vi "Test DQMH modules.vi"() -> ()   [LabVIEW 2018, in "Application.lvlib"]
uses:
  Application.lvlib
  eMIC response.ctl
  DRV stand.ctl
  type defs/HW config.ctl
  eMICs Cluster.ctl
  SubVIs/App state data.ctl
  SubVIs/Trigger cluster.ctl
  type defs/DMM all config cluster.ctl
  type defs/DMM config cluster.ctl
  SubVIs/FGV DRV data.ctl
  SubVIs/DUT data Mode.ctl
  Instrument Drivers/LV_driver_MBrelay/type defs/FGV enum.ctl
  SubVIs/Step data.ctl
  <vilib>/ErrorRing/Error Ring.xnode
  Switches Module/MB switches Module.lvlib
  MB 01 switches Module/MB 01 switches Module.lvlib
  DMM Module/DMM Module.lvlib
  v2_CE14/CE14_v2.lvlib
  Instrument Drivers/LV_driver_MBrelay/MB Relay.lvlib
panel:
  out "Name":string
  out "SAP ID":string
  out "Progress":string
  out "DRV stand":T1
  in  "Auto/Man":bool
  out "DC Measure Completed":bool
  in  "Test Channel 10":bool
  in  "Test Channel 9":bool
  in  "Test Channel 8":bool
  in  "Test Channel 7":bool
  in  "Test Channel 6":bool
  in  "Test Channel 5":bool
  in  "Test Channel 4":bool
  in  "Test Channel 3":bool
  in  "Test Channel 2":bool
  in  "Test Channel 1":bool
  in  "Shorted Circuits Test":bool
  out "CE14  Module did it":bool[](array[boolean])
  out "time elased(ms)":u32
  out "Inst. 9":bool
  in  "Exit":bool
  out "Inst. 8":bool
  out "Inst. 7":bool
  out "Inst. 6":bool
  out "Inst. 5":bool
  out "Inst. 4":bool
  out "Inst. 3":bool
  out "Inst. 2":bool
  out "Inst. 1":bool
  out "new Trigger?":bool
  out "last Trigger?":bool
  out "error out":errorcluster
  out "State log":string
  out "AC Measure  Completed":bool
  in  "Select CE14 eMIC Module Instance":i32(ring)=-1 items=["All"=-1, "1"=1, "2"=2, "3"=3, "4"=4, "5"=5, "6"=6]
  out "New board?":bool
  in  "Test":bool caption="Again"
  out "DRV 61":u32(colorbox)
  in  "Settings":bool
  in  "Again":bool
  out "DRV 60":u32(colorbox) caption="60"
  out "DRV 59":u32(colorbox) caption="59"
  out "DRV 58":u32(colorbox) caption="58"
  out "DRV 57":u32(colorbox) caption="57"
  out "DRV 56":u32(colorbox) caption="56"
  out "DRV 55":u32(colorbox) caption="55"
  out "DRV 54":u32(colorbox) caption="54"
  out "DRV 53":u32(colorbox) caption="53"
  out "DRV 52":u32(colorbox) caption="52"
  out "DRV 51":u32(colorbox) caption="51"
  out "DRV 50":u32(colorbox) caption="50"
  out "DRV 49":u32(colorbox) caption="49"
  out "DRV 48":u32(colorbox) caption="48"
  out "DRV 47":u32(colorbox) caption="47"
  out "DRV 46":u32(colorbox) caption="46"
  out "DRV 45":u32(colorbox) caption="45"
  out "DRV 44":u32(colorbox) caption="44"
  out "DRV 43":u32(colorbox) caption="43"
  out "DRV 42":u32(colorbox) caption="42"
  out "DRV 41":u32(colorbox) caption="41"
  out "DRV 40":u32(colorbox) caption="40"
  out "DRV 39":u32(colorbox) caption="39"
  out "DRV 38":u32(colorbox) caption="38"
  out "DRV 37":u32(colorbox) caption="37"
  out "DRV 36":u32(colorbox) caption="36"
  out "DRV 35":u32(colorbox) caption="35"
  out "DRV 34":u32(colorbox) caption="34"
  out "DRV 33":u32(colorbox) caption="33"
  out "DRV 32":u32(colorbox) caption="32"
  out "DRV 31":u32(colorbox) caption="31"
  out "DRV 30":u32(colorbox) caption="30"
  out "DRV 29":u32(colorbox) caption="29"
  out "DRV 28":u32(colorbox) caption="28"
  out "DRV 27":u32(colorbox) caption="27"
  out "DRV 26":u32(colorbox) caption="26"
  out "DRV 25":u32(colorbox) caption="25"
  out "DRV 24":u32(colorbox) caption="24"
  out "DRV 23":u32(colorbox) caption="23"
  out "DRV 22":u32(colorbox) caption="22"
  out "DRV 21":u32(colorbox) caption="21"
  out "DRV 20":u32(colorbox) caption="20"
  out "DRV 19":u32(colorbox)=4375612 caption="19"
  out "DRV 18":u32(colorbox) caption="18"
  out "DRV 17":u32(colorbox) caption="17"
  out "DRV 16":u32(colorbox) caption="16"
  out "DRV 15":u32(colorbox) caption="15"
  out "DRV 14":u32(colorbox) caption="14"
  out "DRV 13":u32(colorbox)=4375612 caption="13"
  out "DRV 12":u32(colorbox) caption="12"
  out "DRV 11":u32(colorbox) caption="11"
  out "DRV 10":u32(colorbox) caption="10"
  out "DRV 9":u32(colorbox) caption="9"
  out "DRV 8":u32(colorbox) caption="8"
  out "DRV 7":u32(colorbox)=4375612 caption="7"
  out "DRV 6":u32(colorbox) caption="6"
  out "DRV 5":u32(colorbox) caption="5"
  out "DRV 4":u32(colorbox) caption="4"
  out "DRV 3":u32(colorbox) caption="3"
  out "DRV 2":u32(colorbox) caption="2"
  out "DRV 1":u32(colorbox)=13224393 caption="1"
  out "version":string caption="Version"
  out "Module ID":i32
  in  "Tab Control":T2(tab)
  out "Short DRV":bool[][](array[boolean])
  in  "Mux 10-1":bool
  in  "mux 6-1":bool
  in  "Read Optos":bool
  in  "DMM select Current Input":bool
  in  "mux2-1(DMM I) encode":enum16{"DMM I (0.5)", "DMM I (12)"}(ring)
  in  "mux 6-1 data":T3(ring)
  in  "mux 10-1 data":T4(ring)
  out "trigger Value":bool
  in  "Read trigger":bool
  in  "Reset JIG":bool
  in  "eMIC":bool
  in  "DEMUX 1-10":bool
  in  "TurnON/OFF +5V":bool
  in  "5V Value":bool
  in  "demux1_10(x6)_encode":T5(ring)
  in  "eMIC 6 values":bool[](array[boolean])=[FALSE, FALSE, FALSE, FALSE, FALSE, FALSE]
  in  "config DMM input":bool
  in  "connect DMM":bool
  in  "DMM read dual value":bool
  in  "config DMM":bool
  in  "Detector Rate":u8(ring)=2 items=["SLOW", "MID", "FAST"]
  in  "DCI range":dbl=0.5
  in  "DCV range":dbl=1000.0
  out "DCV(Volts)":dbl
  out "DCI(mA)":dbl
  in  "request AC":bool
  in  "Open COM eMIC":bool
  in  "check connected":bool
  out "eMIC 1":T6
  out "eMIC 2":T6
  out "eMIC 3":T6
  out "eMIC 4":T6
  out "eMIC 5":T6
  out "eMIC 6":T6
  out "EMIC connected":bool[](array[boolean])
  out "AC switches Module":bool
  out "DC Measure Module":bool
  out "DC Switches Module":bool
  out "AC Measure Module":bool
  # "HV-60D: LED POWER DRIVER ON-LINE TESTER"
  # "60"
  # "6"
  # "12"
  # "18"
  # "24"
  # "30"
  # "36"
  # "42"
  # "48"
  # "54"
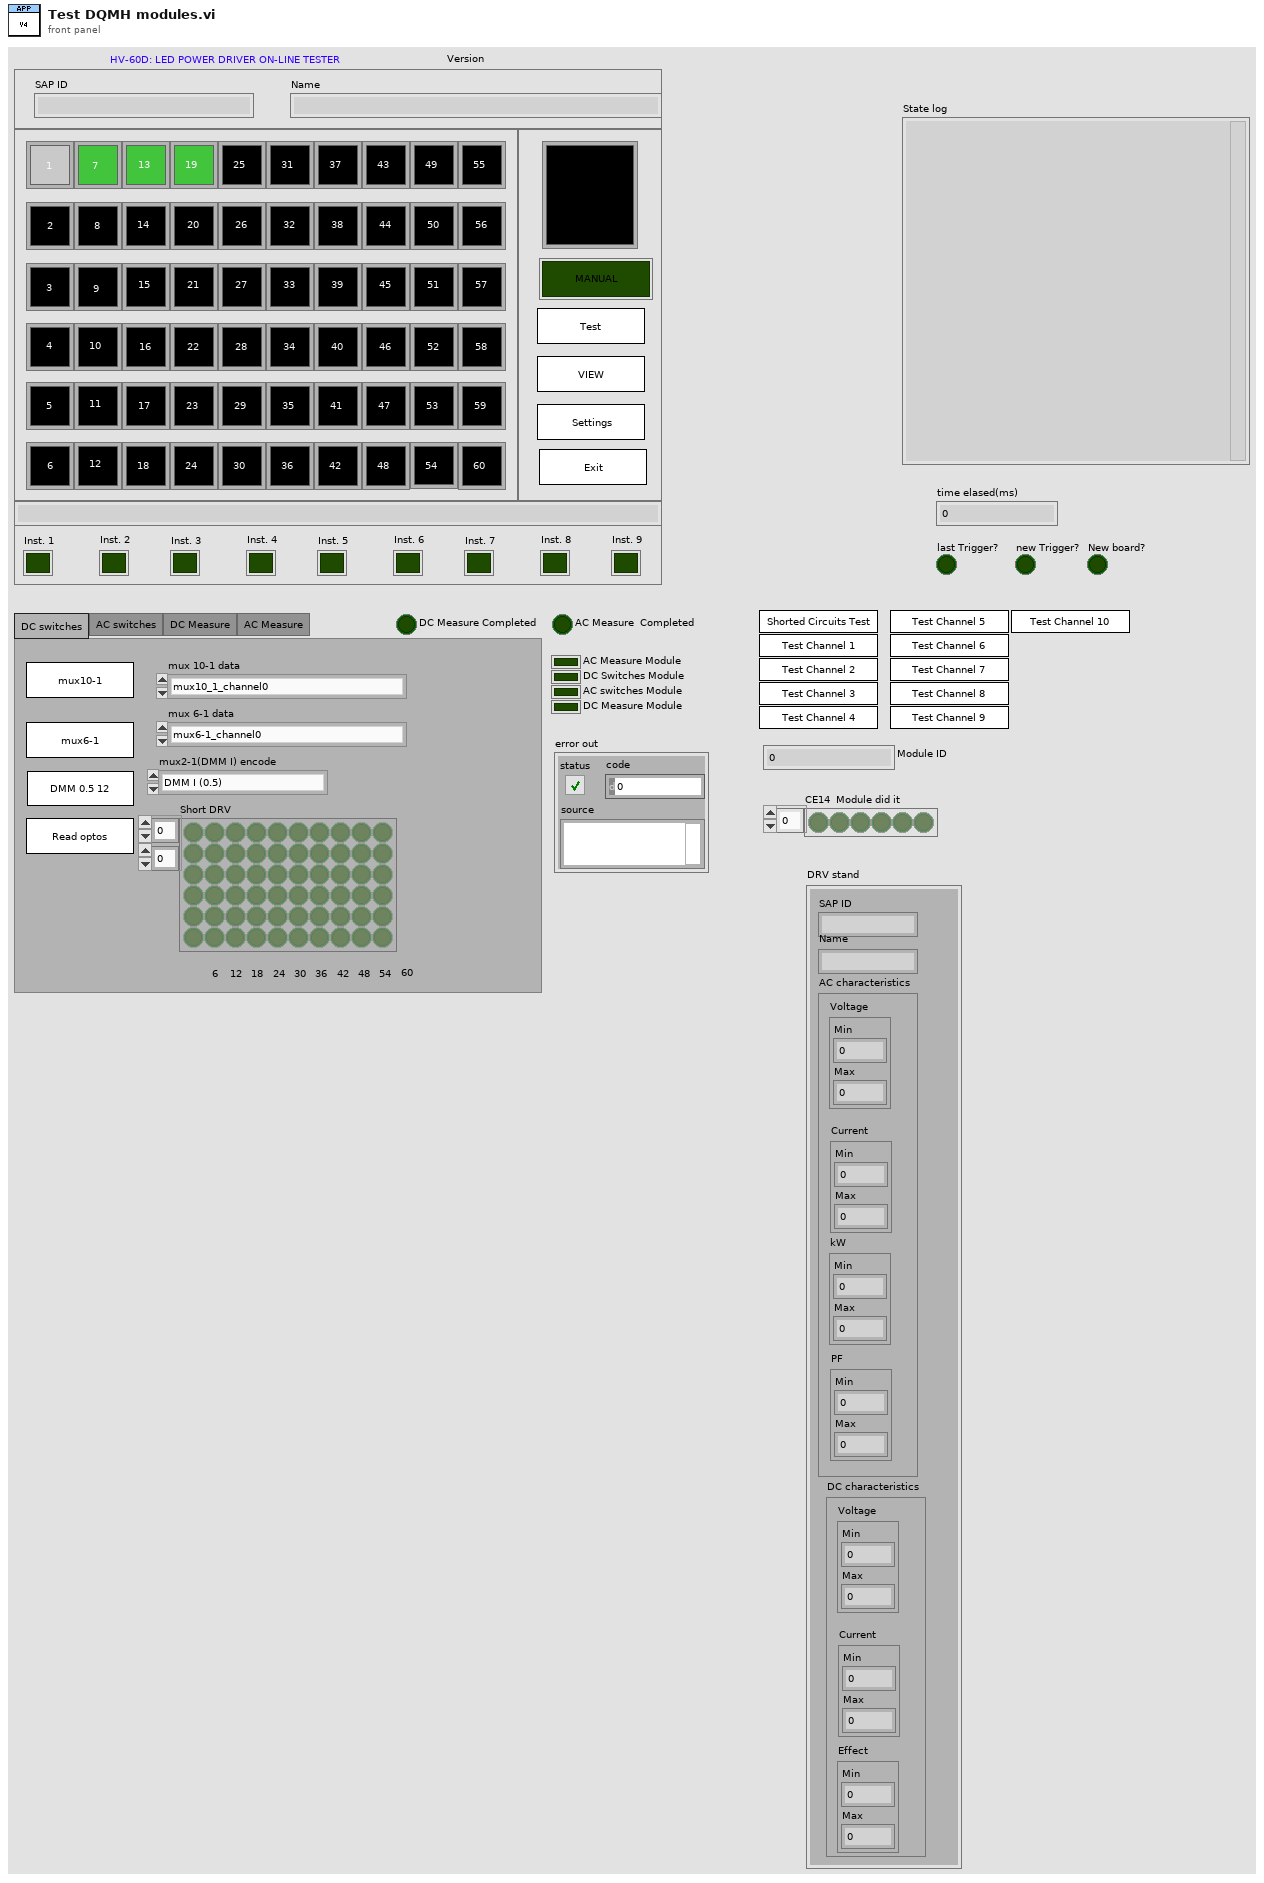
[diagram p1: front panel]
types:
  T1 = typedef "Application.lvlib/DRV stand.ctl" = cluster{"SAP ID":string, "Name":string, "AC characteristics":cluster{"Voltage":cluster{"Min":dbl, "Max":dbl}, "Current":cluster{"Min":dbl, "Max":dbl}, "kW":cluster{"Min":dbl, "Max":dbl}, "PF":cluster{"Min":dbl, "Max":dbl}}, "DC characteristics":cluster{"Voltage":cluster{"Min":dbl, "Max":dbl}, "Current":cluster{"Min":dbl, "Max":dbl}, "Effect":cluster{"Min":dbl, "Max":dbl}}}
  T2 = enum32{"DC switches", "AC switches", "DC Measure", "AC Measure"}
  T3 = enum16{"mux6-1_channel0", "mux6_1_channel1_0", "mux6_1_channel1_1", "mux6-1_channel1_2", "mux6_1_channel1_3", "mux6_1_channel2_0", "mux6_1_channel2_1", "mux6_1_channel2_2", "mux6_1_channel2_3", "mux6_1_channel3_0", "mux6_1_channel3_1", "mux6_1_channel3_2", "mux6_1_channel3_3", "mux6_1_channel4_0", "mux6_1_channel4_1", "mux6_1_channel4_2", "mux6_1_channel4_3", "mux6_1_channel5_0", "mux6_1_channel5_1", "mux6_1_channel5_2", "mux6_1_channel5_3", "mux6_1_channel6_0", "mux6_1_channel6_1", "mux6_1_channel6_2", "mux6_1_channel6_3"}
  T4 = enum16{"mux10_1_channel0", "mux10_1_channel1", "mux10_1_channel2", "mux10_1_channel3", "mux10_1_channel4", "mux10_1_channel5", "mux10_1_channel6", "mux10_1_channel7", "mux10_1_channel8", "mux10_1_channel9", "mux10_1_channel10"}
  T5 = enum16{"demux1_10_channel0", "demux1_10_channel1", "demux1_10_channel2", "demux1_10_channel3", "demux1_10_channel4", "demux1_10_channel5", "demux1_10_channel6", "demux1_10_channel7", "demux1_10_channel8", "demux1_10_channel9", "demux1_10_channel10"}
  T6 = typedef "Application.lvlib/eMIC response.ctl" = cluster{"ACV":dbl, "ACI":dbl, "pF":dbl, "kW":dbl, "Freq":dbl}
  T7 = typedef "Application.lvlib/eMICs Cluster.ctl" = cluster{"eMIC 1":T6, "eMIC 2":T6, "eMIC 3":T6, "eMIC 4":T6, "eMIC 5":T6, "eMIC 6":T6}
  T8 = typedef "Application.lvlib/HW config.ctl" = cluster{"DMM":string, "mux":string, "demux":string, "eMIC1":string, "eMIC2":string, "eMIC3":string, "eMIC4":string, "eMIC5":string, "eMIC6":string}
  T9 = typedef "Application.lvlib/Trigger cluster.ctl" = cluster{"new board?":bool, "new trigger":bool, "last trigger":bool}
  T10 = typedef "Application.lvlib/App state data.ctl" = cluster{"command":string, "command data":variant}
  T11 = typedef "CE14_v2.lvlib/Broadcast Events--cluster.ctl" = cluster{"Module Did Init":refnum<user-event>, "Status Updated":refnum<user-event>, "Error Reported":refnum<user-event>, "Module Did Stop":refnum<user-event>, "Update Module Execution Status":refnum<user-event>, "CE14 response data":refnum<user-event>}
  T12 = typedef "MB switches Module.lvlib/Broadcast Events--cluster.ctl" = cluster{"Module Did Init":refnum<user-event>, "Status Updated":refnum<user-event>, "Error Reported":refnum<user-event>, "Module Did Stop":refnum<user-event>, "Update Module Execution Status":refnum<user-event>}
  T13 = typedef "MB 01 switches Module.lvlib/Broadcast Events--cluster.ctl" = cluster{"Module Did Init":refnum<user-event>, "Status Updated":refnum<user-event>, "Error Reported":refnum<user-event>, "Module Did Stop":refnum<user-event>, "Update Module Execution Status":refnum<user-event>}
  T14 = typedef "DMM Module.lvlib/Broadcast Events--cluster.ctl" = cluster{"Module Did Init":refnum<user-event>, "Status Updated":refnum<user-event>, "Error Reported":refnum<user-event>, "Module Did Stop":refnum<user-event>, "Update Module Execution Status":refnum<user-event>}
  T15 = enum32{"Invalid", "Standard", "Closed", "Hidden", "Minimized", "Maximized"}
  T16 = typedef "Application.lvlib/DMM all config cluster.ctl" = cluster{"DMM config cluster":T17, "mux2-1(DMM I) encode":enum16{"DMM I (0.5)", "DMM I (12)"}}
  T17 = typedef "Application.lvlib/DMM config cluster.ctl" = cluster{"DCV range":dbl, "DCI range":dbl, "Detector Rate":u8}
  T18 = typedef "Application.lvlib/DUT data Mode.ctl" = enum16{"range Limit", "Short Circuits", "AC parameter", "DC parameter"}
  T19 = typedef "Application.lvlib/FGV DRV data.ctl" = enum16{"Init", "Write", "Read", "Process"}
  T20 = typedef "MB Relay.lvlib/FGV enum.ctl" = enum16{"Write", "Init FGV", "Read", "All OFF", "All ON"}
  T21 = typedef "CE14_eMIC.lvlib/CE14.data.ctl" = cluster{"string":string, "float":dbl, "Name":string}
  T22 = typedef "Application.lvlib/DRV cluster 2.ctl" = cluster{"Shorted Circuit":bool, "AC voltage(volts)":dbl, "AC Current (mA)":dbl, "AC kW (W)":dbl, "AC pF ":dbl, "DC Voltage (Volts)":dbl, "DC Current (mA)":dbl, "DC kW (W)":dbl, "DRV Fail/Pass (T)":bool}
  T23 = typedef "Application.lvlib/Step data.ctl" = cluster{"command":string, "Data":variant}
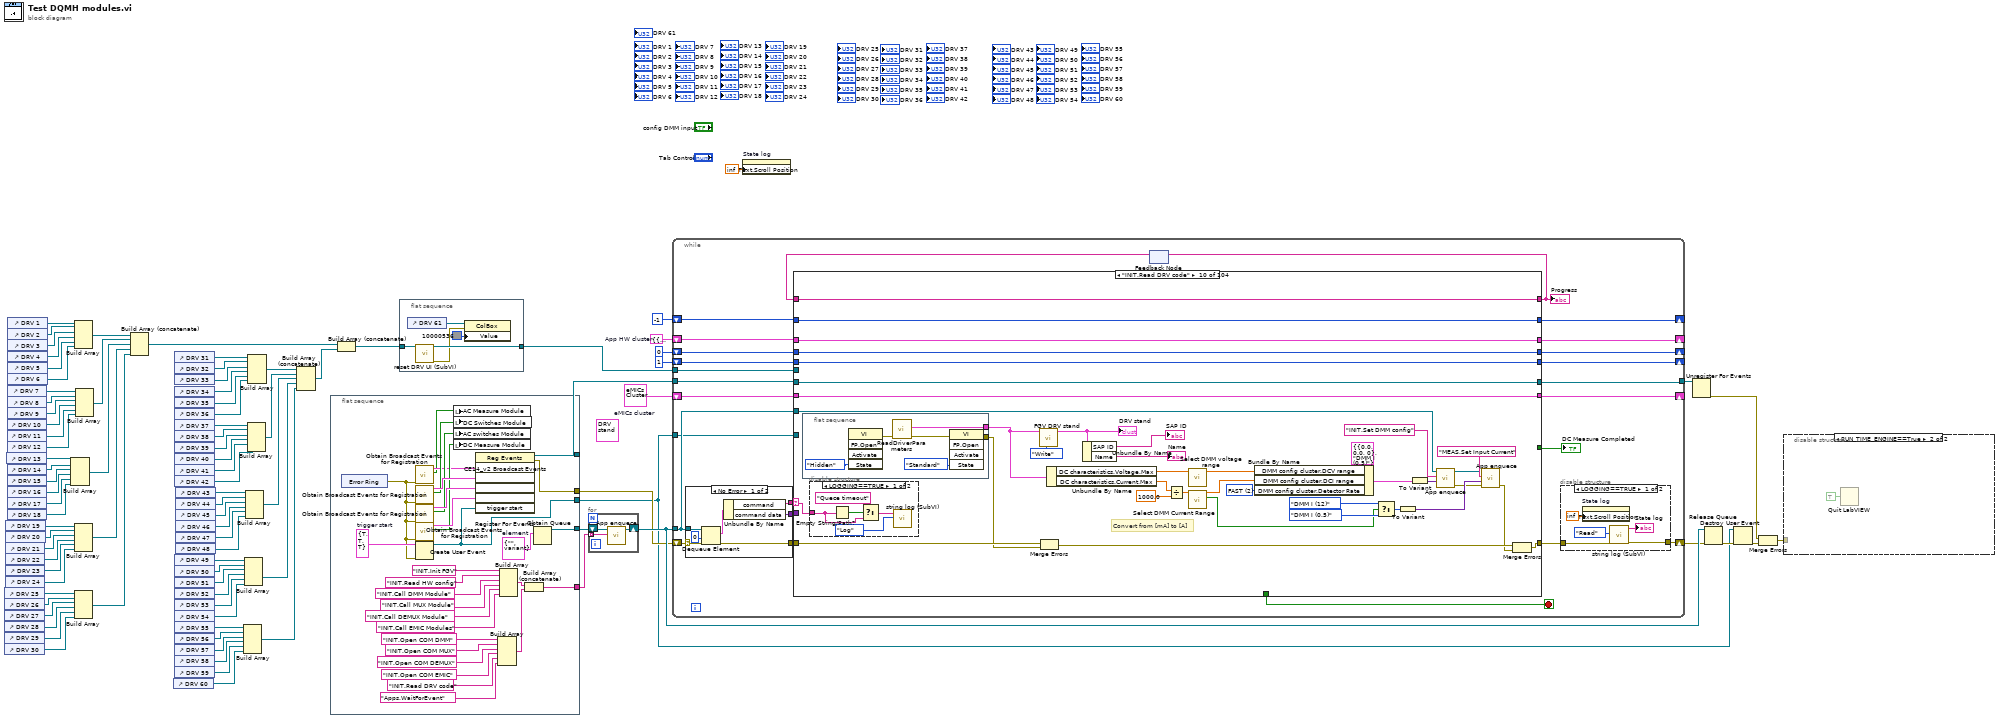
[diagram p0: block diagram]
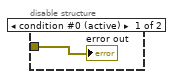
[diagram p2: hidden frame]
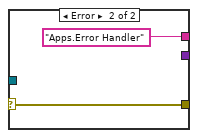
[diagram p4: hidden frame]
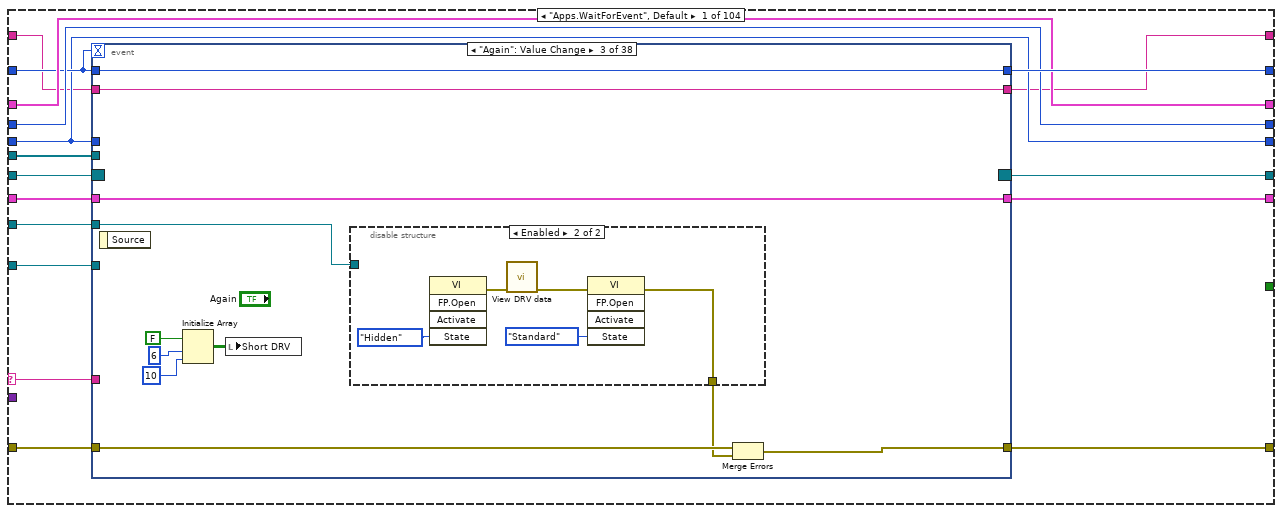
[diagram p5: hidden frame]
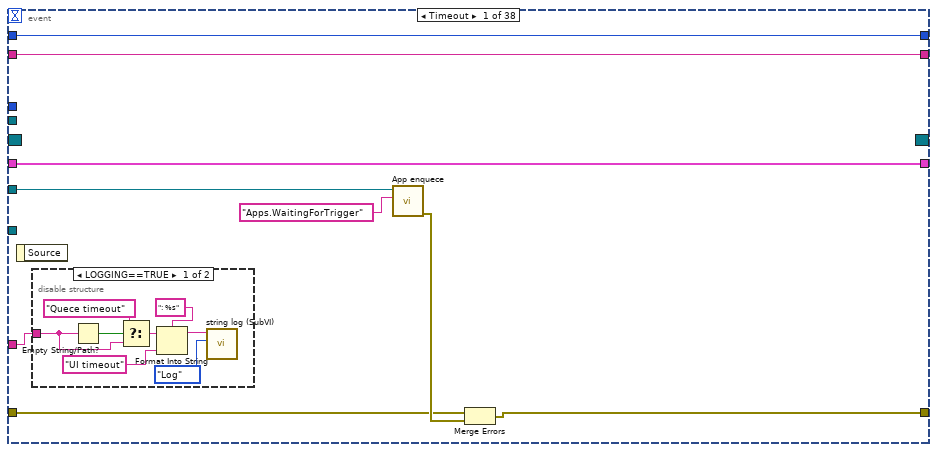
[diagram p6: hidden frame]
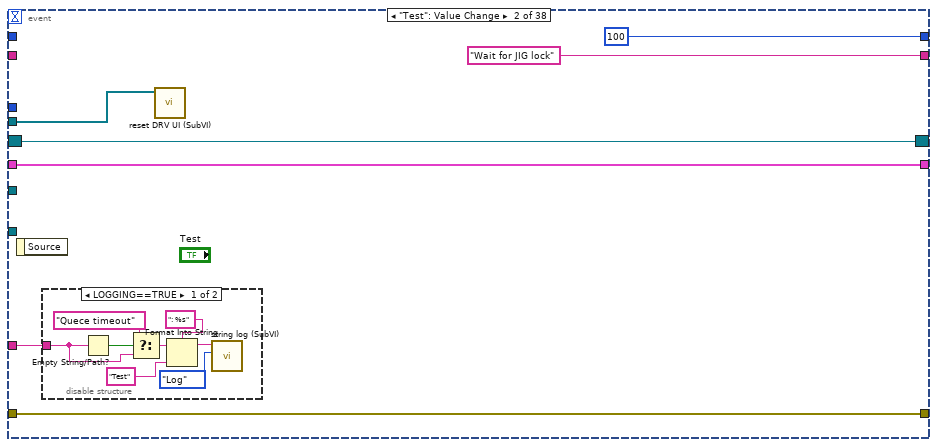
[diagram p8: hidden frame]
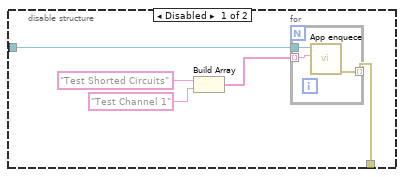
[diagram p10: hidden frame]
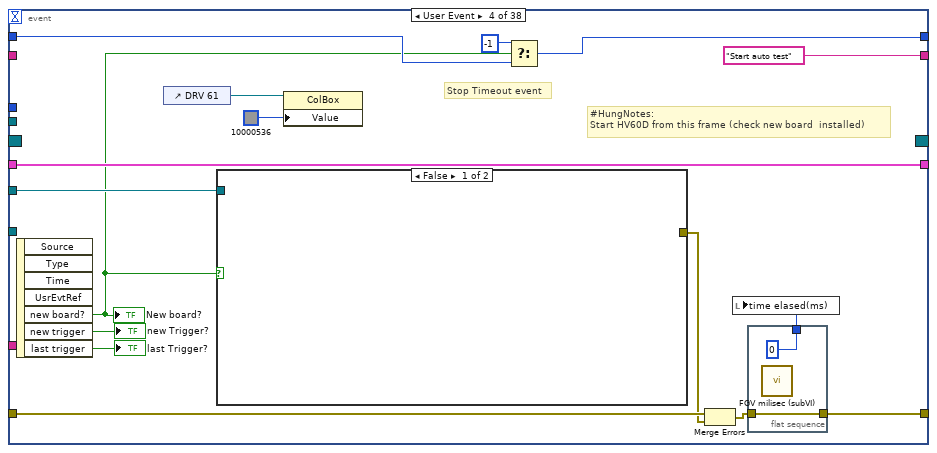
[diagram p11: hidden frame]
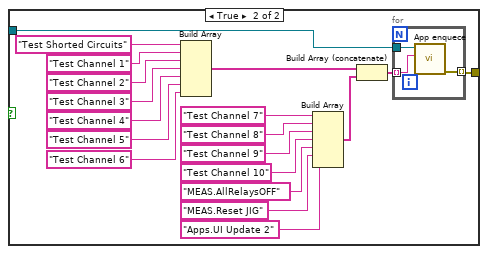
[diagram p12: hidden frame]
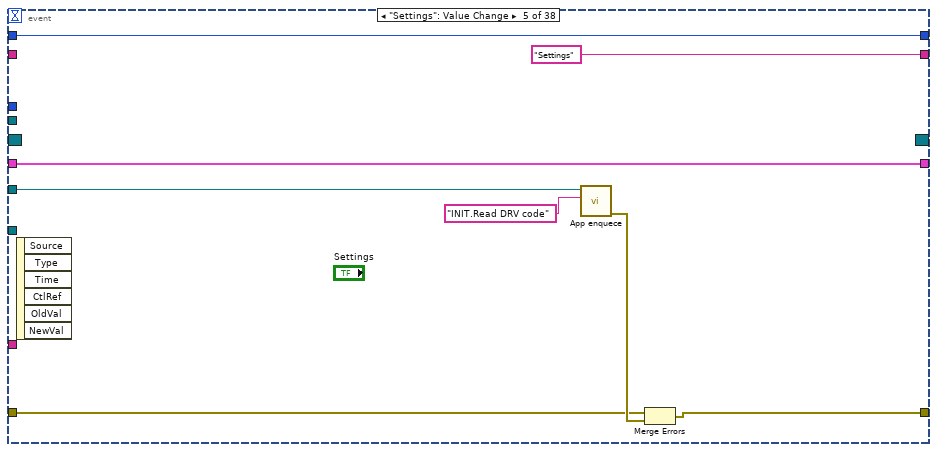
[diagram p13: hidden frame]
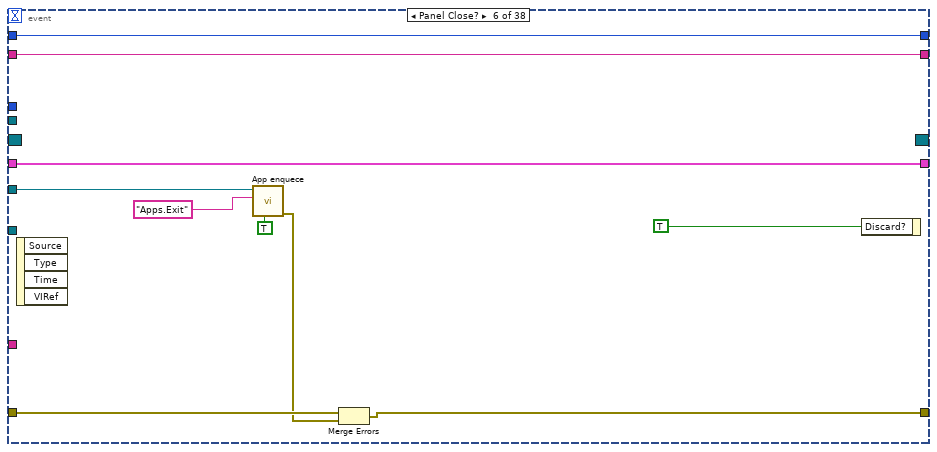
[diagram p14: hidden frame]
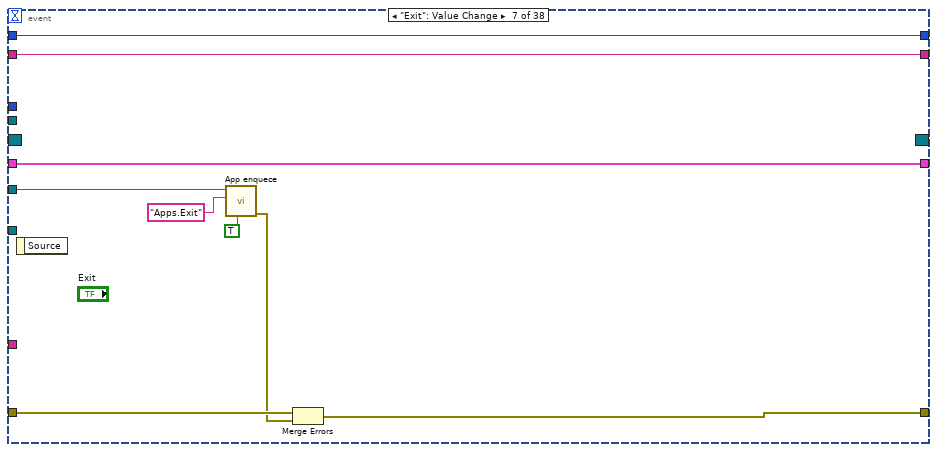
[diagram p15: hidden frame]
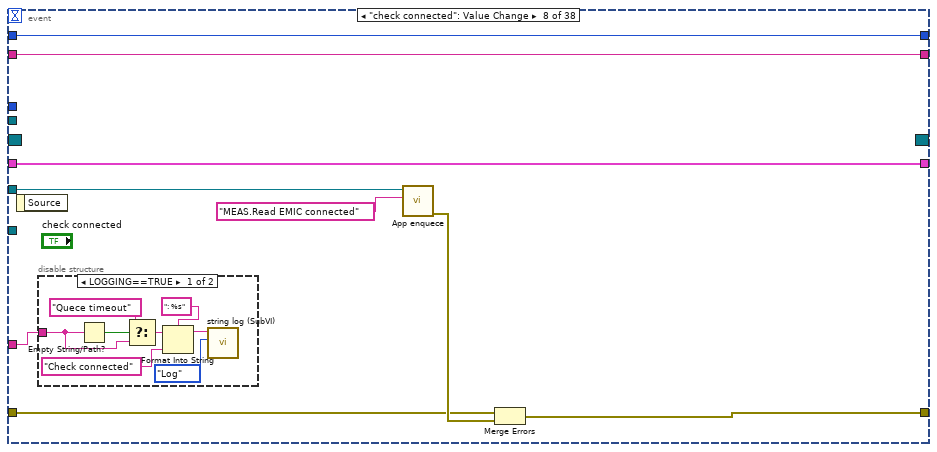
[diagram p16: hidden frame]
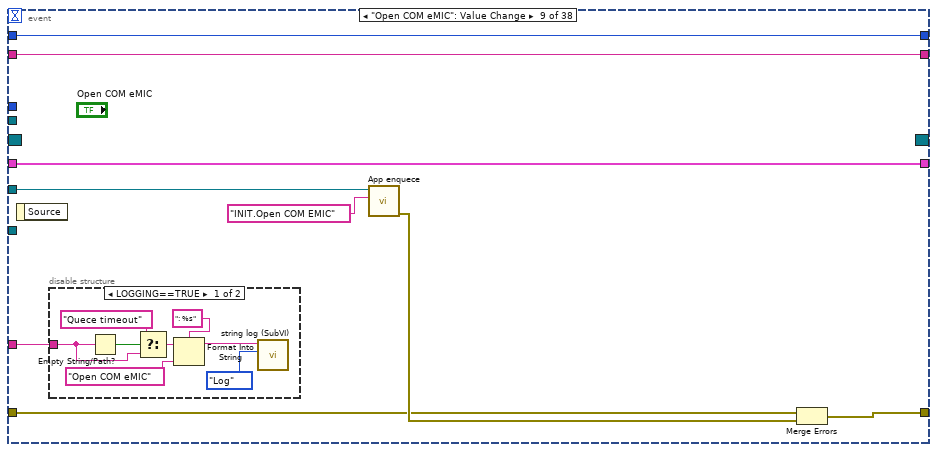
[diagram p18: hidden frame]
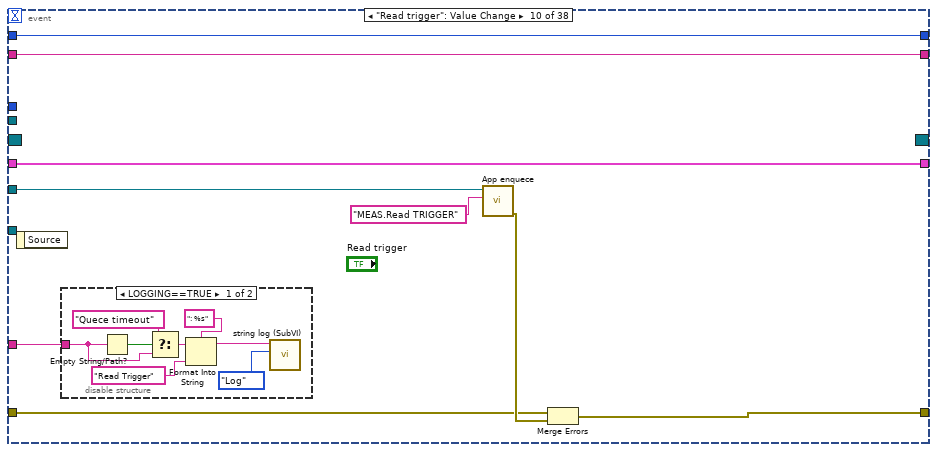
[diagram p20: hidden frame]
diagram:
  (unwired) T1 {"SAP ID"="", "Name"="", "AC characteristics"={"Voltage"={"Min"=0.0, "Max"=0.0}, "Current"={"Min"=0.0, "Max"=0.0}, "kW"={"Min"=0.0, "Max"=0.0}, "PF"={"Min"=0.0, "Max"=0.0}}, "DC characteristics"={"Voltage"={"Min"=0.0, "Max"=0.0}, "Current"={"Min"=0.0, "Max"=0.0}, "Effect"={"Min"=0.0, "Max"=0.0}}} ("DRV stand")
  w84 = T7 {"eMIC 1"={"ACV"=0.0, "ACI"=0.0, "pF"=0.0, "kW"=0.0, "Freq"=0.0}, "eMIC 2"={"ACV"=0.0, "ACI"=0.0, "pF"=0.0, "kW"=0.0, "Freq"=0.0}, "eMIC 3"={"ACV"=0.0, "ACI"=0.0, "pF"=0.0, "kW"=0.0, "Freq"=0.0}, "eMIC 4"={"ACV"=0.0, "ACI"=0.0, "pF"=0.0, "kW"=0.0, "Freq"=0.0}, "eMIC 5"={"ACV"=0.0, "ACI"=0.0, "pF"=0.0, "kW"=0.0, "Freq"=0.0}, "eMIC 6"={"ACV"=0.0, "ACI"=0.0, "pF"=0.0, "kW"=0.0, "Freq"=0.0}}  # eMICs cluster
  w89 = cluster{"HW config 2":T8} {"HW config 2"={"DMM"="COM15", "mux"="COM11", "demux"="COM16", "eMIC1"="COM13", "eMIC2"="COM6", "eMIC3"="COM9", "eMIC4"="COM10", "eMIC5"="COM12", "eMIC6"="COM11"}}  # App HW cluster
  n1 = control-ref of="DRV 25"() -> (w54:refnum<vi>)
  n2 = control-ref of="DRV 26"() -> (w55:refnum<vi>)
  n3 = control-ref of="DRV 27"() -> (w56:refnum<vi>)
  n4 = control-ref of="DRV 28"() -> (w57:refnum<vi>)
  n5 = control-ref of="DRV 29"() -> (w58:refnum<vi>)
  n6 = control-ref of="DRV 30"() -> (w59:refnum<vi>)
  n7 = control-ref of="DRV 21"() -> (w63:refnum<vi>)
  n8 = control-ref of="DRV 22"() -> (w62:refnum<vi>)
  n9 = control-ref of="DRV 23"() -> (w61:refnum<vi>)
  n10 = control-ref of="DRV 24"() -> (w60:refnum<vi>)
  n11 = control-ref of="DRV 19"() -> (w65:refnum<vi>)
  n12 = control-ref of="DRV 20"() -> (w64:refnum<vi>)
  n13 = control-ref of="DRV 13"() -> (w71:refnum<vi>)
  n14 = control-ref of="DRV 7"() -> (w77:refnum<vi>)
  n15 = control-ref of="DRV 8"() -> (w76:refnum<vi>)
  n16 = control-ref of="DRV 9"() -> (w75:refnum<vi>)
  n17 = control-ref of="DRV 10"() -> (w74:refnum<vi>)
  n18 = control-ref of="DRV 11"() -> (w73:refnum<vi>)
  n19 = control-ref of="DRV 12"() -> (w72:refnum<vi>)
  n20 = control-ref of="DRV 14"() -> (w70:refnum<vi>)
  n21 = control-ref of="DRV 15"() -> (w69:refnum<vi>)
  n22 = control-ref of="DRV 16"() -> (w68:refnum<vi>)
  n23 = control-ref of="DRV 17"() -> (w67:refnum<vi>)
  n24 = control-ref of="DRV 18"() -> (w66:refnum<vi>)
  n25 = control-ref of="DRV 1"() -> (w83:refnum<vi>)
  n26 = control-ref of="DRV 2"() -> (w82:refnum<vi>)
  n27 = control-ref of="DRV 3"() -> (w81:refnum<vi>)
  n28 = control-ref of="DRV 4"() -> (w80:refnum<vi>)
  n29 = control-ref of="DRV 5"() -> (w79:refnum<vi>)
  n30 = control-ref of="DRV 6"() -> (w78:refnum<vi>)
  n31 = Build Array(w71, w70, w69, w68, w67, w66) -> (w51:refnum<vi>[])
  n32 = Build Array(w83, w82, w81, w80, w79, w78) -> (w53:refnum<vi>[])
  n33 = Build Array(w65, w64, w63, w62, w61, w60) -> (w50:refnum<vi>[])
  n34 = Build Array(w54, w55, w56, w57, w58, w59) -> (w49:refnum<vi>[])
  n35 = Build Array(w77, w76, w75, w74, w73, w72) -> (w52:refnum<vi>[])
  n36 = Build Array (concatenate)(w53, w52, w51, w50, w49) -> (w13:refnum<vi>[])
  n37 = control-ref of="DRV 60"() -> (w24:refnum<vi>)
  n38 = control-ref of="DRV 55"() -> (w19:refnum<vi>)
  n39 = control-ref of="DRV 56"() -> (w20:refnum<vi>)
  n40 = control-ref of="DRV 57"() -> (w21:refnum<vi>)
  n41 = control-ref of="DRV 58"() -> (w22:refnum<vi>)
  n42 = control-ref of="DRV 59"() -> (w23:refnum<vi>)
  n43 = control-ref of="DRV 31"() -> (w43:refnum<vi>)
  n44 = control-ref of="DRV 32"() -> (w44:refnum<vi>)
  n45 = control-ref of="DRV 33"() -> (w45:refnum<vi>)
  n46 = control-ref of="DRV 34"() -> (w46:refnum<vi>)
  n47 = control-ref of="DRV 35"() -> (w47:refnum<vi>)
  n48 = control-ref of="DRV 36"() -> (w48:refnum<vi>)
  n49 = control-ref of="DRV 37"() -> (w42:refnum<vi>)
  n50 = control-ref of="DRV 38"() -> (w41:refnum<vi>)
  n51 = control-ref of="DRV 39"() -> (w40:refnum<vi>)
  n52 = control-ref of="DRV 40"() -> (w39:refnum<vi>)
  n53 = control-ref of="DRV 41"() -> (w38:refnum<vi>)
  n54 = control-ref of="DRV 42"() -> (w37:refnum<vi>)
  n55 = control-ref of="DRV 49"() -> (w30:refnum<vi>)
  n56 = control-ref of="DRV 50"() -> (w29:refnum<vi>)
  n57 = control-ref of="DRV 51"() -> (w28:refnum<vi>)
  n58 = control-ref of="DRV 52"() -> (w27:refnum<vi>)
  n59 = control-ref of="DRV 53"() -> (w26:refnum<vi>)
  n60 = control-ref of="DRV 54"() -> (w25:refnum<vi>)
  n61 = control-ref of="DRV 43"() -> (w31:refnum<vi>)
  n62 = control-ref of="DRV 44"() -> (w32:refnum<vi>)
  n63 = control-ref of="DRV 45"() -> (w33:refnum<vi>)
  n64 = control-ref of="DRV 46"() -> (w34:refnum<vi>)
  n65 = control-ref of="DRV 47"() -> (w35:refnum<vi>)
  n66 = control-ref of="DRV 48"() -> (w36:refnum<vi>)
  n67 = Build Array(w19, w20, w21, w22, w23, w24) -> (w14:refnum<vi>[])
  n68 = Build Array(w30, w29, w28, w27, w26, w25) -> (w15:refnum<vi>[])
  n69 = Build Array(w31, w32, w33, w34, w35, w36) -> (w16:refnum<vi>[])
  n70 = Build Array(w42, w41, w40, w39, w38, w37) -> (w17:refnum<vi>[])
  n71 = Build Array(w43, w44, w45, w46, w47, w48) -> (w18:refnum<vi>[])
  n72 = Build Array (concatenate)(w18, w17, w16, w15, w14) -> (w12:refnum<vi>[])
  n73 = flat-sequence {
    tunnel: [w116] -> w91
    tunnel: [w115] -> w88
    tunnel: [w114] -> w87
    tunnel: [w113] -> w11
    tunnel: [w108] -> w3
    frame #0 {
      w109 = T9 {"new board?"=TRUE, "new trigger"=TRUE, "last trigger"=TRUE}  # trigger start
      w110 = T10 {"command"="", "command data"=variant}  # element
      n74 = xnode "Error Ring"() -> ("error out"=w107:errorcluster)
      n75 = call "Obtain Broadcast Events for Registration.vi"("error in (no error)"=w107) -> ("Already running?"=w111:bool, "CE14_v2 Broadcast Events"=w112:T11)  [unwired: 8 in, 1 out]
      n76 = call "Obtain Broadcast Events for Registration.vi"("error in (no error)"=w107) -> ("Already running?"=w119:bool, "Switches Module Broadcast Events"=w122:T12)  [unwired: 8 in, 1 out]
      n77 = call "Obtain Broadcast Events for Registration.vi"("error in (no error)"=w107) -> ("Already running?"=w118:bool, "MB 01 switches Module Broadcast Events"=w121:T13)  [unwired: 8 in, 1 out]
      n78 = call "Obtain Broadcast Events for Registration.vi"("error in (no error)"=w107) -> ("Already running?"=w117:bool, "DMM Module Broadcast Events"=w120:T14)  [unwired: 8 in, 1 out]
      n79 = Create User Event(user event datatype=w109, error in=w107) -> (user event=w108:refnum<user-event>)  [unwired: 1 out]
      n80 = local write "AC Measure Module"(w111) -> ()
      n81 = local write "DC Switches Module"(w119) -> ()
      n82 = local write "AC switches Module"(w118) -> ()
      n83 = local write "DC Measure Module"(w117) -> ()
      n84 = register-events(w112, w122, w121, w120, w108) -> (reference out=w116:refnum<event-registration>, error out=w113:errorcluster)  [unwired: 2 in]
      n85 = Build Array("INIT.Open COM DMM", "INIT.Open COM MUX", "INIT.Open COM DEMUX", "INIT.Open COM EMIC", "INIT.Read DRV code", "Apps.WaitForEvent") -> (w104:string[])
      n86 = Build Array("INIT.Init FGV", "INIT.Read HW config", "INIT.Call DMM Module", "INIT.Call MUX Module", "INIT.Call DEMUX Module", "INIT.Call EMIC Modules") -> (w105:string[])
      n87 = Build Array (concatenate)(w105, w104) -> (w114:string[])
      n88 = Obtain Queue(element data type=w110) -> (queue out=w115:refnum<queue>)  [unwired: 4 in, 2 out]
    }
  }
  n89 = Build Array (concatenate)(w13, w12) -> (w10:refnum<vi>[])
  n90 = flat-sequence {
    tunnel: w10 -> [w128]
    tunnel: [w127] -> w9
    frame #0 {
      n91 = control-ref of="DRV 61"() -> (w124:refnum<vi>)
      n92 = call "reset DRV UI (SubVI).vi"("Ref  in"=w128) -> ("error out"=w125:errorcluster, "Ref out"=w127:refnum<vi>[])  [unwired: 9 in]
      n93 = property class="ColBox"(reference=w124, error in=w125, "Value"=u32 10000536 ("DRV 1")) -> ()  [unwired: 2 out]
    }
  }
  n94 = for {
    tunnel: w87 -> [w131] mode=indexing
    shift-right: [w129] -> w86
    shift-left: w88 -> [w130]
    n95 = call "App enquece.vi"("command"=w131, "queue in"=w130) -> ("Queue out"=w129:refnum<queue>)  [unwired: 8 in, 1 out]
  }
  n96 = while {
    shift-right: [w134] -> w85
    shift-left: w11 -> [w156]
    shift-right: [w154] -> _
    shift-left: -1 -> [w153]
    tunnel: w91 -> [w152]
    tunnel: [w151] -> w90
    shift-right: [w149] -> _
    shift-left: w89 -> [w150]
    tunnel: w86 -> [w138]
    shift-right: [w147] -> _
    shift-left: w84 -> [w146]
    tunnel: w9 -> [w144]
    shift-right: [w143] -> _
    shift-left: 1 ("DUT channel (1-11)") -> [w142]
    shift-right: [w141] -> _
    shift-left: 0 ("DUT index(0-59)") -> [w140]
    tunnel: w3 -> [w137]
    stop <- w145 stop-if-true
    n97 = case shown="No Error" w156 {
      selector: w156 -> [w168 w169]
      tunnel: [w166 "Apps.Error Handler"] -> w139
      tunnel: [w167 w169] -> w155
      tunnel: [w165 _] -> w148
      tunnel: w138 -> [w164 _]
      frame No Error {
        n98 = Dequeue Element(queue=w164, timeout in ms (-1)=0, error in (no error)=w168) -> (element=w163:T10, error out=w167:errorcluster)  [unwired: 2 out]
        n99 = Unbundle By Name(w163) -> ("command"=w166:string, "command data"=w165:variant)
      }
      frame Error {
      }
    }
    n100 = feedback #1() -> (w132:string)  [unwired: 1 in]
    n101 = case shown="\"INIT.Read DRV code\"" w139 {
      selector: w139 -> [w175 _ w982 w1010 w1035 w1058 w1081 _ w1120 w1196 w1217 w1240 w1263 w1288 w1322 w1341 w1360 w1379 w1408 w1433 w1457 w1502 w1523 w1547 w1582 w1604 w1629 w1660 w1701 w1723 w1758 w1793 w1827 w1882 w1953 w2022 w2092 w2162 w2232 w2302 w2372 w2443 w2514 w2566 w2603 w2641 w2679 w2717 w2755 w2793 w2831 w2869 w2907 w2945 w2983 w3021 w3059 w3097 w3135 w3173 w3211 w3249 w3287 w3325 w3363 w3401 w3439 w3477 w3515 w3553 w3591 w3629 w3667 w3705 w3743 w3781 w3819 w3857 w3895 w3933 w3971 w4009 w4047 w4085 w4123 w4161 w4199 w4237 w4275 w4313 w4351 w4389 w4427 w4465 w4503 w4541 w4579 w4617 w4655 w4693 w4731 w4769 w4807 _]
      tunnel: w155 -> [w182 w970 w983 w1013 w1049 w1066 w1095 w1117 w1133 w1197 w1218 w1241 w1264 w1289 w1323 w1342 w1361 w1380 w1411 w1434 w1458 w1505 w1526 w1546 w1584 w1605 w1630 w1661 w1705 w1726 w1761 w1794 w1821 w1884 w1955 w2024 w2094 w2164 w2234 w2304 w2374 w2445 w2516 w2579 w2617 w2655 w2693 w2731 w2769 w2807 w2845 w2883 w2921 w2959 w2997 w3035 w3073 w3111 w3149 w3187 w3225 w3263 w3301 w3339 w3377 w3415 w3453 w3491 w3529 w3567 w3605 w3643 w3681 w3719 w3757 w3795 w3833 w3871 w3909 w3947 w3985 w4023 w4061 w4099 w4137 w4175 w4213 w4251 w4289 w4327 w4365 w4403 w4441 w4479 w4517 w4555 w4593 w4631 w4669 w4707 w4745 w4783 w4821 w4846]
      tunnel: [w183 w971 w984 w1014 w1033 w1067 w1083 w1105 w1124 w1183 w1219 w1242 w1265 w1287 w1321 w1340 w1359 w1378 w1398 w1432 w1460 w1504 w1525 w1549 w1583 w1609 w1632 w1664 w1703 w1725 w1759 w1792 w1825 w1885 w1956 w2025 w2095 w2165 w2235 w2305 w2375 w2446 w2517 w2580 w2618 w2656 w2694 w2732 w2770 w2808 w2846 w2884 w2922 w2960 w2998 w3036 w3074 w3112 w3150 w3188 w3226 w3264 w3302 w3340 w3378 w3416 w3454 w3492 w3530 w3568 w3606 w3644 w3682 w3720 w3758 w3796 w3834 w3872 w3910 w3948 w3986 w4024 w4062 w4100 w4138 w4176 w4214 w4252 w4290 w4328 w4366 w4404 w4442 w4480 w4518 w4556 w4594 w4632 w4670 w4708 w4746 w4784 w4822 w4846] -> w135
      tunnel: [_ _ _ _ _ TRUE _ _ _ _ _ _ _ _ _ _ _ _ _ _ _ _ _ _ _ _ _ _ _ _ _ _ _ _ _ _ _ _ _ _ _ _ _ _ _ _ _ _ _ _ _ _ _ _ _ _ _ _ _ _ _ _ _ _ _ _ _ _ _ _ _ _ _ _ _ _ _ _ _ _ _ _ _ _ _ _ _ _ _ _ _ _ _ _ _ _ _ _ _ _ _ _ _ _] -> w145
      tunnel: [w187 w980 w993 w1017 w1048 w1073 w1094 w1116 w1132 w1204 w1233 w1256 w1279 w1303 w1330 w1349 w1368 w1388 w1417 w1448 w1468 w1493 w1536 w1555 w1591 w1616 w1640 w1683 w1712 w1734 w1769 w1800 w1846 w1904 w1974 w2044 w2114 w2184 w2254 w2324 w2394 w2464 w2535 w2585 w2623 w2661 w2699 w2737 w2775 w2813 w2851 w2889 w2927 w2965 w3003 w3041 w3079 w3117 w3155 w3193 w3231 w3269 w3307 w3345 w3383 w3421 w3459 w3497 w3535 w3573 w3611 w3649 w3687 w3725 w3763 w3801 w3839 w3877 w3915 w3953 w3991 w4029 w4067 w4105 w4143 w4181 w4219 w4257 w4295 w4333 w4371 w4409 w4447 w4485 w4523 w4561 w4599 w4637 w4675 w4713 w4751 w4789 w4827 w4845] -> w154
      tunnel: w153 -> [w174 w980 w993 w1017 w1048 w1073 w1094 w1116 w1132 w1204 w1233 w1256 w1279 w1303 w1330 w1349 w1368 w1388 w1417 w1448 w1468 w1492 w1536 w1555 w1591 w1616 w1640 w1683 w1712 w1734 w1769 w1800 w1846 w1904 w1974 w2044 w2114 w2184 w2254 w2324 w2394 w2464 w2535 w2585 w2623 w2661 w2699 w2737 w2775 w2813 w2851 w2889 w2927 w2965 w3003 w3041 w3079 w3117 w3155 w3193 w3231 w3269 w3307 w3345 w3383 w3421 w3459 w3497 w3535 w3573 w3611 w3649 w3687 w3725 w3763 w3801 w3839 w3877 w3915 w3953 w3991 w4029 w4067 w4105 w4143 w4181 w4219 w4257 w4295 w4333 w4371 w4409 w4447 w4485 w4523 w4561 w4599 w4637 w4675 w4713 w4751 w4789 w4827 w4845]
      tunnel: w152 -> [w186 w979 w992 w1016 w1047 w1072 w1093 w1115 w1131 w1203 w1231 w1254 w1277 w1296 w1329 w1348 w1367 w1387 w1416 w1447 w1467 w1511 w1535 w1554 w1590 w1615 w1639 w1682 w1711 w1733 w1768 w1799 w1845 w1903 w1973 w2043 w2113 w2183 w2253 w2323 w2393 w2423 w2534 w2584 w2622 w2660 w2698 w2736 w2774 w2812 w2850 w2888 w2926 w2964 w3002 w3040 w3078 w3116 w3154 w3192 w3230 w3268 w3306 w3344 w3382 w3420 w3458 w3496 w3534 w3572 w3610 w3648 w3686 w3724 w3762 w3800 w3838 w3876 w3914 w3952 w3990 w4028 w4066 w4104 w4142 w4180 w4218 w4256 w4294 w4332 w4370 w4408 w4446 w4484 w4522 w4560 w4598 w4636 w4674 w4712 w4750 w4788 w4826 w4844]
      tunnel: [w185 w979 w992 w1016 w1047 w1072 w1093 w1115 w1131 w1203 w1232 w1255 w1278 w1294 w1329 w1348 w1367 w1387 w1416 w1447 w1467 w1511 w1535 w1554 w1590 w1615 w1639 w1682 w1711 w1733 w1768 w1799 w1845 w1903 w1973 w2043 w2113 w2183 w2253 w2323 w2393 w2423 w2534 w2584 w2622 w2660 w2698 w2736 w2774 w2812 w2850 w2888 w2926 w2964 w3002 w3040 w3078 w3116 w3154 w3192 w3230 w3268 w3306 w3344 w3382 w3420 w3458 w3496 w3534 w3572 w3610 w3648 w3686 w3724 w3762 w3800 w3838 w3876 w3914 w3952 w3990 w4028 w4066 w4104 w4142 w4180 w4218 w4256 w4294 w4332 w4370 w4408 w4446 w4484 w4522 w4560 w4598 w4636 w4674 w4712 w4750 w4788 w4826 w4844] -> w151
      tunnel: w150 -> [w184 w978 w991 w1015 w1046 w1071 w1092 w1114 w1130 w1202 w1228 w1252 w1274 w1295 w1328 w1345 w1366 w1386 w1415 w1446 w1466 w1510 w1534 w1553 w1589 w1614 w1638 w1681 w1710 w1732 w1767 w1798 w1844 w1902 w1972 w2042 w2112 w2182 w2252 w2322 w2392 w2463 w2533 w2583 w2621 w2659 w2697 w2735 w2773 w2811 w2849 w2887 w2925 w2963 w3001 w3039 w3077 w3115 w3153 w3191 w3229 w3267 w3305 w3343 w3381 w3419 w3457 w3495 w3533 w3571 w3609 w3647 w3685 w3723 w3761 w3799 w3837 w3875 w3913 w3951 w3989 w4027 w4065 w4103 w4141 w4179 w4217 w4255 w4293 w4331 w4369 w4407 w4445 w4483 w4521 w4559 w4597 w4635 w4673 w4711 w4749 w4787 w4825 w4843]
      tunnel: [w184 w978 w991 w1015 w1046 w1071 w1092 w1114 w1128 w1202 w1228 w1252 w1274 w1295 w1328 w1345 w1366 w1386 w1415 w1446 w1466 w1510 w1534 w1553 w1589 w1614 w1638 w1681 w1710 w1732 w1767 w1798 w1844 w1902 w1972 w2042 w2112 w2182 w2252 w2322 w2392 w2463 w2533 w2583 w2621 w2659 w2697 w2735 w2773 w2811 w2849 w2887 w2925 w2963 w3001 w3039 w3077 w3115 w3153 w3191 w3229 w3267 w3305 w3343 w3381 w3419 w3457 w3495 w3533 w3571 w3609 w3647 w3685 w3723 w3761 w3799 w3837 w3875 w3913 w3951 w3989 w4027 w4065 w4103 w4141 w4179 w4217 w4255 w4293 w4331 w4369 w4407 w4445 w4483 w4521 w4559 w4597 w4635 w4673 w4711 w4749 w4787 w4825 w4843] -> w149
      tunnel: w148 -> [_ _ _ _ _ _ _ _ _ _ _ _ _ _ _ _ _ _ _ w1445 _ _ w1531 _ _ w1613 w1637 w1680 _ w1731 w1766 _ _ _ _ _ _ _ _ _ _ _ _ _ _ _ _ _ _ _ _ _ _ _ _ _ _ _ _ _ _ _ _ _ _ _ _ _ _ _ _ _ _ _ _ _ _ _ _ _ _ _ _ _ _ _ _ _ _ _ _ _ _ _ _ _ _ _ _ _ _ _ _ _]
      tunnel: w138 -> [w181 w974 w990 _ _ _ w1089 _ w1123 w1187 _ _ _ _ _ _ _ _ _ _ _ _ _ _ _ _ _ w1668 _ _ _ _ w1833 w1867 w1936 w2005 w2075 w2146 w2215 w2288 w2356 w2426 w2497 w2578 w2616 w2654 w2692 w2730 w2768 w2806 w2844 w2882 w2920 w2958 w2996 w3034 w3072 w3110 w3148 w3186 w3224 w3262 w3300 w3338 w3376 w3414 w3452 w3490 w3528 w3566 w3604 w3642 w3680 w3718 w3756 w3794 w3832 w3870 w3908 w3946 w3984 w4022 w4060 w4098 w4136 w4174 w4212 w4250 w4288 w4326 w4364 w4402 w4440 w4478 w4516 w4554 w4592 w4630 w4668 w4706 w4744 w4782 w4820 _]
      tunnel: [w180 w977 w988 w1000 w1045 w1065 w1091 w1113 w1127 w1201 w1222 w1245 w1268 w1293 w1327 w1346 w1364 w1383 w1413 w1438 w1465 w1509 w1529 w1552 w1587 w1611 w1635 w1678 w1708 w1729 w1764 w1797 w1843 w1883 w1954 w2023 w2093 w2163 w2233 w2303 w2373 w2444 w2515 w2582 w2620 w2658 w2696 w2734 w2772 w2810 w2848 w2886 w2924 w2962 w3000 w3038 w3076 w3114 w3152 w3190 w3228 w3266 w3304 w3342 w3380 w3418 w3456 w3494 w3532 w3570 w3608 w3646 w3684 w3722 w3760 w3798 w3836 w3874 w3912 w3950 w3988 w4026 w4064 w4102 w4140 w4178 w4216 w4254 w4292 w4330 w4368 w4406 w4444 w4482 w4520 w4558 w4596 w4634 w4672 w4710 w4748 w4786 w4824 w4842] -> w147
      tunnel: w146 -> [w179 w977 w988 w1000 w1045 w1065 w1091 w1113 w1127 w1201 w1222 w1245 w1268 w1293 w1327 w1346 w1364 w1383 w1413 w1438 w1465 w1509 w1529 w1552 w1587 w1611 w1635 w1678 w1708 w1729 w1764 w1797 w1843 w1883 w1954 w2023 w2093 w2163 w2233 w2303 w2373 w2444 w2515 w2582 w2620 w2658 w2696 w2734 w2772 w2810 w2848 w2886 w2924 w2962 w3000 w3038 w3076 w3114 w3152 w3190 w3228 w3266 w3304 w3342 w3380 w3418 w3456 w3494 w3532 w3570 w3608 w3646 w3684 w3722 w3760 w3798 w3836 w3874 w3912 w3950 w3988 w4026 w4064 w4102 w4140 w4178 w4216 w4254 w4292 w4330 w4368 w4406 w4444 w4482 w4520 w4558 w4596 w4634 w4672 w4710 w4748 w4786 w4824 w4842]
      tunnel: w144 -> [w178 _ _ w1008 _ _ _ _ _ _ _ _ _ _ _ _ _ _ _ _ _ _ _ _ w1578 _ _ _ _ _ _ _ w1832 _ _ _ _ _ _ _ _ _ _ _ _ _ _ _ _ _ _ _ _ _ _ _ _ _ _ _ _ _ _ _ _ _ _ _ _ _ _ _ _ _ _ _ _ _ _ _ _ _ _ _ _ _ _ _ _ _ _ _ _ _ _ _ _ _ _ _ _ _ _ _]
      tunnel: [w173 w976 w986 w1005 w1044 w1060 w1085 w1112 w1126 w1200 w1221 w1244 w1267 w1291 w1325 w1344 w1363 w1382 w1410 w1436 w1462 w1508 w1528 w1551 w1586 w1608 w1634 w1662 w1707 w1728 w1763 w1796 w1831 w1886 w1958 w2027 w2097 w2167 w2237 w2307 w2377 w2448 w2519 w2567 w2605 w2643 w2681 w2719 w2757 w2795 w2833 w2871 w2909 w2947 w2985 w3023 w3061 w3099 w3137 w3175 w3213 w3251 w3289 w3327 w3365 w3403 w3441 w3479 w3517 w3555 w3593 w3631 w3669 w3707 w3745 w3783 w3821 w3859 w3897 w3935 w3973 w4011 w4049 w4087 w4125 w4163 w4201 w4239 w4277 w4315 w4353 w4391 w4429 w4467 w4505 w4543 w4581 w4619 w4657 w4695 w4733 w4771 w4809 w4841] -> w143
      tunnel: w142 -> [w173 w976 w986 w1005 w1044 w1060 w1085 w1112 w1126 w1200 w1221 w1244 w1267 w1291 w1325 w1344 w1363 w1382 w1410 w1436 w1462 w1508 w1528 w1551 w1586 w1608 w1634 w1662 w1707 w1728 w1763 w1796 w1831 _ _ _ _ _ _ _ _ _ _ w2567 w2605 w2643 w2681 w2719 w2757 w2795 w2833 w2871 w2909 w2947 w2985 w3023 w3061 w3099 w3137 w3175 w3213 w3251 w3289 w3327 w3365 w3403 w3441 w3479 w3517 w3555 w3593 w3631 w3669 w3707 w3745 w3783 w3821 w3859 w3897 w3935 w3973 w4011 w4049 w4087 w4125 w4163 w4201 w4239 w4277 w4315 w4353 w4391 w4429 w4467 w4505 w4543 w4581 w4619 w4657 w4695 w4733 w4771 w4809 w4841]
      tunnel: [w177 w975 w985 w1011 w1043 w1059 w1084 w1111 w1125 w1199 w1220 w1243 w1266 w1290 w1324 w1343 w1362 w1381 w1409 w1435 w1461 w1507 w1527 w1550 w1585 w1607 w1633 w1669 w1706 w1727 w1762 w1795 w1830 w1862 w1957 w2026 w2096 w2166 w2236 w2306 w2376 w2447 w2518 w2560 w2604 w2642 w2680 w2718 w2756 w2794 w2832 w2870 w2908 w2946 w2984 w3022 w3060 w3098 w3136 w3174 w3212 w3250 w3288 w3326 w3364 w3402 w3440 w3478 w3516 w3554 w3592 w3630 w3668 w3706 w3744 w3782 w3820 w3858 w3896 w3934 w3972 w4010 w4048 w4086 w4124 w4162 w4200 w4238 w4276 w4314 w4352 w4390 w4428 w4466 w4504 w4542 w4580 w4618 w4656 w4694 w4732 w4770 w4808 w4840] -> w141
      tunnel: w140 -> [w177 w975 w985 w1011 w1043 w1059 w1084 w1111 w1125 w1199 w1220 w1243 w1266 w1290 w1324 w1343 w1362 w1381 w1409 w1435 w1461 w1507 w1527 w1550 w1585 w1607 w1633 w1669 w1706 w1727 w1762 w1795 w1830 w1862 w1957 w2026 w2096 w2166 w2236 w2306 w2376 w2447 w2518 _ _ _ _ _ _ _ _ _ _ _ _ _ _ _ _ _ _ _ _ _ _ _ _ _ _ _ _ _ _ _ _ _ _ _ _ _ _ _ _ _ _ _ _ _ _ _ _ _ _ _ _ _ _ _ _ _ _ _ _ w4840]
      tunnel: w137 -> [w176 _ _ _ _ _ _ _ _ _ _ _ _ _ _ _ _ _ _ _ _ w1499 _ _ _ _ _ _ _ _ _ _ _ _ _ _ _ _ _ _ _ _ _ _ _ _ _ _ _ _ _ _ _ _ _ _ _ _ _ _ _ _ _ _ _ _ _ _ _ _ _ _ _ _ _ _ _ _ _ _ _ _ _ _ _ _ _ _ _ _ _ _ _ _ _ _ _ _ _ _ _ _ _ _]
      tunnel: [_ _ _ _ _ _ _ _ _ _ _ _ _ _ _ _ _ _ _ _ _ _ _ _ _ _ _ _ _ _ _ TRUE _ _ _ _ _ _ _ _ _ _ _ _ _ _ _ _ _ _ _ _ _ _ _ _ _ _ _ _ _ _ _ _ _ _ _ _ _ _ _ _ _ _ _ _ _ _ _ _ _ _ _ _ _ _ _ _ _ _ _ _ _ _ _ _ _ _ _ _ _ _ _ _] -> w136
      tunnel: [w171 w969 w981 w999 "Completed" w1057 w1080 w1110 "Initialize Apps" w1171 w1216 w1239 w1262 w1285 w1319 w1338 w1357 w1376 w1396 w1430 w1456 w1494 w1522 w1544 w1579 w1602 w1626 w1659 w1698 w1720 w1755 w1788 "Shorted Circuit" "Test Channel 1" "Test Channel 2" "Test Channel 3" "Test Channel 4" "Test Channel 5" "Test Channel 6" "Test Channel 7" "Test Channel 8" "Test Channel 9" "Test Channel 10" w2559 w2597 w2635 w2673 w2711 w2749 w2787 w2825 w2863 w2901 w2939 w2977 w3015 w3053 w3091 w3129 w3167 w3205 w3243 w3281 w3319 w3357 w3395 w3433 w3471 w3509 w3547 w3585 w3623 w3661 w3699 w3737 w3775 w3813 w3851 w3889 w3927 w3965 w4003 w4041 w4079 w4117 w4155 w4193 w4231 w4269 w4307 w4345 w4383 w4421 w4459 w4497 w4535 w4573 w4611 w4649 w4687 w4725 w4763 w4801 w4839] -> w133
      tunnel: w132 -> [w172 w969 w981 w999 _ w1057 w1080 w1110 _ w1171 w1216 w1239 w1262 w1285 w1319 w1338 w1357 w1376 w1396 w1430 w1456 w1494 w1522 w1544 w1579 w1602 w1626 w1659 w1698 w1720 w1755 w1788 _ _ _ _ _ _ _ _ _ _ _ w2559 w2597 w2635 w2673 w2711 w2749 w2787 w2825 w2863 w2901 w2939 w2977 w3015 w3053 w3091 w3129 w3167 w3205 w3243 w3281 w3319 w3357 w3395 w3433 w3471 w3509 w3547 w3585 w3623 w3661 w3699 w3737 w3775 w3813 w3851 w3889 w3927 w3965 w4003 w4041 w4079 w4117 w4155 w4193 w4231 w4269 w4307 w4345 w4383 w4421 w4459 w4497 w4535 w4573 w4611 w4649 w4687 w4725 w4763 w4801 w4839]
      frame "Apps.WaitForEvent", Default {
        n102 = event shown="[2] \"Again\": Value Change" {
          selector: w186 -> [_ w208 _ _ _ _ _ _ _ _ _ _ _ _ _ _ _ _ _ _ _ _ _ _ _ _ _ _ _ _ _ _ _ _ _ _ _ _]
          dyn-events: [_ w208 _ _ _ _ _ _ _ _ _ _ _ _ _ _ _ _ _ _ _ _ _ _ _ _ _ _ _ _ _ _ _ _ _ _ _ _] -> w185
          timeout: w174 -> [_ _ _ _ _ _ _ _ _ _ _ _ _ _ _ _ _ _ _ _ _ _ _ _ _ _ _ _ _ _ _ _ _ _ _ _ _ _]
          tunnel: [w191 100 w230 w252 w291 w301 w310 w316 w336 w353 w370 w384 w403 w427 w444 w459 w481 w498 w515 w539 w558 w576 w600 w686 w716 w733 w752 w771 w790 w809 w828 w847 w866 w885 w904 w916 w935 w954] -> w187
          tunnel: w174 -> [w191 _ w230 w251 w291 w301 w310 w316 w336 w353 w370 w384 w403 w427 w444 w459 w481 w498 w515 w539 w558 w576 w600 w686 w716 w733 w752 w771 w790 w809 w828 w847 w866 w885 w904 w916 w935 w954]
          tunnel: [w195 w207 w226 w249 w285 w293 w305 w314 w331 w348 w365 w382 w401 w420 w439 w456 w479 w496 w513 w532 w550 w570 w592 w685 w713 w731 w750 w769 w788 w807 w826 w845 w864 w883 w902 w914 w931 w951] -> w183
          tunnel: w182 -> [w189 w207 w228 w257 w286 w295 w309 w313 w330 w347 w364 w381 w400 w419 w438 w455 w478 w495 w512 w531 w552 w574 w591 w684 w714 w732 w751 w770 w789 w808 w827 w846 w865 w884 w903 w913 w930 w952]
          tunnel: w181 -> [w192 _ w229 w259 w289 w297 w308 w319 w335 w352 w369 w389 w408 w424 w443 w467 w484 w501 w520 w536 w557 w577 w594 w673 w710 w728 w747 w766 w785 w804 w823 w843 w861 w880 w899 _ _ _]
          tunnel: [w196 w211 w221 w258 w290 w299 w303 w315 w333 w349 w366 w383 w402 w421 w440 w458 w480 w497 w514 w538 w553 w571 w595 w687 w709 w726 w745 w764 w783 w802 w821 w841 w859 w878 w897 w915 w934 w953] -> w180
          tunnel: w179 -> [w196 w211 w221 w258 w290 w299 w303 w315 w333 w349 w366 w383 w402 w421 w440 w458 w480 w497 w514 w538 w553 _ w599 w687 w709 w726 w745 w764 w783 w802 w821 w841 w859 w878 w897 w915 w934 w953]
          tunnel: w178 -> [_ w205 _ _ _ _ _ _ _ _ _ _ _ _ _ _ _ _ _ _ _ _ _ _ _ w725 w742 w760 w779 w798 w817 w836 w855 w874 w893 _ _ _]
          tunnel: w175 -> [w194 w210 _ _ _ _ _ w312 w329 w346 w363 w380 w399 w418 w437 w454 w477 w494 w511 w530 w549 w572 w589 w683 _ _ _ _ _ _ _ _ _ _ _ w912 w933 w950]
          tunnel: w176 -> [_ _ _ _ _ _ _ _ _ _ _ _ _ _ _ _ _ _ _ _ _ _ _ _ _ _ _ _ _ _ _ _ _ _ _ _ _ _]
          tunnel: w173 -> [_ _ _ _ _ _ _ _ _ _ _ _ _ _ _ _ _ _ _ _ _ _ w587 _ _ _ _ _ _ _ _ _ _ _ _ _ _ _]
          tunnel: w172 -> [w188 _ w220 _ _ w292 w302 w311 w328 w345 w362 w379 w398 w417 w436 w453 w476 w493 w510 w529 w548 w567 w586 w670 w708 w721 w740 w759 w778 w797 w816 w835 w854 w873 w892 w910 w929 w948]
          tunnel: [w188 "Wait for JIG lock" w220 "Start auto test" "Settings" w292 w302 w311 w328 w345 w362 w379 w398 w417 w436 w453 w476 w493 w510 w529 w548 w567 w586 w670 w708 w721 w740 w759 w778 w797 w816 w835 w854 w873 w892 w910 w929 w948] -> w171
          event Timeout {
            n103 = event-data() -> ()  [unwired: 1 in, 1 out]
            n104 = disable-structure shown="LOGGING==TRUE" {
              disable-tunnel: w194 -> [w197 _]
              frame condition #0 (active) {
                n105 = Empty String/Path?(string/path=w197) -> (empty?=w204:bool)
                n106 = Select(t="Quece timeout", s=w204, f=w197) -> (s? t:f=w202:string)
                n107 = Format Into String(format string=": %s", initial string=w202, "UI timeout") -> (resulting string=w199:string)  [unwired: 1 in, 1 out]
                n108 = call "string log (SubVI).vi"("Enum"=enum16{"Init", "Log", "Read"}."Log", "state Name"=w199) -> ()  [unwired: 8 in, 2 out]
              }
              frame condition #1 {
              }
            }
            n109 = call "App enquece.vi"("command"="Apps.WaitingForTrigger", "queue in"=w192) -> ("error out"=w190:errorcluster)  [unwired: 8 in, 1 out]
            n110 = Merge Errors(w189, w190) -> (w195:errorcluster)
          }
          event "Test": Value Change {
            n111 = event-data() -> ()  [unwired: 1 in, 1 out]
            n112 = disable-structure shown="LOGGING==TRUE" {
              disable-tunnel: w210 -> [w212 _]
              frame condition #0 (active) {
                n113 = Empty String/Path?(string/path=w212) -> (empty?=w219:bool)
                n114 = Select(t="Quece timeout", s=w219, f=w212) -> (s? t:f=w217:string)
                n115 = Format Into String(format string=": %s", initial string=w217, "Test") -> (resulting string=w214:string)  [unwired: 1 in, 1 out]
                n116 = call "string log (SubVI).vi"("Enum"=enum16{"Init", "Log", "Read"}."Log", "state Name"=w214) -> ()  [unwired: 8 in, 2 out]
              }
              frame condition #1 {
              }
            }
            n117 = call "reset DRV UI (SubVI).vi"("Ref  in"=w205) -> ()  [unwired: 9 in, 2 out]
          }
          event "Again": Value Change {
            n118 = event-data() -> ()  [unwired: 1 in, 1 out]
            n119 = Initialize Array(FALSE, 6 ("dimension size"), 10 ("dimension size")) -> (w222:bool[][])
            n120 = local write "Short DRV"(w222) -> ()
            n121 = disable-structure shown="Enabled" {
              disable-tunnel: w229 -> [w235 _]
              disable-tunnel: [w234 w241] -> w227
              frame Disabled {
                n122 = Build Array("Test Shorted Circuits", "Test Channel 1") -> (w232:string[])
                n123 = for {
                  tunnel: w235 -> [w238]
                  tunnel: [w237] -> w234 mode=indexing
                  tunnel: w232 -> [w236] mode=indexing
                  n124 = call "App enquece.vi"("command"=w236, "queue in"=w238) -> ("error out"=w237:errorcluster)  [unwired: 8 in, 1 out]
                }
              }
              frame Enabled {
                n125 = invoke class="VI" method="FP.Open"("State"=T15."Hidden") -> (error out=w243:errorcluster)  [unwired: 4 in, 4 out]
                n126 = call "View DRV data.vi"("error in (no error)"=w243) -> ("error out"=w242:errorcluster)  [unwired: 10 in]
                n127 = invoke class="VI" method="FP.Open"(error in=w242, "State"=T15."Standard") -> (error out=w241:errorcluster)  [unwired: 3 in, 4 out]
              }
            }
            n128 = Merge Errors(w228, w227) -> (w226:errorcluster)
          }
          event User Event {
            # "#HungNotes:\nStart HV60D from this frame (check new board  installed)"
            # "Stop Timeout event"
            n129 = event-data() -> ("new board?"=w250:bool, "new trigger"=→"new Trigger?":bool, "last trigger"=→"last Trigger?":bool)  [unwired: 1 in, 4 out]
            "New board?" <- w250
            n130 = control-ref of="DRV 61"() -> (w245:refnum<vi>)
            n131 = case shown="False" w250 {
              tunnel: w259 -> [_ w272]
              tunnel: [_ w279] -> w256
              frame False {
              }
              frame True {
                n132 = Build Array("Test Shorted Circuits", "Test Channel 1", "Test Channel 2", "Test Channel 3", "Test Channel 4", "Test Channel 5", "Test Channel 6") -> (w265:string[])
                n133 = Build Array("Test Channel 7", "Test Channel 8", "Test Channel 9", "Test Channel 10", "MEAS.AllRelaysOFF", "MEAS.Reset JIG", "Apps.UI Update 2") -> (w264:string[])
                n134 = Build Array (concatenate)(w265, w264) -> (w263:string[])
                n135 = for {
                  tunnel: w272 -> [w283]
                  tunnel: [w282] -> w279 mode=indexing
                  tunnel: w263 -> [w281] mode=indexing
                  n136 = call "App enquece.vi"("command"=w281, "queue in"=w283) -> ("error out"=w282:errorcluster)  [unwired: 8 in, 1 out]
                }
              }
            }
            n137 = property class="ColBox"(reference=w245, "Value"=u32 10000536 ("DRV 1")) -> ()  [unwired: 1 in, 2 out]
            n138 = Select(t=-1, s=w250, f=w251) -> (s? t:f=w252:i32)
            n139 = Merge Errors(w257, w256) -> (w248:errorcluster)
            n140 = local write "time elased(ms)"(w247) -> ()
            n141 = flat-sequence {
              tunnel: [w261] -> w249
              tunnel: w248 -> [w261]
              tunnel: [u32 0 ("time elased(ms)")] -> w247
              frame #0 {
                n142 = call "FGV milisec (subVI).vi"() -> ()  [unwired: 11 in, 1 out]
              }
            }
          }
          event "Settings": Value Change {
            n143 = event-data() -> ()  [unwired: 1 in, 6 out]
            n144 = call "App enquece.vi"("command"="INIT.Read DRV code", "queue in"=w289) -> ("error out"=w287:errorcluster)  [unwired: 8 in, 1 out]
            n145 = Merge Errors(w286, w287) -> (w285:errorcluster)
          }
          event Panel Close? {
            n146 = event-data() -> ()  [unwired: 1 in, 4 out]
            n147 = call "App enquece.vi"("Priority Enquece"=TRUE, "command"="Apps.Exit", "queue in"=w297) -> ("error out"=w294:errorcluster)  [unwired: 7 in, 1 out]
            n148 = Merge Errors(w295, w294) -> (w293:errorcluster)
            n149 = event-data("Discard?"=TRUE) -> ()  [unwired: 1 in, 1 out]
          }
          event "Exit": Value Change {
            n150 = event-data() -> ()  [unwired: 1 in, 1 out]
            n151 = call "App enquece.vi"("Priority Enquece"=TRUE, "command"="Apps.Exit", "queue in"=w308) -> ("error out"=w307:errorcluster)  [unwired: 7 in, 1 out]
            n152 = Merge Errors(w309, w307) -> (w305:errorcluster)
          }
          event "check connected": Value Change {
            n153 = event-data() -> ()  [unwired: 1 in, 1 out]
            n154 = disable-structure shown="LOGGING==TRUE" {
              disable-tunnel: w312 -> [w320 _]
              frame condition #0 (active) {
                n155 = Empty String/Path?(string/path=w320) -> (empty?=w327:bool)
                n156 = Select(t="Quece timeout", s=w327, f=w320) -> (s? t:f=w325:string)
                n157 = Format Into String(format string=": %s", initial string=w325, "Check connected") -> (resulting string=w322:string)  [unwired: 1 in, 1 out]
                n158 = call "string log (SubVI).vi"("Enum"=enum16{"Init", "Log", "Read"}."Log", "state Name"=w322) -> ()  [unwired: 8 in, 2 out]
              }
              frame condition #1 {
              }
            }
            n159 = call "App enquece.vi"("command"="MEAS.Read EMIC connected", "queue in"=w319) -> ("error out"=w317:errorcluster)  [unwired: 8 in, 1 out]
            n160 = Merge Errors(w313, w317) -> (w314:errorcluster)
          }
          event "Open COM eMIC": Value Change {
            n161 = event-data() -> ()  [unwired: 1 in, 1 out]
            n162 = disable-structure shown="LOGGING==TRUE" {
              disable-tunnel: w329 -> [w337 _]
              frame condition #0 (active) {
                n163 = Empty String/Path?(string/path=w337) -> (empty?=w344:bool)
                n164 = Select(t="Quece timeout", s=w344, f=w337) -> (s? t:f=w342:string)
                n165 = Format Into String(format string=": %s", initial string=w342, "Open COM eMIC") -> (resulting string=w339:string)  [unwired: 1 in, 1 out]
                n166 = call "string log (SubVI).vi"("Enum"=enum16{"Init", "Log", "Read"}."Log", "state Name"=w339) -> ()  [unwired: 8 in, 2 out]
              }
              frame condition #1 {
              }
            }
            n167 = call "App enquece.vi"("command"="INIT.Open COM EMIC", "queue in"=w335) -> ("error out"=w334:errorcluster)  [unwired: 8 in, 1 out]
            n168 = Merge Errors(w330, w334) -> (w331:errorcluster)
          }
          event "Read trigger": Value Change {
            n169 = event-data() -> ()  [unwired: 1 in, 1 out]
            n170 = disable-structure shown="LOGGING==TRUE" {
              disable-tunnel: w346 -> [w354 _]
              frame condition #0 (active) {
                n171 = Empty String/Path?(string/path=w354) -> (empty?=w361:bool)
                n172 = Select(t="Quece timeout", s=w361, f=w354) -> (s? t:f=w359:string)
                n173 = Format Into String(format string=": %s", initial string=w359, "Read Trigger") -> (resulting string=w356:string)  [unwired: 1 in, 1 out]
                n174 = call "string log (SubVI).vi"("Enum"=enum16{"Init", "Log", "Read"}."Log", "state Name"=w356) -> ()  [unwired: 8 in, 2 out]
              }
              frame condition #1 {
              }
            }
            n175 = call "App enquece.vi"("command"="MEAS.Read TRIGGER", "queue in"=w352) -> ("error out"=w350:errorcluster)  [unwired: 8 in, 1 out]
            n176 = Merge Errors(w347, w350) -> (w348:errorcluster)
          }
          event "Read Optos": Value Change {
            n177 = event-data() -> ()  [unwired: 1 in, 1 out]
            n178 = disable-structure shown="LOGGING==TRUE" {
              disable-tunnel: w363 -> [w371 _]
              frame condition #0 (active) {
                n179 = Empty String/Path?(string/path=w371) -> (empty?=w378:bool)
                n180 = Select(t="Quece timeout", s=w378, f=w371) -> (s? t:f=w376:string)
                n181 = Format Into String(format string=": %s", initial string=w376, "Read Optos") -> (resulting string=w373:string)  [unwired: 1 in, 1 out]
                n182 = call "string log (SubVI).vi"("Enum"=enum16{"Init", "Log", "Read"}."Log", "state Name"=w373) -> ()  [unwired: 8 in, 2 out]
              }
              frame condition #1 {
              }
            }
            n183 = call "App enquece.vi"("command"="MEAS.Read Optos", "queue in"=w369) -> ("error out"=w367:errorcluster)  [unwired: 8 in, 1 out]
            n184 = Merge Errors(w364, w367) -> (w365:errorcluster)
          }
          event "DMM select Current Input": Value Change {
            n185 = event-data() -> ()  [unwired: 1 in, 1 out]
            n186 = disable-structure shown="LOGGING==TRUE" {
              disable-tunnel: w380 -> [w390 _]
              frame condition #0 (active) {
                n187 = Empty String/Path?(string/path=w390) -> (empty?=w397:bool)
                n188 = Select(t="Quece timeout", s=w397, f=w390) -> (s? t:f=w395:string)
                n189 = Format Into String(format string=": %s", initial string=w395, "DMM Current Input") -> (resulting string=w392:string)  [unwired: 1 in, 1 out]
                n190 = call "string log (SubVI).vi"("Enum"=enum16{"Init", "Log", "Read"}."Log", "state Name"=w392) -> ()  [unwired: 8 in, 2 out]
              }
              frame condition #1 {
              }
            }
            n191 = To Variant(anything="mux2-1(DMM I) encode") -> (Variant=w386:variant)
            n192 = call "App enquece.vi"("command data"=w386, "command"="MEAS.Set Input Current", "queue in"=w389) -> ("error out"=w385:errorcluster)  [unwired: 7 in, 1 out]
            n193 = Merge Errors(w381, w385) -> (w382:errorcluster)
          }
          event "DEMUX 1-10": Value Change {
            n194 = event-data() -> ()  [unwired: 1 in, 1 out]
            n195 = disable-structure shown="LOGGING==TRUE" {
              disable-tunnel: w399 -> [w409 _]
              frame condition #0 (active) {
                n196 = Empty String/Path?(string/path=w409) -> (empty?=w416:bool)
                n197 = Select(t="Quece timeout", s=w416, f=w409) -> (s? t:f=w414:string)
                n198 = Format Into String(format string=": %s", initial string=w414, "demux1-10") -> (resulting string=w411:string)  [unwired: 1 in, 1 out]
                n199 = call "string log (SubVI).vi"("Enum"=enum16{"Init", "Log", "Read"}."Log", "state Name"=w411) -> ()  [unwired: 8 in, 2 out]
              }
              frame condition #1 {
              }
            }
            n200 = To Variant(anything="demux1_10(x6)_encode") -> (Variant=w405:variant)
            n201 = call "App enquece.vi"("command data"=w405, "command"="MEAS.demux1-10", "queue in"=w408) -> ("error out"=w404:errorcluster)  [unwired: 7 in, 1 out]
            n202 = Merge Errors(w400, w404) -> (w401:errorcluster)
          }
          event "eMIC": Value Change {
            n203 = event-data() -> ()  [unwired: 1 in, 1 out]
            n204 = disable-structure shown="LOGGING==TRUE" {
              disable-tunnel: w418 -> [w428 _]
              frame condition #0 (active) {
                n205 = Empty String/Path?(string/path=w428) -> (empty?=w435:bool)
                n206 = Select(t="Quece timeout", s=w435, f=w428) -> (s? t:f=w433:string)
                n207 = Format Into String(format string=": %s", initial string=w433, "eMIC") -> (resulting string=w430:string)  [unwired: 1 in, 1 out]
                n208 = call "string log (SubVI).vi"("Enum"=enum16{"Init", "Log", "Read"}."Log", "state Name"=w430) -> ()  [unwired: 8 in, 2 out]
              }
              frame condition #1 {
              }
            }
            n209 = To Variant(anything="eMIC 6 values") -> (Variant=w422:variant)
            n210 = call "App enquece.vi"("command data"=w422, "command"="MEAS.eMIC", "queue in"=w424) -> ("error out"=w426:errorcluster)  [unwired: 7 in, 1 out]
            n211 = Merge Errors(w419, w426) -> (w420:errorcluster)
          }
          event "connect DMM": Value Change {
            n212 = event-data() -> ()  [unwired: 1 in, 1 out]
            n213 = disable-structure shown="LOGGING==TRUE" {
              disable-tunnel: w437 -> [w445 _]
              frame condition #0 (active) {
                n214 = Empty String/Path?(string/path=w445) -> (empty?=w452:bool)
                n215 = Select(t="Quece timeout", s=w452, f=w445) -> (s? t:f=w450:string)
                n216 = Format Into String(format string=": %s", initial string=w450, "Connect DMM") -> (resulting string=w447:string)  [unwired: 1 in, 1 out]
                n217 = call "string log (SubVI).vi"("Enum"=enum16{"Init", "Log", "Read"}."Log", "state Name"=w447) -> ()  [unwired: 8 in, 2 out]
              }
              frame condition #1 {
              }
            }
            n218 = call "App enquece.vi"("command"="INIT.Open COM DMM", "queue in"=w443) -> ("error out"=w442:errorcluster)  [unwired: 8 in, 1 out]
            n219 = Merge Errors(w438, w442) -> (w439:errorcluster)
          }
          event "config DMM": Value Change {
            n220 = event-data() -> ()  [unwired: 1 in, 1 out]
            n221 = disable-structure shown="LOGGING==TRUE" {
              disable-tunnel: w454 -> [w468 _]
              frame condition #0 (active) {
                n222 = Empty String/Path?(string/path=w468) -> (empty?=w475:bool)
                n223 = Select(t="Quece timeout", s=w475, f=w468) -> (s? t:f=w473:string)
                n224 = Format Into String(format string=": %s", initial string=w473, "config DMM") -> (resulting string=w470:string)  [unwired: 1 in, 1 out]
                n225 = call "string log (SubVI).vi"("Enum"=enum16{"Init", "Log", "Read"}."Log", "state Name"=w470) -> ()  [unwired: 8 in, 2 out]
              }
              frame condition #1 {
              }
            }
            n226 = Bundle By Name(cluster=T16 {"DMM config cluster"={"DCV range"=0.0, "DCI range"=0.0, "Detector Rate"=0}, "mux2-1(DMM I) encode"=enum."DMM I (0.5)"} ("DMM all config"), "DMM config cluster.DCV range"="DCV range", "DMM config cluster.DCI range"="DCI range", "DMM config cluster.Detector Rate"="Detector Rate") -> (w462:T16)
            n227 = To Variant(anything=w462) -> (Variant=w460:variant)
            n228 = call "App enquece.vi"("command data"=w460, "command"="MEAS.Set DMM config", "queue in"=w467) -> ("error out"=w457:errorcluster)  [unwired: 7 in, 1 out]
            n229 = Merge Errors(w455, w457) -> (w456:errorcluster)
          }
          event "DMM read dual value": Value Change {
            n230 = event-data() -> ()  [unwired: 1 in, 1 out]
            n231 = disable-structure shown="LOGGING==TRUE" {
              disable-tunnel: w477 -> [w485 _]
              frame condition #0 (active) {
                n232 = Empty String/Path?(string/path=w485) -> (empty?=w492:bool)
                n233 = Select(t="Quece timeout", s=w492, f=w485) -> (s? t:f=w490:string)
                n234 = Format Into String(format string=": %s", initial string=w490, "DMM read dual value") -> (resulting string=w487:string)  [unwired: 1 in, 1 out]
                n235 = call "string log (SubVI).vi"("Enum"=enum16{"Init", "Log", "Read"}."Log", "state Name"=w487) -> ()  [unwired: 8 in, 2 out]
              }
              frame condition #1 {
              }
            }
            n236 = call "App enquece.vi"("command"="MEAS.DMM dual read", "queue in"=w484) -> ("error out"=w482:errorcluster)  [unwired: 8 in, 1 out]
            n237 = Merge Errors(w478, w482) -> (w479:errorcluster)
          }
          event "Reset JIG": Value Change {
            n238 = event-data() -> ()  [unwired: 1 in, 1 out]
            n239 = disable-structure shown="LOGGING==TRUE" {
              disable-tunnel: w494 -> [w502 _]
              frame condition #0 (active) {
                n240 = Empty String/Path?(string/path=w502) -> (empty?=w509:bool)
                n241 = Select(t="Quece timeout", s=w509, f=w502) -> (s? t:f=w507:string)
                n242 = Format Into String(format string=": %s", initial string=w507, "reset JIG") -> (resulting string=w504:string)  [unwired: 1 in, 1 out]
                n243 = call "string log (SubVI).vi"("Enum"=enum16{"Init", "Log", "Read"}."Log", "state Name"=w504) -> ()  [unwired: 8 in, 2 out]
              }
              frame condition #1 {
              }
            }
            n244 = call "App enquece.vi"("command"="MEAS.Reset JIG", "queue in"=w501) -> ("error out"=w499:errorcluster)  [unwired: 8 in, 1 out]
            n245 = Merge Errors(w495, w499) -> (w496:errorcluster)
          }
          event "TurnON/OFF +5V": Value Change {
            n246 = event-data() -> ()  [unwired: 1 in, 1 out]
            n247 = disable-structure shown="LOGGING==TRUE" {
              disable-tunnel: w511 -> [w521 _]
              frame condition #0 (active) {
                n248 = Empty String/Path?(string/path=w521) -> (empty?=w528:bool)
                n249 = Select(t="Quece timeout", s=w528, f=w521) -> (s? t:f=w526:string)
                n250 = Format Into String(format string=": %s", initial string=w526, "ON/OFF +5V") -> (resulting string=w523:string)  [unwired: 1 in, 1 out]
                n251 = call "string log (SubVI).vi"("Enum"=enum16{"Init", "Log", "Read"}."Log", "state Name"=w523) -> ()  [unwired: 8 in, 2 out]
              }
              frame condition #1 {
              }
            }
            n252 = To Variant(anything="5V Value") -> (Variant=w517:variant)
            n253 = call "App enquece.vi"("command data"=w517, "command"="MEAS.Turn+5V", "queue in"=w520) -> ("error out"=w519:errorcluster)  [unwired: 7 in, 1 out]
            n254 = Merge Errors(w512, w519) -> (w513:errorcluster)
          }
          event "mux 6-1": Value Change {
            n255 = event-data() -> ()  [unwired: 1 in, 1 out]
            n256 = disable-structure shown="LOGGING==TRUE" {
              disable-tunnel: w530 -> [w540 _]
              frame condition #0 (active) {
                n257 = Empty String/Path?(string/path=w540) -> (empty?=w547:bool)
                n258 = Select(t="Quece timeout", s=w547, f=w540) -> (s? t:f=w545:string)
                n259 = Format Into String(format string=": %s", initial string=w545, "mux6-1") -> (resulting string=w542:string)  [unwired: 1 in, 1 out]
                n260 = call "string log (SubVI).vi"("Enum"=enum16{"Init", "Log", "Read"}."Log", "state Name"=w542) -> ()  [unwired: 8 in, 2 out]
              }
              frame condition #1 {
              }
            }
            n261 = To Variant(anything="mux 6-1 data") -> (Variant=w534:variant)
            n262 = call "App enquece.vi"("command data"=w534, "command"="MEAS.mux6_1", "queue in"=w536) -> ("error out"=w533:errorcluster)  [unwired: 7 in, 1 out]
            n263 = Merge Errors(w531, w533) -> (w532:errorcluster)
          }
          event "Mux 10-1": Value Change {
            n264 = event-data() -> ()  [unwired: 1 in, 1 out]
            n265 = disable-structure shown="LOGGING==TRUE" {
              disable-tunnel: w549 -> [w559 _]
              frame condition #0 (active) {
                n266 = Empty String/Path?(string/path=w559) -> (empty?=w566:bool)
                n267 = Select(t="Quece timeout", s=w566, f=w559) -> (s? t:f=w564:string)
                n268 = Format Into String(format string=": %s", initial string=w564, "mux10-1") -> (resulting string=w561:string)  [unwired: 1 in, 1 out]
                n269 = call "string log (SubVI).vi"("Enum"=enum16{"Init", "Log", "Read"}."Log", "state Name"=w561) -> ()  [unwired: 8 in, 2 out]
              }
              frame condition #1 {
              }
            }
            n270 = To Variant(anything="mux 10-1 data") -> (Variant=w554:variant)
            n271 = call "App enquece.vi"("command data"=w554, "command"="MEAS.mux10-1", "queue in"=w557) -> ("error out"=w551:errorcluster)  [unwired: 7 in, 1 out]
            n272 = Merge Errors(w552, w551) -> (w550:errorcluster)
          }
          event "request AC": Value Change {
            w571 = T7 {"eMIC 1"={"ACV"=0.0, "ACI"=0.0, "pF"=0.0, "kW"=0.0, "Freq"=0.0}, "eMIC 2"={"ACV"=0.0, "ACI"=0.0, "pF"=0.0, "kW"=0.0, "Freq"=0.0}, "eMIC 3"={"ACV"=0.0, "ACI"=0.0, "pF"=0.0, "kW"=0.0, "Freq"=0.0}, "eMIC 4"={"ACV"=0.0, "ACI"=0.0, "pF"=0.0, "kW"=0.0, "Freq"=0.0}, "eMIC 5"={"ACV"=0.0, "ACI"=0.0, "pF"=0.0, "kW"=0.0, "Freq"=0.0}, "eMIC 6"={"ACV"=0.0, "ACI"=0.0, "pF"=0.0, "kW"=0.0, "Freq"=0.0}}  # eMICs cluster
            n273 = event-data() -> ()  [unwired: 1 in, 1 out]
            n274 = disable-structure shown="LOGGING==TRUE" {
              disable-tunnel: w572 -> [w578 _]
              frame condition #0 (active) {
                n275 = Empty String/Path?(string/path=w578) -> (empty?=w585:bool)
                n276 = Select(t="Quece timeout", s=w585, f=w578) -> (s? t:f=w583:string)
                n277 = Format Into String(format string=": %s", initial string=w583, "request AC") -> (resulting string=w580:string)  [unwired: 1 in, 1 out]
                n278 = call "string log (SubVI).vi"("Enum"=enum16{"Init", "Log", "Read"}."Log", "state Name"=w580) -> ()  [unwired: 8 in, 2 out]
              }
              frame condition #1 {
              }
            }
            n279 = call "FGV wait for 6 eMICs.vi"("Enum"=enum16{"Init", "count"}."Init") -> ("error out"=w568:errorcluster)  [unwired: 8 in, 2 out]
            n280 = call "App enquece.vi"("error in (no error)"=w568, "command"="MEAS.request AC", "queue in"=w577) -> ("error out"=w573:errorcluster)  [unwired: 7 in, 1 out]
            n281 = Merge Errors(w574, w573) -> (w570:errorcluster)
          }
          event User Event {
            # "TRUE means  6 eMICs have responsed\nthen update FGVs\nFALSE means  waiting  for  DUT data. \nthen move to other test channel"
            n282 = event-data() -> ("Module ID"=w588:i32, "Array"=w607:T21[])  [unwired: 1 in]
            n283 = call "FGV wait for 6 eMICs.vi"("Enum"=enum16{"Init", "count"}."count") -> ("error out"=w593:errorcluster, "wait done"=w596:bool)  [unwired: 8 in, 1 out]
            "AC Measure  Completed" <- w596
            n284 = for {
              tunnel: w607 -> [w653] mode=indexing
              shift-right: [w649] -> w598
              shift-left: T6 {"ACV"=0.0, "ACI"=0.0, "pF"=0.0, "kW"=0.0, "Freq"=0.0} ("eMIC response") -> [w651]
              n285 = Unbundle By Name(w653) -> ("float"=w650:dbl, "Name"=w652:string)
              n286 = case shown="\"ACV\"" w652 {
                tunnel: w651 -> [w654 w657 w660 w663 w666 w669]
                tunnel: w650 -> [_ w655 w658 w661 w665 w667]
                tunnel: [w654 w656 w659 w662 w664 w668] -> w649
                frame "False", Default {
                }
                frame "ACI" {
                  n287 = Bundle By Name(cluster=w657, "ACI"=w655) -> (w656:T6)
                }
                frame "kW" {
                  n288 = Bundle By Name(cluster=w660, "kW"=w658) -> (w659:T6)
                }
                frame "PF" {
                  n289 = Bundle By Name(cluster=w663, "pF"=w661) -> (w662:T6)
                }
                frame "ACV" {
                  n290 = Bundle By Name(cluster=w666, "ACV"=w665) -> (w664:T6)
                }
                frame "Freq" {
                  n291 = Bundle By Name(cluster=w669, "Freq"=w667) -> (w668:T6)
                }
              }
            }
            n292 = case shown="2" w588 {
              tunnel: [w630 w632 w635 w638 w641 w644 w647] -> w595
              tunnel: w599 -> [w630 w633 w636 w639 w642 w645 w648]
              tunnel: w598 -> [_ w631 w634 w637 w640 w643 w646]
              frame 0, Default {
              }
              frame 1 {
                n293 = Bundle By Name(cluster=w633, "eMIC 1"=w631) -> (w632:T7)
              }
              frame 2 {
                n294 = Bundle By Name(cluster=w636, "eMIC 2"=w634) -> (w635:T7)
              }
              frame 3 {
                n295 = Bundle By Name(cluster=w639, "eMIC 3"=w637) -> (w638:T7)
              }
              frame 4 {
                n296 = Bundle By Name(cluster=w642, "eMIC 4"=w640) -> (w641:T7)
              }
              frame 5 {
                n297 = Bundle By Name(cluster=w645, "eMIC 5"=w643) -> (w644:T7)
              }
              frame 6 {
                n298 = Bundle By Name(cluster=w648, "eMIC 6"=w646) -> (w647:T7)
              }
            }
            n299 = disable-structure shown="LOGGING==TRUE" {
              disable-tunnel: w589 -> [w615 _]
              disable-tunnel: w588 -> [w611 _]
              frame condition #0 (active) {
                n300 = Empty String/Path?(string/path=w615) -> (empty?=w617:bool)
                n301 = Select(t="Quece timeout", s=w617, f=w615) -> (s? t:f=w614:string)
                n302 = Format Into String(format string=":%s %d", initial string=w614, "CE14  data response", w611) -> (resulting string=w610:string)  [unwired: 1 in, 1 out]
                n303 = call "string log (SubVI).vi"("Enum"=enum16{"Init", "Log", "Read"}."Log", "state Name"=w610) -> ()  [unwired: 8 in, 2 out]
              }
              frame condition #1 {
              }
            }
            n304 = case shown="True" w596 {
              tunnel: w595 -> [_ w624]
              tunnel: w587 -> [_ w629]
              tunnel: w594 -> [w622 _]
              tunnel: w593 -> [w619 w626]
              tunnel: [w618 w625] -> w590
              frame False {
                n305 = call "App enquece.vi"("Priority Enquece"=TRUE, "error in (no error)"=w619, "command"="Apps.WaitForEvent", "queue in"=w622) -> ("error out"=w618:errorcluster)  [unwired: 6 in, 1 out]
              }
              frame True {
                n306 = To Variant(anything=w624) -> (Variant=w623:variant)
                n307 = call "FGV Driver Data.vi"("DUT channel (1-11)"=w629, "Mode"=DUT_data_Mode."AC parameter", "error in (no error)"=w626, "FGV enum"=FGV_DRV_data."Write" ("FGV DRV data enum"), "data"=w623) -> ("error out"=w625:errorcluster)  [unwired: 3 in, 3 out]
              }
            }
            n308 = Unbundle By Name(w595) -> ("eMIC 1"=→"eMIC 1":T6, "eMIC 2"=→"eMIC 2":T6, "eMIC 3"=→"eMIC 3":T6, "eMIC 4"=→"eMIC 4":T6, "eMIC 5"=→"eMIC 5":T6, "eMIC 6"=→"eMIC 6":T6)
            n309 = Merge Errors(w591, w590) -> (w592:errorcluster)
          }
          event User Event {
            n310 = event-data() -> ("Init?"=w680:bool, "Module ID"=w681:i32)  [unwired: 1 in]
            "Module ID" <- w681
            "AC Measure Module" <- w680
            n311 = disable-structure shown="LOGGING==TRUE" {
              disable-tunnel: w683 -> [w703 _]
              disable-tunnel: w681 -> [w699 _]
              frame condition #0 (active) {
                n312 = Empty String/Path?(string/path=w703) -> (empty?=w705:bool)
                n313 = Select(t="Quece timeout", s=w705, f=w703) -> (s? t:f=w702:string)
                n314 = Format Into String(format string=":%s %d", initial string=w702, "CE14 Did  it", w699) -> (resulting string=w698:string)  [unwired: 1 in, 1 out]
                n315 = call "string log (SubVI).vi"("Enum"=enum16{"Init", "Log", "Read"}."Log", "state Name"=w698) -> ()  [unwired: 8 in, 2 out]
              }
              frame condition #1 {
              }
            }
            n316 = disable-structure shown="DEBUGGING==TRUE" {
              disable-tunnel: w686 -> [w706 _]
              frame condition #0 {
                n317 = call "Show Panel.vi"("Module ID"=w706) -> ()  [unwired: 10 in, 1 out]
              }
              frame condition #1 (active) {
              }
            }
            n318 = Decrement(x=w681) -> (x-1=w682:i32)
            n319 = Initialize Array(FALSE, 6 ("dimension size")) -> (w676:bool[])
            n320 = feedback #2(w676) -> (w677:bool[])
            n321 = Replace Array Subset(array=w677, new element=w680, index=w682) -> (w675:bool[])
            "CE14  Module did it" <- w675
            n322 = feedback-in #2(w675) -> ()
            n323 = And Array Elements(Boolean array=w675) -> (logical AND=w674:bool)
            n324 = case shown="False" w674 {
              tunnel: w673 -> [_ w690]
              tunnel: [_ w689] -> w672
              frame False {
              }
              frame True {
                n325 = flat-sequence {
                  tunnel: [w692] -> w691
                  tunnel: w690 -> [w692]
                  tunnel: w691 -> [w695]
                  tunnel: [w694] -> w689
                  frame #0 {
                    n326 = Wait (ms)(milliseconds to wait=u32 500) -> ()  [unwired: 1 out]
                  }
                  frame #1 {
                    n327 = call "App enquece.vi"("command"="MEAS.Read EMIC connected", "queue in"=w695) -> ("error out"=w694:errorcluster)  [unwired: 8 in, 1 out]
                  }
                }
              }
            }
            n328 = control-ref of="Select CE14 eMIC Module Instance"() -> (w688:refnum<vi>)
            n329 = call "Update Select Module Ring.vi"("Select Module Ring Ref"=w688) -> ("error out"=w671:errorcluster)  [unwired: 8 in, 2 out]
            n330 = Merge Errors(w684, w672, w671) -> (w685:errorcluster)
          }
          event "Shorted Circuits Test": Value Change {
            n331 = event-data() -> ()  [unwired: 1 in, 1 out]
            n332 = Build Array("Test Shorted Circuits", "MEAS.AllRelaysOFF") -> (w711:string[])
            n333 = for {
              tunnel: [w719] -> w712 mode=indexing
              tunnel: w711 -> [w718] mode=indexing
              tunnel: w710 -> [w717]
              n334 = call "App enquece.vi"("command"=w718, "queue in"=w717) -> ("error out"=w719:errorcluster)  [unwired: 8 in, 1 out]
            }
            n335 = Merge Errors(w714, w712) -> (w713:errorcluster)
          }
          event "Test Channel 1": Value Change {
            n336 = event-data() -> ()  [unwired: 1 in, 1 out]
            n337 = Array Subset(array=w725, index=0, length=6) -> (w722:refnum<vi>[])
            n338 = for {
              tunnel: w722 -> [w734] mode=indexing
              n339 = property class="ColBox"(reference=w734, "Value"=u32 10000536 ("DRV 1")) -> ()  [unwired: 1 in, 2 out]
            }
            n340 = Build Array("Test Channel 1", "MEAS.AllRelaysOFF") -> (w729:string[])
            n341 = for {
              tunnel: [w738] -> w730 mode=indexing
              tunnel: w729 -> [w737] mode=indexing
              tunnel: w728 -> [w736]
              n342 = call "App enquece.vi"("command"=w737, "queue in"=w736) -> ("error out"=w738:errorcluster)  [unwired: 8 in, 1 out]
            }
            n343 = Merge Errors(w732, w730) -> (w731:errorcluster)
          }
          event "Test Channel 2": Value Change {
            n344 = event-data() -> ()  [unwired: 1 in, 1 out]
            n345 = Array Subset(array=w742, index=6, length=6) -> (w741:refnum<vi>[])
            n346 = for {
              tunnel: w741 -> [w753] mode=indexing
              n347 = property class="ColBox"(reference=w753, "Value"=u32 10000536 ("DRV 1")) -> ()  [unwired: 1 in, 2 out]
            }
            n348 = Build Array("Test Channel 2", "MEAS.AllRelaysOFF") -> (w748:string[])
            n349 = for {
              tunnel: [w757] -> w749 mode=indexing
              tunnel: w748 -> [w756] mode=indexing
              tunnel: w747 -> [w755]
              n350 = call "App enquece.vi"("command"=w756, "queue in"=w755) -> ("error out"=w757:errorcluster)  [unwired: 8 in, 1 out]
            }
            n351 = Merge Errors(w751, w749) -> (w750:errorcluster)
          }
          event "Test Channel 3": Value Change {
            n352 = event-data() -> ()  [unwired: 1 in, 1 out]
            n353 = Array Subset(array=w760, index=12, length=6) -> (w761:refnum<vi>[])
            n354 = for {
              tunnel: w761 -> [w772] mode=indexing
              n355 = property class="ColBox"(reference=w772, "Value"=u32 10000536 ("DRV 1")) -> ()  [unwired: 1 in, 2 out]
            }
            n356 = Build Array("Test Channel 3", "MEAS.AllRelaysOFF") -> (w767:string[])
            n357 = for {
              tunnel: [w776] -> w768 mode=indexing
              tunnel: w767 -> [w775] mode=indexing
              tunnel: w766 -> [w774]
              n358 = call "App enquece.vi"("command"=w775, "queue in"=w774) -> ("error out"=w776:errorcluster)  [unwired: 8 in, 1 out]
            }
            n359 = Merge Errors(w770, w768) -> (w769:errorcluster)
          }
          event "Test Channel 4": Value Change {
            n360 = event-data() -> ()  [unwired: 1 in, 1 out]
            n361 = Array Subset(array=w779, index=18, length=6) -> (w780:refnum<vi>[])
            n362 = for {
              tunnel: w780 -> [w791] mode=indexing
              n363 = property class="ColBox"(reference=w791, "Value"=u32 10000536 ("DRV 1")) -> ()  [unwired: 1 in, 2 out]
            }
            n364 = Build Array("Test Channel 4", "MEAS.AllRelaysOFF") -> (w786:string[])
            n365 = for {
              tunnel: [w795] -> w787 mode=indexing
              tunnel: w786 -> [w794] mode=indexing
              tunnel: w785 -> [w793]
              n366 = call "App enquece.vi"("command"=w794, "queue in"=w793) -> ("error out"=w795:errorcluster)  [unwired: 8 in, 1 out]
            }
            n367 = Merge Errors(w789, w787) -> (w788:errorcluster)
          }
          event "Test Channel 5": Value Change {
            n368 = event-data() -> ()  [unwired: 1 in, 1 out]
            n369 = Array Subset(array=w798, index=24, length=6) -> (w799:refnum<vi>[])
            n370 = for {
              tunnel: w799 -> [w810] mode=indexing
              n371 = property class="ColBox"(reference=w810, "Value"=u32 10000536 ("DRV 1")) -> ()  [unwired: 1 in, 2 out]
            }
            n372 = Build Array("Test Channel 5", "MEAS.AllRelaysOFF") -> (w805:string[])
            n373 = for {
              tunnel: [w814] -> w806 mode=indexing
              tunnel: w805 -> [w813] mode=indexing
              tunnel: w804 -> [w812]
              n374 = call "App enquece.vi"("command"=w813, "queue in"=w812) -> ("error out"=w814:errorcluster)  [unwired: 8 in, 1 out]
            }
            n375 = Merge Errors(w808, w806) -> (w807:errorcluster)
          }
          event "Test Channel 6": Value Change {
            n376 = event-data() -> ()  [unwired: 1 in, 1 out]
            n377 = Array Subset(array=w817, index=30, length=6) -> (w818:refnum<vi>[])
            n378 = for {
              tunnel: w818 -> [w829] mode=indexing
              n379 = property class="ColBox"(reference=w829, "Value"=u32 10000536 ("DRV 1")) -> ()  [unwired: 1 in, 2 out]
            }
            n380 = Build Array("Test Channel 6", "MEAS.AllRelaysOFF") -> (w824:string[])
            n381 = for {
              tunnel: [w833] -> w825 mode=indexing
              tunnel: w824 -> [w832] mode=indexing
              tunnel: w823 -> [w831]
              n382 = call "App enquece.vi"("command"=w832, "queue in"=w831) -> ("error out"=w833:errorcluster)  [unwired: 8 in, 1 out]
            }
            n383 = Merge Errors(w827, w825) -> (w826:errorcluster)
          }
          event "Test Channel 7": Value Change {
            n384 = event-data() -> ()  [unwired: 1 in, 1 out]
            n385 = Array Subset(array=w836, index=36, length=6) -> (w837:refnum<vi>[])
            n386 = for {
              tunnel: w837 -> [w848] mode=indexing
              n387 = property class="ColBox"(reference=w848, "Value"=u32 10000536 ("DRV 1")) -> ()  [unwired: 1 in, 2 out]
            }
            n388 = Build Array("Test Channel 7", "MEAS.AllRelaysOFF") -> (w844:string[])
            n389 = for {
              tunnel: [w852] -> w840 mode=indexing
              tunnel: w844 -> [w851] mode=indexing
              tunnel: w843 -> [w850]
              n390 = call "App enquece.vi"("command"=w851, "queue in"=w850) -> ("error out"=w852:errorcluster)  [unwired: 8 in, 1 out]
            }
            n391 = Merge Errors(w846, w840) -> (w845:errorcluster)
          }
          event "Test Channel 8": Value Change {
            n392 = event-data() -> ()  [unwired: 1 in, 1 out]
            n393 = Array Subset(array=w855, index=42, length=6) -> (w856:refnum<vi>[])
            n394 = for {
              tunnel: w856 -> [w867] mode=indexing
              n395 = property class="ColBox"(reference=w867, "Value"=u32 10000536 ("DRV 1")) -> ()  [unwired: 1 in, 2 out]
            }
            n396 = Build Array("Test Channel 8", "MEAS.AllRelaysOFF") -> (w862:string[])
            n397 = for {
              tunnel: [w871] -> w863 mode=indexing
              tunnel: w862 -> [w870] mode=indexing
              tunnel: w861 -> [w869]
              n398 = call "App enquece.vi"("command"=w870, "queue in"=w869) -> ("error out"=w871:errorcluster)  [unwired: 8 in, 1 out]
            }
            n399 = Merge Errors(w865, w863) -> (w864:errorcluster)
          }
          event "Test Channel 9": Value Change {
            n400 = event-data() -> ()  [unwired: 1 in, 1 out]
            n401 = Array Subset(array=w874, index=48, length=6) -> (w875:refnum<vi>[])
            n402 = for {
              tunnel: w875 -> [w886] mode=indexing
              n403 = property class="ColBox"(reference=w886, "Value"=u32 10000536 ("DRV 1")) -> ()  [unwired: 1 in, 2 out]
            }
            n404 = Build Array("Test Channel 9", "MEAS.AllRelaysOFF") -> (w881:string[])
            n405 = for {
              tunnel: [w890] -> w882 mode=indexing
              tunnel: w881 -> [w889] mode=indexing
              tunnel: w880 -> [w888]
              n406 = call "App enquece.vi"("command"=w889, "queue in"=w888) -> ("error out"=w890:errorcluster)  [unwired: 8 in, 1 out]
            }
            n407 = Merge Errors(w884, w882) -> (w883:errorcluster)
          }
          event "Test Channel 10": Value Change {
            n408 = event-data() -> ()  [unwired: 1 in, 1 out]
            n409 = Array Subset(array=w893, index=54, length=6) -> (w894:refnum<vi>[])
            n410 = for {
              tunnel: w894 -> [w905] mode=indexing
              n411 = property class="ColBox"(reference=w905, "Value"=u32 10000536 ("DRV 1")) -> ()  [unwired: 1 in, 2 out]
            }
            n412 = Build Array("Test Channel 10", "MEAS.AllRelaysOFF") -> (w900:string[])
            n413 = for {
              tunnel: [w909] -> w901 mode=indexing
              tunnel: w900 -> [w908] mode=indexing
              tunnel: w899 -> [w907]
              n414 = call "App enquece.vi"("command"=w908, "queue in"=w907) -> ("error out"=w909:errorcluster)  [unwired: 8 in, 1 out]
            }
            n415 = Merge Errors(w903, w901) -> (w902:errorcluster)
          }
          event User Event {
            n416 = event-data() -> ("Init?"=→"DC Measure Module" →"Inst. 1":bool)  [unwired: 1 in]
            n417 = disable-structure shown="LOGGING==TRUE" {
              disable-tunnel: w912 -> [w917 _]
              frame condition #0 (active) {
                n418 = Empty String/Path?(string/path=w917) -> (empty?=w924:bool)
                n419 = Select(t="Quece timeout", s=w924, f=w917) -> (s? t:f=w922:string)
                n420 = Format Into String(format string=":%s", initial string=w922, "DMM  Did  it") -> (resulting string=w919:string)  [unwired: 1 in, 1 out]
                n421 = call "string log (SubVI).vi"("Enum"=enum16{"Init", "Log", "Read"}."Log", "state Name"=w919) -> ()  [unwired: 8 in, 2 out]
              }
              frame condition #1 {
              }
            }
            n422 = disable-structure shown="DEBUGGING==TRUE" {
              disable-tunnel: [w925 w927] -> w914
              disable-tunnel: w913 -> [w925 w928]
              frame condition #0 (active) {
              }
              frame condition #1 {
                n423 = call "Show Panel.vi"() -> ("error out"=w926:errorcluster)  [unwired: 11 in]
                n424 = Merge Errors(w928, w926) -> (w927:errorcluster)
              }
            }
          }
          event User Event {
            n425 = event-data() -> ("Init?"=→"AC switches Module" →"Inst. 2":bool)  [unwired: 1 in]
            n426 = disable-structure shown="LOGGING==TRUE" {
              disable-tunnel: w933 -> [w940 _]
              frame condition #0 (active) {
                n427 = Empty String/Path?(string/path=w940) -> (empty?=w947:bool)
                n428 = Select(t="Quece timeout", s=w947, f=w940) -> (s? t:f=w945:string)
                n429 = Format Into String(format string=":%s", initial string=w945, "MB01  Did  it") -> (resulting string=w942:string)  [unwired: 1 in, 1 out]
                n430 = call "string log (SubVI).vi"("Enum"=enum16{"Init", "Log", "Read"}."Log", "state Name"=w942) -> ()  [unwired: 8 in, 2 out]
              }
              frame condition #1 {
              }
            }
            n431 = disable-structure shown="DEBUGGING==TRUE" {
              disable-tunnel: [w936 w939] -> w931
              disable-tunnel: w930 -> [w936 w938]
              frame condition #0 (active) {
              }
              frame condition #1 {
                n432 = call "Show Panel.vi"() -> ("error out"=w937:errorcluster)  [unwired: 11 in]
                n433 = Merge Errors(w938, w937) -> (w939:errorcluster)
              }
            }
          }
          event User Event {
            n434 = event-data() -> ("Init?"=→"DC Switches Module" →"Inst. 3":bool)  [unwired: 1 in]
            n435 = disable-structure shown="LOGGING==TRUE" {
              disable-tunnel: w950 -> [w955 _]
              frame condition #0 (active) {
                n436 = Empty String/Path?(string/path=w955) -> (empty?=w962:bool)
                n437 = Select(t="Quece timeout", s=w962, f=w955) -> (s? t:f=w960:string)
                n438 = Format Into String(format string=":%s", initial string=w960, "M054  Did  it") -> (resulting string=w957:string)  [unwired: 1 in, 1 out]
                n439 = call "string log (SubVI).vi"("Enum"=enum16{"Init", "Log", "Read"}."Log", "state Name"=w957) -> ()  [unwired: 8 in, 2 out]
              }
              frame condition #1 {
              }
            }
            n440 = disable-structure shown="DEBUGGING==TRUE" {
              disable-tunnel: w952 -> [w963 w965 w968]
              disable-tunnel: [w964 w965 w966] -> w951
              frame condition #0 (active) {
                n441 = Merge Errors(w963) -> (w964:errorcluster)
              }
              frame condition #1 {
              }
              frame condition #2 {
                n442 = call "Show Panel.vi"() -> ("error out"=w967:errorcluster)  [unwired: 11 in]
                n443 = Merge Errors(w968, w967) -> (w966:errorcluster)
              }
            }
          }
        }
      }
      frame "Apps.WaitingForTrigger" {
        n444 = call "App enquece.vi"("command"="MEAS.Read TRIGGER", "queue in"=w974) -> ("error out"=w972:errorcluster)  [unwired: 8 in, 1 out]
        n445 = Merge Errors(w970, w972) -> (w971:errorcluster)
      }
      frame "Apps.UpdateStatus" {
        n446 = disable-structure shown="LOGGING==TRUE" {
          disable-tunnel: w982 -> [w995 _]
          frame condition #0 (active) {
            n447 = Empty String/Path?(string/path=w995) -> (empty?=w998:bool)
            n448 = Select(t="Quece timeout", s=w998, f=w995) -> (s? t:f=w994:string)
            n449 = call "string log (SubVI).vi"("Enum"=enum16{"Init", "Log", "Read"}."Log", "state Name"=w994) -> ()  [unwired: 8 in, 2 out]
          }
          frame condition #1 {
          }
        }
        n450 = call "App enquece.vi"("command"="Apps.WaitForEvent", "queue in"=w990) -> ("error out"=w987:errorcluster)  [unwired: 8 in, 1 out]
        n451 = Merge Errors(w983, w987) -> (w984:errorcluster)
      }
      frame "Apps.UI Update" {
        w1002 = 6 ("length")
        n452 = disable-structure shown="LOGGING==TRUE" {
          disable-tunnel: w1010 -> [w1019 _]
          frame condition #0 (active) {
            n453 = Empty String/Path?(string/path=w1019) -> (empty?=w1022:bool)
            n454 = Select(t="Quece timeout", s=w1022, f=w1019) -> (s? t:f=w1018:string)
            n455 = call "string log (SubVI).vi"("Enum"=enum16{"Init", "Log", "Read"}."Log", "state Name"=w1018) -> ()  [unwired: 8 in, 2 out]
          }
          frame condition #1 {
          }
        }
        n456 = call "FGV Driver Data.vi"("DUT channel (1-11)"=w1005, "FGV enum"=FGV_DRV_data."Process" ("FGV DRV data enum")) -> ("60 DRV data"=w1003:T22[])  [unwired: 6 in, 3 out]
        n457 = Decrement(x=w1005) -> (x-1=w1006:i32)
        n458 = Multiply(x=w1006, y=w1002) -> (x*y=w1004:i32)
        n459 = Array Subset(array=w1008, index=w1004, length=w1002) -> (w1007:refnum<vi>[])
        n460 = Array Subset(array=w1003, index=w1004, length=w1002) -> (w1001:T22[])
        n461 = for {
          tunnel: w1007 -> [w1025] mode=indexing
          tunnel: w1001 -> [w1024] mode=indexing
          tunnel: [w1023] -> w1012 mode=indexing
          n462 = Unbundle By Name(w1024) -> ("DRV Fail/Pass (T)"=w1028:bool)
          n463 = Select(t=u32 16711686 ("DRV 1"), s=w1028, f=u32 65309 ("DRV 1")) -> (s? t:f=w1029:u32)
          n464 = property class="ColBox"(reference=w1025, "Value"=w1029) -> (error out=w1023:errorcluster)  [unwired: 1 in, 1 out]
        }
        n465 = Merge Errors(w1013, w1012) -> (w1014:errorcluster)
      }
      frame "Apps.UI Update 2" {
        n466 = disable-structure shown="LOGGING==TRUE" {
          disable-tunnel: w1035 -> [w1051 _]
          frame condition #0 (active) {
            n467 = Empty String/Path?(string/path=w1051) -> (empty?=w1054:bool)
            n468 = Select(t="Quece timeout", s=w1054, f=w1051) -> (s? t:f=w1050:string)
            n469 = call "string log (SubVI).vi"("Enum"=enum16{"Init", "Log", "Read"}."Log", "state Name"=w1050) -> ()  [unwired: 8 in, 2 out]
          }
          frame condition #1 {
          }
        }
        n470 = call "FGV Driver Data.vi"("FGV enum"=FGV_DRV_data."Read" ("FGV DRV data enum")) -> ("error out"=w1034:errorcluster, "60 DRV data"=w1031:T22[])  [unwired: 7 in, 2 out]
        n471 = for {
          tunnel: w1031 -> [w1056] mode=indexing
          tunnel: [w1055] -> w1041 mode=indexing
          n472 = Unbundle By Name(w1056) -> ("DRV Fail/Pass (T)"=w1055:bool)
        }
        n473 = Or Array Elements(Boolean array=w1041) -> (logical OR=w1039:bool)
        n474 = control-ref of="DRV 61"() -> (w1040:refnum<vi>)
        n475 = Select(t=u32 16711680 ("DRV 1"), s=w1039, f=u32 6618880 ("DRV 1")) -> (s? t:f=w1036:u32)
        n476 = property class="ColBox"(reference=w1040, error in=w1034, "Value"=w1036) -> (error out=w1032:errorcluster)  [unwired: 1 out]
        n477 = Merge Errors(w1049, w1032) -> (w1033:errorcluster)
      }
      frame "Apps.Exit" {
        w1061 = TRUE
        n478 = disable-structure shown="LOGGING==TRUE" {
          disable-tunnel: w1058 -> [w1076 _]
          frame condition #0 (active) {
            n479 = Empty String/Path?(string/path=w1076) -> (empty?=w1079:bool)
            n480 = Select(t="Quece timeout", s=w1079, f=w1076) -> (s? t:f=w1075:string)
            n481 = call "string log (SubVI).vi"("Enum"=enum16{"Init", "Log", "Read"}."Log", "state Name"=w1075) -> ()  [unwired: 8 in, 2 out]
          }
          frame condition #1 {
          }
        }
        n482 = call "Application Name--constant.vi"() -> ("Application Name"=w1062:string)  [unwired: 11 in]
        n483 = call "Stop Module.vi"("Wait for Module to stop? (F)"=w1061, "Origin"=w1062, "Module ID"=-1) -> ("error out"=w1064:errorcluster)  [unwired: 8 in]
        n484 = call "Stop Module.vi"("Wait for Module to Stop? (F)"=w1061, "Origin"=w1062) -> ("error out"=w1070:errorcluster)  [unwired: 9 in]
        n485 = call "Stop Module.vi"("Wait for Module to Stop? (F)"=w1061, "Origin"=w1062) -> ("error out"=w1069:errorcluster)  [unwired: 9 in]
        n486 = call "Stop Module.vi"("Wait for Module to Stop? (F)"=w1061, "Origin"=w1062) -> ("error out"=w1068:errorcluster)  [unwired: 9 in]
        n487 = Merge Errors(w1066, w1070, w1069, w1068, w1064) -> (w1067:errorcluster)
      }
      frame "Apps.Error Handler" {
        w1088 = TRUE  # Priority Enquece
        n488 = disable-structure shown="LOGGING==TRUE" {
          disable-tunnel: w1081 -> [w1097 _]
          frame condition #0 (active) {
            n489 = Empty String/Path?(string/path=w1097) -> (empty?=w1100:bool)
            n490 = Select(t="Quece timeout", s=w1100, f=w1097) -> (s? t:f=w1096:string)
            n491 = call "string log (SubVI).vi"("Enum"=enum16{"Init", "Log", "Read"}."Log", "state Name"=w1096) -> ()  [unwired: 8 in, 2 out]
          }
          frame condition #1 {
          }
        }
        n492 = call <vilib>:"Simple Error Handler.vi"("error in (no error)"=w1095) -> ("error out"=w1090:errorcluster)  [unwired: 4 in, 4 out]
        n493 = flat-sequence {
          tunnel: w1090 -> [_]
          tunnel: [w1101] -> w1082
          frame #0 {
            n494 = xnode "Error Ring"() -> ("error out"=w1101:errorcluster)
          }
        }
        n495 = call "App enquece.vi"("Priority Enquece"=w1088, "command"="Apps.Exit", "queue in"=w1089) -> ("error out"=w1087:errorcluster)  [unwired: 7 in, 1 out]
        n496 = Merge Errors(w1082, w1087) -> (w1083:errorcluster)
      }
      frame "INIT.Init FGV" {
        n497 = call "FGV_HoldingRegs.vi"("FGV_enum"=FGV_enum."Init FGV") -> ("error out"=w1106:errorcluster)  [unwired: 8 in, 2 out]
        n498 = local write "EMIC connected"(bool[] [FALSE, FALSE, FALSE, FALSE, FALSE, FALSE] ("Array")) -> ()
        n499 = local write "Auto/Man"(FALSE) -> ()
        n500 = call "FGV Driver Data.vi"("error in (no error)"=w1106, "FGV enum"=FGV_DRV_data."Init" ("FGV DRV data enum")) -> ("error out"=w1104:errorcluster)  [unwired: 6 in, 3 out]
        n501 = Merge Errors(w1117, w1104) -> (w1105:errorcluster)
      }
      frame "INIT.Read HW config" {
        n502 = disable-structure shown="LOGGING==TRUE" {
          disable-tunnel: w1120 -> [w1163 _]
          frame condition #0 (active) {
            n503 = Empty String/Path?(string/path=w1163) -> (empty?=w1166:bool)
            n504 = Select(t="Quece timeout", s=w1166, f=w1163) -> (s? t:f=w1162:string)
            n505 = call "string log (SubVI).vi"("Enum"=enum16{"Init", "Log", "Read"}."Log", "state Name"=w1162) -> ()  [unwired: 8 in, 2 out]
          }
          frame condition #1 {
          }
        }
        n506 = call "HW Config.vi"() -> ("error out"=w1121:errorcluster, "HW config 2"=w1129:T8)  [unwired: 10 in]
        n507 = Bundle By Name(cluster=w1130, "HW config 2"=w1129) -> (w1128:cluster{"HW config 2":T8})
        n508 = disable-structure shown="Enabled" {
          disable-tunnel: w1123 -> [w1136 _]
          disable-tunnel: [w1135 w1161] -> w1122
          disable-tunnel: w1121 -> [w1134 w1161]
          frame Enabled {
            n509 = invoke class="VI" method="FP.Open"(error in=w1134, "State"=T15."Minimized") -> (error out=w1137:errorcluster)  [unwired: 3 in, 4 out]
            n510 = disable-structure shown="Disabled" {
              disable-tunnel: [w1143 TRUE ("Login Successed")] -> w1140
              disable-tunnel: [w1142 w1150] -> w1139
              disable-tunnel: w1137 -> [w1141 w1150]
              frame Disabled {
                n511 = disable-structure shown="Default" {
                  disable-tunnel: [w1146 TRUE ("Login Successed")] -> w1143
                  disable-tunnel: [w1145 w1148] -> w1142
                  disable-tunnel: w1141 -> [w1144 w1148]
                  frame condition #0 {
                    n512 = call "Login.vi"("error in (no error)"=w1144) -> ("error out"=w1145:errorcluster, "Login Successed"=w1146:bool)  [unwired: 9 in]
                  }
                  frame condition #1 (active) {
                  }
                }
              }
              frame Enabled {
              }
            }
            n513 = case shown="True" w1140 {
              tunnel: w1136 -> [w1157 _]
              tunnel: w1139 -> [w1154 w1159]
              tunnel: [w1153 w1160] -> w1135
              frame False {
                n514 = call "string log (SubVI).vi"("Enum"=enum16{"Init", "Log", "Read"}."Init") -> ("error out"=w1151:errorcluster)  [unwired: 9 in, 1 out]
                n515 = call "App enquece.vi"("Priority Enquece"=TRUE, "error in (no error)"=w1154, "command"="Apps.Exit", "queue in"=w1157) -> ("error out"=w1153:errorcluster)  [unwired: 6 in, 1 out]
                n516 = call "inst.InitialiseFGV.vi"("error in (no error)"=w1151) -> ()  [unwired: 10 in, 1 out]
              }
              frame True {
                n517 = invoke class="VI" method="FP.Open"(error in=w1159, "State"=T15."Standard") -> (error out=w1160:errorcluster)  [unwired: 3 in, 4 out]
              }
            }
          }
          frame Disabled {
          }
        }
        n518 = Merge Errors(w1133, w1122) -> (w1124:errorcluster)
        "version" <- "Development" ("version")
      }
      frame "INIT.Read DRV code" {
        w1184 = u8 2 items=["SLOW", "MID", "FAST"] ("Detector Rate")
        # "Convert from [mA] to [A]"
        n519 = flat-sequence {
          tunnel: [w1210] -> w1173
          tunnel: [w1205] -> w1167
          frame #0 {
            n520 = invoke class="VI" method="FP.Open"("State"=T15."Hidden") -> (error out=w1208:errorcluster)  [unwired: 4 in, 4 out]
            n521 = call "ReadDriverParameters.vi"("error in (no error)"=w1208) -> ("error out"=w1206:errorcluster, "DRV stand"=w1210:T1)  [unwired: 9 in]
            n522 = invoke class="VI" method="FP.Open"(error in=w1206, "State"=T15."Standard") -> (error out=w1205:errorcluster)  [unwired: 3 in, 4 out]
          }
        }
        n523 = disable-structure shown="LOGGING==TRUE" {
          disable-tunnel: w1196 -> [w1212 _]
          frame condition #0 (active) {
            n524 = Empty String/Path?(string/path=w1212) -> (empty?=w1215:bool)
            n525 = Select(t="Quece timeout", s=w1215, f=w1212) -> (s? t:f=w1211:string)
            n526 = call "string log (SubVI).vi"("Enum"=enum16{"Init", "Log", "Read"}."Log", "state Name"=w1211) -> ()  [unwired: 8 in, 2 out]
          }
          frame condition #1 {
          }
        }
        n527 = call "FGV DRV stand.vi"("Enum"=enum16{"Write", "Read"}."Write", "DRV stand  in"=w1173) -> ("DRV stand out"=w1170:T1)  [unwired: 9 in]
        "DRV stand" <- w1170
        n528 = Merge Errors(w1197, w1167) -> (w1198:errorcluster)
        n529 = Unbundle By Name(w1173) -> ("DC characteristics.Voltage.Max"=w1195:dbl, "DC characteristics.Current.Max"=w1194:dbl)
        n530 = Unbundle By Name(w1170) -> ("SAP ID"=→"SAP ID":string, "Name"=→"Name":string)
        n531 = Divide(x=w1194, y=1000.0) -> (x/y=w1192:dbl)
        n532 = call "Select DMM voltage range.vi"("Max"=w1195) -> ("DDM voltage Range"=w1186:dbl)  [unwired: 9 in, 1 out]
        n533 = call "Select DMM Current Range.vi"("Max"=w1192) -> ("1A/10A?"=w1174:bool, "DMM current range"=w1185:dbl)  [unwired: 8 in, 1 out]
        n534 = Bundle By Name(cluster=T16 {"DMM config cluster"={"DCV range"=0.0, "DCI range"=0.0, "Detector Rate"=0}, "mux2-1(DMM I) encode"=enum."DMM I (0.5)"} ("DMM all config"), "DMM config cluster.DCV range"=w1186, "DMM config cluster.DCI range"=w1185, "DMM config cluster.Detector Rate"=w1184) -> (w1190:T16)
        n535 = Select(t=enum16{"DMM I (0.5)", "DMM I (12)"}."DMM I (12)" ("mux2-1(DMM I) encode 2"), s=w1174, f=enum16{"DMM I (0.5)", "DMM I (12)"}."DMM I (0.5)" ("mux2-1(DMM I) encode 2")) -> (s? t:f=w1179:enum16{"DMM I (0.5)", "DMM I (12)"})
        n536 = To Variant(anything=w1179) -> (Variant=w1181:variant)
        n537 = To Variant(anything=w1190) -> (Variant=w1189:variant)
        n538 = call "App enquece.vi"("command data"=w1189, "command"="INIT.Set DMM config", "queue in"=w1187) -> ("error out"=w1176:errorcluster, "Queue out"=w1180:refnum<queue>)  [unwired: 7 in]
        n539 = call "App enquece.vi"("error in (no error)"=w1176, "command data"=w1181, "command"="MEAS.Set Input Current", "queue in"=w1180) -> ("error out"=w1175:errorcluster)  [unwired: 6 in, 1 out]
        n540 = Merge Errors(w1198, w1175) -> (w1183:errorcluster)
      }
      frame "INIT.Call DMM module" {
        n541 = disable-structure shown="LOGGING==TRUE" {
          disable-tunnel: w1217 -> [w1235 _]
          frame condition #0 (active) {
            n542 = Empty String/Path?(string/path=w1235) -> (empty?=w1238:bool)
            n543 = Select(t="Quece timeout", s=w1238, f=w1235) -> (s? t:f=w1234:string)
            n544 = call "string log (SubVI).vi"("Enum"=enum16{"Init", "Log", "Read"}."Log", "state Name"=w1234) -> ()  [unwired: 8 in, 2 out]
          }
          frame condition #1 {
          }
        }
        n545 = Unbundle By Name(w1228) -> ("HW config 2.DMM"=w1227:string)
        n546 = Type Cast(type=refnum<visa-resource-name> refnum ("VISA resource name 2"), x=w1227) -> (*(type *) &x=w1225:refnum<visa-resource-name>)
        n547 = call "Start Module.vi"("VISA resource name 2"=w1225) -> ("error out"=w1230:errorcluster, "Wait for Event Sync?"=w1224:bool, "DMM Module Broadcast Events"=w1223:T14)  [unwired: 7 in, 1 out]
        n548 = register-events(reference=w1231, w1223) -> (reference out=w1232:refnum<event-registration>)  [unwired: 5 in, 1 out]
        n549 = call "Synchronize Module Events.vi"("error in"=w1230, "Wait for Event Sync?"=w1224) -> ("error out"=w1229:errorcluster)  [unwired: 9 in]
        n550 = Merge Errors(w1218, w1229) -> (w1219:errorcluster)
      }
      frame "INIT.Call MUX module" {
        n551 = disable-structure shown="LOGGING==TRUE" {
          disable-tunnel: w1240 -> [w1258 _]
          frame condition #0 (active) {
            n552 = Empty String/Path?(string/path=w1258) -> (empty?=w1261:bool)
            n553 = Select(t="Quece timeout", s=w1261, f=w1258) -> (s? t:f=w1257:string)
            n554 = call "string log (SubVI).vi"("Enum"=enum16{"Init", "Log", "Read"}."Log", "state Name"=w1257) -> ()  [unwired: 8 in, 2 out]
          }
          frame condition #1 {
          }
        }
        n555 = Unbundle By Name(w1252) -> ("HW config 2.mux"=w1251:string)
        n556 = Type Cast(type=refnum<visa-resource-name> refnum ("VISA resource name"), x=w1251) -> (*(type *) &x=w1250:refnum<visa-resource-name>)
        n557 = call "Start Module.vi"("VISA resource name"=w1250) -> ("error out"=w1253:errorcluster, "Wait for Event Sync?"=w1247:bool, "Switches Module Broadcast Events"=w1248:T12)  [unwired: 7 in, 1 out]
        n558 = register-events(reference=w1254, w1248) -> (reference out=w1255:refnum<event-registration>)  [unwired: 5 in, 1 out]
        n559 = call "Synchronize Module Events.vi"("error in"=w1253, "Wait for Event Sync?"=w1247) -> ("error out"=w1246:errorcluster)  [unwired: 9 in]
        n560 = Merge Errors(w1241, w1246) -> (w1242:errorcluster)
      }
      frame "INIT.Call DEMUX module" {
        n561 = disable-structure shown="LOGGING==TRUE" {
          disable-tunnel: w1263 -> [w1281 _]
          frame condition #0 (active) {
            n562 = Empty String/Path?(string/path=w1281) -> (empty?=w1284:bool)
            n563 = Select(t="Quece timeout", s=w1284, f=w1281) -> (s? t:f=w1280:string)
            n564 = call "string log (SubVI).vi"("Enum"=enum16{"Init", "Log", "Read"}."Log", "state Name"=w1280) -> ()  [unwired: 8 in, 2 out]
          }
          frame condition #1 {
          }
        }
        n565 = Unbundle By Name(w1274) -> ("HW config 2.demux"=w1273:string)
        n566 = Type Cast(type=refnum<visa-resource-name> refnum ("COMport name"), x=w1273) -> (*(type *) &x=w1272:refnum<visa-resource-name>)
        n567 = call "Start Module.vi"("COMport name"=w1272) -> ("error out"=w1275:errorcluster, "Wait for Event Sync?"=w1276:bool, "MB 01 switches Module Broadcast Events"=w1270:T13)  [unwired: 7 in, 1 out]
        n568 = register-events(reference=w1277, w1270) -> (reference out=w1278:refnum<event-registration>)  [unwired: 5 in, 1 out]
        n569 = call "Synchronize Module Events.vi"("error in"=w1275, "Wait for Event Sync?"=w1276) -> ("error out"=w1269:errorcluster)  [unwired: 9 in]
        n570 = Merge Errors(w1264, w1269) -> (w1265:errorcluster)
      }
      frame "INIT.Call EMIC modules" {
        n571 = disable-structure shown="LOGGING==TRUE" {
          disable-tunnel: w1288 -> [w1305 _]
          frame condition #0 (active) {
            n572 = Empty String/Path?(string/path=w1305) -> (empty?=w1308:bool)
            n573 = Select(t="Quece timeout", s=w1308, f=w1305) -> (s? t:f=w1304:string)
            n574 = call "string log (SubVI).vi"("Enum"=enum16{"Init", "Log", "Read"}."Log", "state Name"=w1304) -> ()  [unwired: 8 in, 2 out]
          }
          frame condition #1 {
          }
        }
        n575 = Unbundle By Name(w1295) -> ("HW config 2.eMIC1"=w1302:string, "HW config 2.eMIC2"=w1301:string, "HW config 2.eMIC3"=w1300:string, "HW config 2.eMIC4"=w1299:string, "HW config 2.eMIC5"=w1298:string, "HW config 2.eMIC6"=w1297:string)
        n576 = Build Array(w1302, w1301, w1300, w1299, w1298, w1297) -> (w1286:string[])
        n577 = for {
          shift-right: [w1318] -> w1294
          shift-left: w1296 -> [w1316]
          tunnel: w1286 -> [w1317] mode=indexing
          tunnel: [w1310] -> w1292 mode=indexing
          n578 = Type Cast(type=refnum<visa-resource-name> refnum ("VISA resource name"), x=w1317) -> (*(type *) &x=w1314:refnum<visa-resource-name>)
          n579 = call "Start Module.vi"("VISA resource name"=w1314) -> ("error out"=w1311:errorcluster, "Wait for Event Sync?"=w1309:bool, "CE14_v2 Broadcast Events"=w1313:T11, "Module ID"=w1312:i32)  [unwired: 7 in]
          n580 = register-events(reference=w1316, w1313) -> (reference out=w1318:refnum<event-registration>)  [unwired: 5 in, 1 out]
          n581 = call "Synchronize Module Events.vi"("error in"=w1311, "Wait for Event Sync?"=w1309, "Module ID in"=w1312) -> ("error out"=w1310:errorcluster)  [unwired: 7 in, 1 out]
        }
        n582 = Merge Errors(w1289, w1292) -> (w1287:errorcluster)
      }
      frame "INIT.Open COM DMM" {
        n583 = disable-structure shown="LOGGING==TRUE" {
          disable-tunnel: w1322 -> [w1334 _]
          frame condition #0 (active) {
            n584 = Empty String/Path?(string/path=w1334) -> (empty?=w1337:bool)
            n585 = Select(t="Quece timeout", s=w1337, f=w1334) -> (s? t:f=w1333:string)
            n586 = call "string log (SubVI).vi"("Enum"=enum16{"Init", "Log", "Read"}."Log", "state Name"=w1333) -> ()  [unwired: 8 in, 2 out]
          }
          frame condition #1 {
          }
        }
        n587 = call "DMM connect and reset.vi"() -> ("error out"=w1326:errorcluster)  [unwired: 11 in]
        n588 = Merge Errors(w1323, w1326) -> (w1320:errorcluster)
        n589 = flat-sequence {
          tunnel: [w1332] -> w1321
          tunnel: w1320 -> [w1332]
          frame #0 {
            n590 = Wait (ms)(milliseconds to wait=u32 70) -> ()  [unwired: 1 out]
          }
        }
      }
      frame "INIT.Open COM MUX" {
        n591 = disable-structure shown="LOGGING==TRUE" {
          disable-tunnel: w1341 -> [w1353 _]
          frame condition #0 (active) {
            n592 = Empty String/Path?(string/path=w1353) -> (empty?=w1356:bool)
            n593 = Select(t="Quece timeout", s=w1356, f=w1353) -> (s? t:f=w1352:string)
            n594 = call "string log (SubVI).vi"("Enum"=enum16{"Init", "Log", "Read"}."Log", "state Name"=w1352) -> ()  [unwired: 8 in, 2 out]
          }
          frame condition #1 {
          }
        }
        n595 = call "inst.Open.vi"() -> ("error out"=w1347:errorcluster)  [unwired: 11 in]
        n596 = Merge Errors(w1342, w1347) -> (w1339:errorcluster)
        n597 = flat-sequence {
          tunnel: [w1351] -> w1340
          tunnel: w1339 -> [w1351]
          frame #0 {
            n598 = Wait (ms)(milliseconds to wait=u32 70) -> ()  [unwired: 1 out]
          }
        }
      }
      frame "INIT.Open COM DEMUX" {
        n599 = disable-structure shown="LOGGING==TRUE" {
          disable-tunnel: w1360 -> [w1372 _]
          frame condition #0 (active) {
            n600 = Empty String/Path?(string/path=w1372) -> (empty?=w1375:bool)
            n601 = Select(t="Quece timeout", s=w1375, f=w1372) -> (s? t:f=w1371:string)
            n602 = call "string log (SubVI).vi"("Enum"=enum16{"Init", "Log", "Read"}."Log", "state Name"=w1371) -> ()  [unwired: 8 in, 2 out]
          }
          frame condition #1 {
          }
        }
        n603 = call "MB01 Open.vi"() -> ("error out"=w1365:errorcluster)  [unwired: 11 in]
        n604 = Merge Errors(w1361, w1365) -> (w1358:errorcluster)
        n605 = flat-sequence {
          tunnel: [w1370] -> w1359
          tunnel: w1358 -> [w1370]
          frame #0 {
            n606 = Wait (ms)(milliseconds to wait=u32 70) -> ()  [unwired: 1 out]
          }
        }
      }
      frame "INIT.Open COM EMIC" {
        n607 = disable-structure shown="LOGGING==TRUE" {
          disable-tunnel: w1379 -> [w1392 _]
          frame condition #0 (active) {
            n608 = Empty String/Path?(string/path=w1392) -> (empty?=w1395:bool)
            n609 = Select(t="Quece timeout", s=w1395, f=w1392) -> (s? t:f=w1391:string)
            n610 = call "string log (SubVI).vi"("Enum"=enum16{"Init", "Log", "Read"}."Log", "state Name"=w1391) -> ()  [unwired: 8 in, 2 out]
          }
          frame condition #1 {
          }
        }
        n611 = call "Connect to CE14.vi"("Module ID"=-1) -> ("error out"=w1384:errorcluster)  [unwired: 10 in]
        n612 = Merge Errors(w1380, w1384) -> (w1377:errorcluster)
        n613 = flat-sequence {
          tunnel: [w1390] -> w1378
          tunnel: w1377 -> [w1390]
          frame #0 {
            n614 = Wait (ms)(milliseconds to wait=u32 70) -> ()  [unwired: 1 out]
          }
        }
      }
      frame "MEAS.Read EMIC connected" {
        n615 = disable-structure shown="LOGGING==TRUE" {
          disable-tunnel: w1408 -> [w1421 _]
          frame condition #0 (active) {
            n616 = Empty String/Path?(string/path=w1421) -> (empty?=w1424:bool)
            n617 = Select(t="Quece timeout", s=w1424, f=w1421) -> (s? t:f=w1420:string)
            n618 = call "string log (SubVI).vi"("Enum"=enum16{"Init", "Log", "Read"}."Log", "state Name"=w1420) -> ()  [unwired: 8 in, 2 out]
          }
          frame condition #1 {
          }
        }
        n619 = for {
          N: 6 -> [_]
          tunnel: [w1427] -> w1406 mode=indexing
          tunnel: [w1426] -> w1412 mode=indexing
          i -> [w1429]
          n620 = Increment(x=w1429) -> (x+1=w1428:i32)
          n621 = Wait (ms)(milliseconds to wait=u32 50) -> ()  [unwired: 1 out]
          n622 = call "CE14.CheckConnected.vi"("Module ID"=w1428) -> ("error out"=w1426:errorcluster, "Success"=w1427:bool)  [unwired: 8 in, 1 out]
        }
        "EMIC connected" <- w1406
        n623 = local read "CE14  Module did it"() -> (w1407:bool[])
        n624 = And(x=w1407, y=w1406) -> (x .and. y?=w1405:bool[])
        n625 = Merge Errors(w1411, w1412) -> (w1397:errorcluster)
        n626 = Index Array(array=w1405) -> (element #1=→"Inst. 4":bool, element #2=→"Inst. 5":bool, element #3=→"Inst. 6":bool, element #4=→"Inst. 7":bool, element #5=→"Inst. 8":bool, element #6=→"Inst. 9":bool)  [unwired: 9 in, 3 out]
        n627 = flat-sequence {
          tunnel: [w1418] -> w1398
          tunnel: w1397 -> [w1418]
          frame #0 {
            n628 = Wait (ms)(milliseconds to wait=u32 70) -> ()  [unwired: 1 out]
          }
        }
      }
      frame "MEAS.Set DMM config" {
        n629 = disable-structure shown="LOGGING==TRUE" {
          disable-tunnel: w1433 -> [w1452 _]
          frame condition #0 (active) {
            n630 = Empty String/Path?(string/path=w1452) -> (empty?=w1455:bool)
            n631 = Select(t="Quece timeout", s=w1455, f=w1452) -> (s? t:f=w1451:string)
            n632 = call "string log (SubVI).vi"("Enum"=enum16{"Init", "Log", "Read"}."Log", "state Name"=w1451) -> ()  [unwired: 8 in, 2 out]
          }
          frame condition #1 {
          }
        }
        n633 = Variant To Data(type=T16 {"DMM config cluster"={"DCV range"=0.0, "DCI range"=0.0, "Detector Rate"=0}, "mux2-1(DMM I) encode"=enum."DMM I (0.5)"} ("DMM all config"), Variant=w1445) -> (data=w1443:T16)  [unwired: 1 in, 1 out]
        n634 = Unbundle By Name(w1443) -> ("DMM config cluster"=w1442:T17)
        n635 = Unbundle By Name(w1442) -> ("DCV range"=w1441:dbl, "DCI range"=w1440:dbl, "Detector Rate"=w1439:u8)
        n636 = call "config channel.vi"("Detector Rate"=w1439, "DCI range"=w1440, "DCV range"=w1441) -> ("error out"=w1437:errorcluster)  [unwired: 8 in]
        n637 = Merge Errors(w1434, w1437) -> (w1431:errorcluster)
        n638 = flat-sequence {
          tunnel: [w1450] -> w1432
          tunnel: w1431 -> [w1450]
          frame #0 {
            n639 = Wait (ms)(milliseconds to wait=u32 70) -> ()  [unwired: 1 out]
          }
        }
      }
      frame "MEAS.AllRelaysOFF" {
        n640 = disable-structure shown="LOGGING==TRUE" {
          disable-tunnel: w1457 -> [w1470 _]
          frame condition #0 (active) {
            n641 = Empty String/Path?(string/path=w1470) -> (empty?=w1473:bool)
            n642 = Select(t="Quece timeout", s=w1473, f=w1470) -> (s? t:f=w1469:string)
            n643 = call "string log (SubVI).vi"("Enum"=enum16{"Init", "Log", "Read"}."Log", "state Name"=w1469) -> ()  [unwired: 8 in, 2 out]
          }
          frame condition #1 {
          }
        }
        n644 = for {
          N: 5 -> [_]
          tunnel: [w1476] -> w1464 mode=indexing
          i -> [w1478]
          n645 = case shown="4" w1478 {
            tunnel: [w1482 w1483 w1484 w1485 w1486 _] -> w1476
            frame 0 {
              # "eMIC"
              n646 = Initialize Array(FALSE, 6 ("dimension size")) -> (w1479:bool[])
              n647 = call "MB01_eMICs.vi"("Array"=w1479) -> ("error out"=w1482:errorcluster)  [unwired: 10 in]
            }
            frame 1 {
              # "demux 1-10 (AC)"
              n648 = call "demux1-10_chan0.vi"() -> ("error out"=w1483:errorcluster)  [unwired: 11 in]
            }
            frame 2 {
              # "5V for  Shorted Circuit"
              n649 = call "SC enable OFF.vi"() -> ("error out"=w1484:errorcluster)  [unwired: 11 in]
            }
            frame 3 {
              # "mux 10-1 (DC)"
              n650 = call "mux10-1_chan0.vi"() -> ("error out"=w1485:errorcluster)  [unwired: 11 in]
            }
            frame 4 {
              # "mux 6-1 3wires (DMM)"
              n651 = call "mux6-1_chan0.vi"() -> ("error out"=w1486:errorcluster)  [unwired: 11 in]
            }
            frame 5.., Default {
            }
          }
          n652 = Wait (ms)(milliseconds to wait=u32 100) -> ()  [unwired: 1 out]
        }
        n653 = Merge Errors(w1458, w1464) -> (w1459:errorcluster)
        n654 = flat-sequence {
          tunnel: [w1474] -> w1460
          tunnel: w1459 -> [w1474]
          frame #0 {
            n655 = Wait (ms)(milliseconds to wait=u32 100) -> ()  [unwired: 1 out]
          }
        }
      }
      frame "MEAS.Read TRIGGER" {
        w1498 = T9 {"new board?"=TRUE, "new trigger"=TRUE, "last trigger"=TRUE}  # trigger infor
        # "JIG locked - rising-edge happens"
        n656 = disable-structure shown="LOGGING==TRUE" {
          disable-tunnel: w1502 -> [w1516 _]
          frame condition #0 (active) {
            n657 = Empty String/Path?(string/path=w1516) -> (empty?=w1519:bool)
            n658 = Select(t="Quece timeout", s=w1519, f=w1516) -> (s? t:f=w1515:string)
            n659 = call "string log (SubVI).vi"("Enum"=enum16{"Init", "Log", "Read"}."Log", "state Name"=w1515) -> ()  [unwired: 8 in, 2 out]
          }
          frame condition #1 {
          }
        }
        n660 = call "Read JIG trigger.vi"() -> ("error out"=w1506:errorcluster, "Trigger?"=w1487:bool)  [unwired: 9 in, 1 out]
        "trigger Value" <- w1487
        n661 = feedback-in #3(w1487) -> ()
        n662 = feedback #3(FALSE) -> (w1495:bool)
        n663 = Greater?(x=w1487, y=w1495) -> (0:w1489:bool)
        n664 = Bundle By Name(cluster=w1498, "new board?"=w1489, "new trigger"=w1487, "last trigger"=w1495) -> (w1497:T9)
        n665 = Select(t=-1, s=w1489, f=w1492) -> (s? t:f=w1493:i32)
        n666 = And(x="Auto/Man", y=w1489) -> (x .and. y?=w1488:bool)
        n667 = local write "new Trigger?"(w1487) -> ()
        n668 = local write "New board?"(w1489) -> ()
        n669 = local write "last Trigger?"(w1495) -> ()
        n670 = Merge Errors(w1505, w1506) -> (w1503:errorcluster)
        n671 = case shown="True" w1488 {
          tunnel: w1499 -> [_ w1514]
          tunnel: w1497 -> [_ w1513]
          tunnel: [_ w1512] -> w1496
          frame False {
          }
          frame True {
            n672 = Generate User Event(user event=w1514, event data cluster=w1513) -> (error out=w1512:errorcluster)  [unwired: 2 in, 1 out]
          }
        }
        n673 = Merge Errors(w1503, w1496) -> (w1500:errorcluster)
        n674 = flat-sequence {
          tunnel: [w1520] -> w1504
          tunnel: w1500 -> [w1520]
          frame #0 {
            n675 = Wait (ms)(milliseconds to wait=u32 70) -> ()  [unwired: 1 out]
          }
        }
      }
      frame "MEAS.Set Input Current" {
        n676 = disable-structure shown="LOGGING==TRUE" {
          disable-tunnel: w1523 -> [w1538 _]
          frame condition #0 (active) {
            n677 = Empty String/Path?(string/path=w1538) -> (empty?=w1541:bool)
            n678 = Select(t="Quece timeout", s=w1541, f=w1538) -> (s? t:f=w1537:string)
            n679 = call "string log (SubVI).vi"("Enum"=enum16{"Init", "Log", "Read"}."Log", "state Name"=w1537) -> ()  [unwired: 8 in, 2 out]
          }
          frame condition #1 {
          }
        }
        n680 = Variant To Data(type=enum16{"DMM I (0.5)", "DMM I (12)"}."DMM I (0.5)" ("mux2-1(DMM I) encode"), Variant=w1531) -> (data=w1530:enum16{"DMM I (0.5)", "DMM I (12)"})  [unwired: 1 in, 1 out]
        n681 = call "DMM I 0.5_10.vi"("mux2-1(DMM I) encode"=w1530) -> ("error out"=w1533:errorcluster)  [unwired: 10 in]
        n682 = Merge Errors(w1526, w1533) -> (w1524:errorcluster)
        n683 = flat-sequence {
          tunnel: [w1542] -> w1525
          tunnel: w1524 -> [w1542]
          frame #0 {
            n684 = Wait (ms)(milliseconds to wait=u32 70) -> ()  [unwired: 1 out]
          }
        }
      }
      frame "MEAS.Read Optos" {
        n685 = disable-structure shown="LOGGING==TRUE" {
          disable-tunnel: w1547 -> [w1572 _]
          frame condition #0 (active) {
            n686 = Empty String/Path?(string/path=w1572) -> (empty?=w1575:bool)
            n687 = Select(t="Quece timeout", s=w1575, f=w1572) -> (s? t:f=w1571:string)
            n688 = call "string log (SubVI).vi"("Enum"=enum16{"Init", "Log", "Read"}."Log", "state Name"=w1571) -> ()  [unwired: 8 in, 2 out]
          }
          frame condition #1 {
          }
        }
        n689 = flat-sequence {
          tunnel: [w1561] -> w1545
          frame #0 {
            n690 = Initialize Array(FALSE, 6 ("dimension size"), 10 ("dimension size")) -> (w1557:bool[][])
            n691 = Wait (ms)(milliseconds to wait=u32 100) -> ()  [unwired: 1 out]
            n692 = local write "Short DRV"(w1557) -> ()
          }
          frame #1 {
            n693 = call "inst.Optos.vi"() -> ("error out"=w1570:errorcluster, "Optos"=w1568:bool[])  [unwired: 9 in, 1 out]
            n694 = Reshape Array(w1568, 10 ("dimension size"), 6 ("dimension size")) -> (w1566:bool[][])
            n695 = To Variant(anything=w1568) -> (Variant=w1569:variant)
            n696 = Transpose 2D Array(2D array=w1566) -> (transposed array=→"Short DRV":bool[][])
            n697 = call "FGV Driver Data.vi"("Mode"=DUT_data_Mode."Short Circuits", "error in (no error)"=w1570, "FGV enum"=FGV_DRV_data."Write" ("FGV DRV data enum"), "data"=w1569) -> ("error out"=w1561:errorcluster)  [unwired: 4 in, 3 out]
          }
        }
        n698 = Merge Errors(w1546, w1545) -> (w1548:errorcluster)
        n699 = flat-sequence {
          tunnel: [w1576] -> w1549
          tunnel: w1548 -> [w1576]
          frame #0 {
            n700 = Wait (ms)(milliseconds to wait=u32 70) -> ()  [unwired: 1 out]
          }
        }
      }
      frame "MEAS.Reset JIG" {
        n701 = disable-structure shown="Disabled" {
          disable-tunnel: w1578 -> [w1592 _]
          frame Disabled {
            n702 = call "reset DRV UI (SubVI).vi"("Ref  in"=w1592) -> ()  [unwired: 9 in, 2 out]
          }
          frame Enabled {
          }
        }
        n703 = disable-structure shown="LOGGING==TRUE" {
          disable-tunnel: w1582 -> [w1594 _]
          frame condition #0 (active) {
            n704 = Empty String/Path?(string/path=w1594) -> (empty?=w1597:bool)
            n705 = Select(t="Quece timeout", s=w1597, f=w1594) -> (s? t:f=w1593:string)
            n706 = call "string log (SubVI).vi"("Enum"=enum16{"Init", "Log", "Read"}."Log", "state Name"=w1593) -> ()  [unwired: 8 in, 2 out]
          }
          frame condition #1 {
          }
        }
        n707 = call "JIG Reset.vi"() -> ("error out"=w1588:errorcluster)  [unwired: 11 in]
        n708 = Merge Errors(w1584, w1588) -> (w1580:errorcluster)
        n709 = flat-sequence {
          tunnel: w1580 -> [w1598]
          tunnel: [w1598] -> w1581
          tunnel: [w1601] -> w1583
          tunnel: w1581 -> [w1601]
          frame #0 {
            n710 = Wait (ms)(milliseconds to wait=u32 70) -> ()  [unwired: 1 out]
          }
          frame #1 {
            n711 = call "FGV milisec (subVI).vi"() -> ("time elased(ms)"=→"time elased(ms)":u32)  [unwired: 11 in]
          }
        }
      }
      frame "MEAS.Turn+5V" {
        n712 = disable-structure shown="LOGGING==TRUE" {
          disable-tunnel: w1604 -> [w1620 _]
          frame condition #0 (active) {
            n713 = Empty String/Path?(string/path=w1620) -> (empty?=w1623:bool)
            n714 = Select(t="Quece timeout", s=w1623, f=w1620) -> (s? t:f=w1619:string)
            n715 = call "string log (SubVI).vi"("Enum"=enum16{"Init", "Log", "Read"}."Log", "state Name"=w1619) -> ()  [unwired: 8 in, 2 out]
          }
          frame condition #1 {
          }
        }
        n716 = Variant To Data(type=TRUE, Variant=w1613) -> (data=w1603:bool)  [unwired: 1 in, 1 out]
        n717 = case shown="False" w1603 {
          tunnel: [w1617 w1618] -> w1610
          frame False {
            n718 = call "SC enable OFF.vi"() -> ("error out"=w1617:errorcluster)  [unwired: 11 in]
          }
          frame True {
            n719 = call "SC enable ON.vi"() -> ("error out"=w1618:errorcluster)  [unwired: 11 in]
          }
        }
        n720 = Merge Errors(w1605, w1610) -> (w1606:errorcluster)
        n721 = flat-sequence {
          tunnel: w1606 -> [w1624]
          tunnel: [w1624] -> w1609
          frame #0 {
            n722 = Wait (ms)(milliseconds to wait=u32 2000) -> ()  [unwired: 1 out]
          }
        }
      }
      frame "MEAS.demux1-10" {
        n723 = disable-structure shown="LOGGING==TRUE" {
          disable-tunnel: w1629 -> [w1653 _]
          frame condition #0 (active) {
            n724 = Empty String/Path?(string/path=w1653) -> (empty?=w1656:bool)
            n725 = Select(t="Quece timeout", s=w1656, f=w1653) -> (s? t:f=w1652:string)
            n726 = call "string log (SubVI).vi"("Enum"=enum16{"Init", "Log", "Read"}."Log", "state Name"=w1652) -> ()  [unwired: 8 in, 2 out]
          }
          frame condition #1 {
          }
        }
        n727 = Variant To Data(type=T5."demux1_10_channel0" ("demux1_10(x6)_encode"), Variant=w1637) -> (data=w1628:T5)  [unwired: 1 in, 1 out]
        n728 = case shown="\"demux1_10_channel1\"" w1628 {
          tunnel: [w1641 w1642 w1643 w1644 w1645 w1646 w1647 w1648 w1649 w1650 w1651] -> w1627
          frame "demux1_10_channel0", Default {
            n729 = call "demux1-10_chan0.vi"() -> ("error out"=w1641:errorcluster)  [unwired: 11 in]
          }
          frame "demux1_10_channel1" {
            n730 = call "demux1-10_chan1.vi"() -> ("error out"=w1642:errorcluster)  [unwired: 11 in]
          }
          frame "demux1_10_channel2" {
            n731 = call "demux1-10_chan2.vi"() -> ("error out"=w1643:errorcluster)  [unwired: 11 in]
          }
          frame "demux1_10_channel3" {
            n732 = call "demux1-10_chan3.vi"() -> ("error out"=w1644:errorcluster)  [unwired: 11 in]
          }
          frame "demux1_10_channel4" {
            n733 = call "demux1-10_chan4.vi"() -> ("error out"=w1645:errorcluster)  [unwired: 11 in]
          }
          frame "demux1_10_channel5" {
            n734 = call "demux1-10_chan5.vi"() -> ("error out"=w1646:errorcluster)  [unwired: 11 in]
          }
          frame "demux1_10_channel6" {
            n735 = call "demux1-10_chan6.vi"() -> ("error out"=w1647:errorcluster)  [unwired: 11 in]
          }
          frame "demux1_10_channel7" {
            n736 = call "demux1-10_chan7.vi"() -> ("error out"=w1648:errorcluster)  [unwired: 11 in]
          }
          frame "demux1_10_channel8" {
            n737 = call "demux1-10_chan8.vi"() -> ("error out"=w1649:errorcluster)  [unwired: 11 in]
          }
          frame "demux1_10_channel9" {
            n738 = call "demux1-10_chan9.vi"() -> ("error out"=w1650:errorcluster)  [unwired: 11 in]
          }
          frame "demux1_10_channel10" {
            n739 = call "demux1-10_chan10.vi"() -> ("error out"=w1651:errorcluster)  [unwired: 11 in]
          }
        }
        n740 = Merge Errors(w1630, w1627) -> (w1631:errorcluster)
        n741 = flat-sequence {
          tunnel: [w1657] -> w1632
          tunnel: w1631 -> [w1657]
          frame #0 {
            n742 = Wait (ms)(milliseconds to wait=u32 70) -> ()  [unwired: 1 out]
          }
        }
      }
      frame "MEAS.eMIC" {
        # "wait for DRV stable(10ms),\n then  tester requests to read AC"
        # "eliminated shorted Circuits"
        n743 = disable-structure shown="LOGGING==TRUE" {
          disable-tunnel: w1660 -> [w1685 _]
          frame condition #0 (active) {
            n744 = Empty String/Path?(string/path=w1685) -> (empty?=w1688:bool)
            n745 = Select(t="Quece timeout", s=w1688, f=w1685) -> (s? t:f=w1684:string)
            n746 = call "string log (SubVI).vi"("Enum"=enum16{"Init", "Log", "Read"}."Log", "state Name"=w1684) -> ()  [unwired: 8 in, 2 out]
          }
          frame condition #1 {
          }
        }
        n747 = call "FGV Driver Data.vi"("DUT channel (1-11)"=w1662, "FGV enum"=FGV_DRV_data."Read" ("FGV DRV data enum")) -> ("Short Circuits?"=w1675:bool[])  [unwired: 6 in, 3 out]
        n748 = Variant To Data(type=bool[] [], Variant=w1680) -> (data=w1673:bool[])  [unwired: 1 in, 1 out]
        n749 = Not(x=w1675) -> (.not. x?=w1674:bool[])
        n750 = And(x=w1674, y=w1673) -> (x .and. y?=w1672:bool[])
        n751 = call "MB01_eMICs.vi"("Array"=w1672) -> ("error out"=w1670:errorcluster)  [unwired: 10 in]
        n752 = call "FGV wait for 6 eMICs.vi"("Enum"=enum16{"Init", "count"}."Init", "error in (no error)"=w1670) -> ("error out"=w1666:errorcluster, "wait done"=w1671:bool)  [unwired: 7 in, 1 out]
        n753 = flat-sequence {
          tunnel: w1666 -> [w1691]
          tunnel: [w1691] -> w1667
          tunnel: w1668 -> [w1697]
          tunnel: w1667 -> [w1695]
          tunnel: [w1694] -> w1665
          frame #0 {
            n754 = Wait (ms)(milliseconds to wait=u32 20) -> ()  [unwired: 1 out]
          }
          frame #1 {
            n755 = call "App enquece.vi"("Priority Enquece"=TRUE, "error in (no error)"=w1695, "command"="MEAS.request AC", "queue in"=w1697) -> ("error out"=w1694:errorcluster)  [unwired: 6 in, 1 out]
          }
        }
        n756 = local write "AC Measure  Completed"(w1671) -> ()
        n757 = Merge Errors(w1661, w1665) -> (w1663:errorcluster)
        n758 = flat-sequence {
          tunnel: [w1690] -> w1664
          tunnel: w1663 -> [w1690]
          frame #0 {
            n759 = Wait (ms)(milliseconds to wait=u32 70) -> ()  [unwired: 1 out]
          }
        }
      }
      frame "MEAS.request AC" {
        n760 = disable-structure shown="LOGGING==TRUE" {
          disable-tunnel: w1701 -> [w1714 _]
          frame condition #0 (active) {
            n761 = Empty String/Path?(string/path=w1714) -> (empty?=w1717:bool)
            n762 = Select(t="Quece timeout", s=w1717, f=w1714) -> (s? t:f=w1713:string)
            n763 = call "string log (SubVI).vi"("Enum"=enum16{"Init", "Log", "Read"}."Log", "state Name"=w1713) -> ()  [unwired: 8 in, 2 out]
          }
          frame condition #1 {
          }
        }
        n764 = call "FGV wait for 6 eMICs.vi"("Enum"=enum16{"Init", "count"}."Init") -> ("error out"=w1699:errorcluster)  [unwired: 8 in, 2 out]
        n765 = call "Read AC parameters.vi"("error in"=w1699, "Module ID"=-1) -> ("error out"=w1704:errorcluster)  [unwired: 9 in]
        n766 = Merge Errors(w1705, w1704) -> (w1702:errorcluster)
        n767 = flat-sequence {
          tunnel: [w1718] -> w1703
          tunnel: w1702 -> [w1718]
          frame #0 {
            n768 = Wait (ms)(milliseconds to wait=u32 70) -> ()  [unwired: 1 out]
          }
        }
      }
      frame "MEAS.mux6_1" {
        n769 = disable-structure shown="LOGGING==TRUE" {
          disable-tunnel: w1723 -> [w1749 _]
          frame condition #0 (active) {
            n770 = Empty String/Path?(string/path=w1749) -> (empty?=w1752:bool)
            n771 = Select(t="Quece timeout", s=w1752, f=w1749) -> (s? t:f=w1748:string)
            n772 = call "string log (SubVI).vi"("Enum"=enum16{"Init", "Log", "Read"}."Log", "state Name"=w1748) -> ()  [unwired: 8 in, 2 out]
          }
          frame condition #1 {
          }
        }
        n773 = Variant To Data(type=T3."mux6-1_channel0" ("mux6_1(3wires)_encode"), Variant=w1731) -> (data=w1722:T3)  [unwired: 1 in, 1 out]
        n774 = case shown="\"mux6-1_channel0\", Default" w1722 {
          tunnel: [w1735 w1736 w1737 w1738 w1739 w1740 w1741 w1742 w1743 w1744 w1745 w1746 w1747] -> w1721
          frame "mux6-1_channel0", Default {
            n775 = call "mux6-1_chan0.vi"() -> ("error out"=w1735:errorcluster)  [unwired: 11 in]
          }
          frame "mux6-1_channel1_2" {
            n776 = call "mux6-1_chan1_1.vi"() -> ("error out"=w1736:errorcluster)  [unwired: 11 in]
          }
          frame "mux6_1_channel1_3" {
            n777 = call "mux6-1_chan1_2.vi"() -> ("error out"=w1737:errorcluster)  [unwired: 11 in]
          }
          frame "mux6_1_channel2_2" {
            n778 = call "mux6-1_chan2_1.vi"() -> ("error out"=w1738:errorcluster)  [unwired: 11 in]
          }
          frame "mux6_1_channel2_3" {
            n779 = call "mux6-1_chan2_2.vi"() -> ("error out"=w1739:errorcluster)  [unwired: 11 in]
          }
          frame "mux6_1_channel3_2" {
            n780 = call "mux6-1_chan3_1.vi"() -> ("error out"=w1740:errorcluster)  [unwired: 11 in]
          }
          frame "mux6_1_channel3_3" {
            n781 = call "mux6-1_chan3_2.vi"() -> ("error out"=w1741:errorcluster)  [unwired: 11 in]
          }
          frame "mux6_1_channel4_2" {
            n782 = call "mux6-1_chan4_1.vi"() -> ("error out"=w1742:errorcluster)  [unwired: 11 in]
          }
          frame "mux6_1_channel4_3" {
            n783 = call "mux6-1_chan4_2.vi"() -> ("error out"=w1743:errorcluster)  [unwired: 11 in]
          }
          frame "mux6_1_channel5_2" {
            n784 = call "mux6-1_chan5_1.vi"() -> ("error out"=w1744:errorcluster)  [unwired: 11 in]
          }
          frame "mux6_1_channel5_3" {
            n785 = call "mux6-1_chan5_2.vi"() -> ("error out"=w1745:errorcluster)  [unwired: 11 in]
          }
          frame "mux6_1_channel6_2" {
            n786 = call "mux6-1_chan6_1.vi"() -> ("error out"=w1746:errorcluster)  [unwired: 11 in]
          }
          frame "mux6_1_channel6_3" {
            n787 = call "mux6-1_chan6_2.vi"() -> ("error out"=w1747:errorcluster)  [unwired: 11 in]
          }
        }
        n788 = Merge Errors(w1726, w1721) -> (w1724:errorcluster)
        n789 = flat-sequence {
          tunnel: [w1754] -> w1725
          tunnel: w1724 -> [w1754]
          frame #0 {
            n790 = Wait (ms)(milliseconds to wait=u32 70) -> ()  [unwired: 1 out]
          }
        }
      }
      frame "MEAS.mux10-1" {
        n791 = disable-structure shown="LOGGING==TRUE" {
          disable-tunnel: w1758 -> [w1782 _]
          frame condition #0 (active) {
            n792 = Empty String/Path?(string/path=w1782) -> (empty?=w1785:bool)
            n793 = Select(t="Quece timeout", s=w1785, f=w1782) -> (s? t:f=w1781:string)
            n794 = call "string log (SubVI).vi"("Enum"=enum16{"Init", "Log", "Read"}."Log", "state Name"=w1781) -> ()  [unwired: 8 in, 2 out]
          }
          frame condition #1 {
          }
        }
        n795 = Variant To Data(type=T4."mux10_1_channel0" ("mux10_1(x6)_encode"), Variant=w1766) -> (data=w1757:T4)  [unwired: 1 in, 1 out]
        n796 = case shown="\"mux10_1_channel1\"" w1757 {
          tunnel: [w1770 w1771 w1772 w1773 w1774 w1775 w1776 w1777 w1778 w1779 w1780] -> w1756
          frame "mux10_1_channel0", Default {
            n797 = call "mux10-1_chan0.vi"() -> ("error out"=w1770:errorcluster)  [unwired: 11 in]
          }
          frame "mux10_1_channel1" {
            n798 = call "mux10-1_chan1.vi"() -> ("error out"=w1771:errorcluster)  [unwired: 11 in]
          }
          frame "mux10_1_channel2" {
            n799 = call "mux10-1_chan2.vi"() -> ("error out"=w1772:errorcluster)  [unwired: 11 in]
          }
          frame "mux10_1_channel3" {
            n800 = call "mux10-1_chan3.vi"() -> ("error out"=w1773:errorcluster)  [unwired: 11 in]
          }
          frame "mux10_1_channel4" {
            n801 = call "mux10-1_chan4.vi"() -> ("error out"=w1774:errorcluster)  [unwired: 11 in]
          }
          frame "mux10_1_channel5" {
            n802 = call "mux10-1_chan5.vi"() -> ("error out"=w1775:errorcluster)  [unwired: 11 in]
          }
          frame "mux10_1_channel6" {
            n803 = call "mux10-1_chan6.vi"() -> ("error out"=w1776:errorcluster)  [unwired: 11 in]
          }
          frame "mux10_1_channel7" {
            n804 = call "mux10-1_chan7.vi"() -> ("error out"=w1777:errorcluster)  [unwired: 11 in]
          }
          frame "mux10_1_channel8" {
            n805 = call "mux10-1_chan8.vi"() -> ("error out"=w1778:errorcluster)  [unwired: 11 in]
          }
          frame "mux10_1_channel9" {
            n806 = call "mux10-1_chan9.vi"() -> ("error out"=w1779:errorcluster)  [unwired: 11 in]
          }
          frame "mux10_1_channel10" {
            n807 = call "mux10-1_chan10.vi"() -> ("error out"=w1780:errorcluster)  [unwired: 11 in]
          }
        }
        n808 = Merge Errors(w1761, w1756) -> (w1760:errorcluster)
        n809 = flat-sequence {
          tunnel: w1760 -> [w1786]
          tunnel: [w1786] -> w1759
          frame #0 {
            n810 = Wait (ms)(milliseconds to wait=u32 70) -> ()  [unwired: 1 out]
          }
        }
      }
      frame "MEAS.DMM dual read" {
        n811 = disable-structure shown="LOGGING==TRUE" {
          disable-tunnel: w1793 -> [w1814 _]
          frame condition #0 (active) {
            n812 = Empty String/Path?(string/path=w1814) -> (empty?=w1817:bool)
            n813 = Select(t="Quece timeout", s=w1817, f=w1814) -> (s? t:f=w1813:string)
            n814 = call "string log (SubVI).vi"("Enum"=enum16{"Init", "Log", "Read"}."Log", "state Name"=w1813) -> ()  [unwired: 8 in, 2 out]
          }
          frame condition #1 {
          }
        }
        n815 = flat-sequence {
          tunnel: w1795 -> [w1803]
          tunnel: [w1802] -> w1789
          frame #0 {
            w1810 = u16 2 items=["1st Display", "2nd Display", "1st & 2nd Display"] ("Sets to Display")
            n816 = call "Read DCV_DCI.vi"("Sets to Display"=w1810) -> ("error out"=w1801:errorcluster, "DCI"=w1809:dbl, "DCV"=w1808:dbl)  [unwired: 7 in, 1 out]
            "DCI(mA)" <- w1809
            "DCV(Volts)" <- w1808
            n817 = Build Array(w1808, w1809) -> (w1807:dbl[])
            n818 = To Variant(anything=w1807) -> (Variant=w1806:variant)
            n819 = call "FGV Driver Data.vi"("Mode"=DUT_data_Mode."DC parameter", "DUT index(0-59)"=w1803, "error in (no error)"=w1801, "FGV enum"=FGV_DRV_data."Write" ("FGV DRV data enum"), "data"=w1806) -> ("error out"=w1802:errorcluster)  [unwired: 3 in, 3 out]
          }
        }
        n820 = Merge Errors(w1794, w1789) -> (w1791:errorcluster)
        n821 = flat-sequence {
          tunnel: [w1812] -> w1792
          tunnel: w1791 -> [w1812]
          frame #0 {
            n822 = Wait (ms)(milliseconds to wait=u32 70) -> ()  [unwired: 1 out]
          }
        }
      }
      frame "Test Shorted Circuits" {
        w1835 = T23 {"command"="", "Data"=variant} ("Variant")
        # "Reset UI to gray"
        n823 = disable-structure shown="LOGGING==TRUE" {
          disable-tunnel: w1827 -> [w1848 _]
          frame condition #0 (active) {
            n824 = Empty String/Path?(string/path=w1848) -> (empty?=w1851:bool)
            n825 = Select(t="Quece timeout", s=w1851, f=w1848) -> (s? t:f=w1847:string)
            n826 = call "string log (SubVI).vi"("Enum"=enum16{"Init", "Log", "Read"}."Log", "state Name"=w1847) -> ()  [unwired: 8 in, 2 out]
          }
          frame condition #1 {
          }
        }
        n827 = To Variant(anything=TRUE) -> (Variant=w1838:variant)
        n828 = To Variant(anything=FALSE) -> (Variant=w1822:variant)
        n829 = Bundle By Name(cluster=w1835, "command"="MEAS.AllRelaysOFF") -> (w1840:T23)
        n830 = Bundle By Name(cluster=w1835, "command"="MEAS.Turn+5V", "Data"=w1838) -> (w1839:T23)
        n831 = Bundle By Name(cluster=w1835, "command"="MEAS.Read Optos") -> (w1836:T23)
        n832 = Bundle By Name(cluster=w1835, "command"="MEAS.Turn+5V", "Data"=w1822) -> (w1826:T23)
        n833 = Build Array(w1840, w1839, w1836, w1826) -> (w1828:T23[])
        n834 = Reverse 1D Array(array=w1828) -> (reversed array=w1829:T23[])
        n835 = for {
          tunnel: w1829 -> [w1855] mode=indexing
          tunnel: w1833 -> [w1857]
          tunnel: [w1856] -> w1819 mode=indexing
          n836 = Unbundle By Name(w1855) -> ("command"=w1854:string, "Data"=w1853:variant)
          n837 = call "App enquece.vi"("Priority Enquece"=TRUE, "command data"=w1853, "command"=w1854, "queue in"=w1857) -> ("error out"=w1856:errorcluster)  [unwired: 6 in, 1 out]
        }
        n838 = call "reset DRV UI (SubVI).vi"("Ref  in"=w1832) -> ("error out"=w1820:errorcluster)  [unwired: 9 in, 1 out]
        n839 = Merge Errors(w1821, w1819, w1820) -> (w1825:errorcluster)
      }
      frame "Test Channel 1" {
        w1886 = 1  # DUT channel (1-11)
        w1887 = T10 {"command"="", "command data"=variant} ("element")
        n840 = disable-structure shown="LOGGING==TRUE" {
          disable-tunnel: w1882 -> [w1917 _]
          frame condition #0 (active) {
            n841 = Empty String/Path?(string/path=w1917) -> (empty?=w1920:bool)
            n842 = Select(t="Quece timeout", s=w1920, f=w1917) -> (s? t:f=w1916:string)
            n843 = call "string log (SubVI).vi"("Enum"=enum16{"Init", "Log", "Read"}."Log", "state Name"=w1916) -> ()  [unwired: 8 in, 2 out]
          }
          frame condition #1 {
          }
        }
        n844 = Build Array("Apps.UI Update", "MEAS.AllRelaysOFF", "Apps.WaitForEvent") -> (w1864:string[])
        n845 = for {
          tunnel: [w1907] -> w1866 mode=indexing
          shift-right: [w1906] -> w1865
          shift-left: w1867 -> [w1909]
          tunnel: w1864 -> [w1905] mode=indexing
          n846 = call "App enquece.vi"("Priority Enquece"=TRUE, "command"=w1905, "queue in"=w1909) -> ("error out"=w1907:errorcluster, "Queue out"=w1906:refnum<queue>)  [unwired: 7 in]
        }
        n847 = Build Array("Test DRV 1", "Test DRV 2", "Test DRV 3", "Test DRV 4", "Test DRV 5", "Test DRV 6") -> (w1879:string[])
        n848 = Merge Errors(w1866) -> (w1861:errorcluster)
        n849 = Reverse 1D Array(array=w1879) -> (reversed array=w1880:string[])
        n850 = for {
          tunnel: w1880 -> [w1914] mode=indexing
          tunnel: [w1913] -> w1871 mode=indexing
          shift-right: [w1912] -> w1872
          shift-left: w1865 -> [w1915]
          tunnel: w1861 -> [w1911]
          n851 = call "App enquece.vi"("Priority Enquece"=TRUE, "error in (no error)"=w1911, "command"=w1914, "queue in"=w1915) -> ("error out"=w1913:errorcluster, "Queue out"=w1912:refnum<queue>)  [unwired: 6 in]
        }
        n852 = Initialize Array(TRUE, 6 ("dimension size")) -> (w1890:bool[])
        n853 = To Variant(anything=T5."demux1_10_channel1" ("demux1_10(x6)_encode")) -> (Variant=w1896:variant)
        n854 = To Variant(anything=w1890) -> (Variant=w1889:variant)
        n855 = To Variant(anything=T4."mux10_1_channel1" ("mux10_1(x6)_encode")) -> (Variant=w1900:variant)
        n856 = Bundle By Name(cluster=w1887, "command"="MEAS.mux10-1", "command data"=w1900) -> (w1895:T10)
        n857 = Bundle By Name(cluster=w1887, "command"="MEAS.demux1-10", "command data"=w1896) -> (w1894:T10)
        n858 = Bundle By Name(cluster=w1887, "command"="MEAS.eMIC", "command data"=w1889) -> (w1888:T10)
        n859 = Build Array(w1895, w1894, w1888) -> (w1869:T10[])
        n860 = Merge Errors(w1871) -> (w1870:errorcluster)
        n861 = Reverse 1D Array(array=w1869) -> (reversed array=w1868:T10[])
        n862 = for {
          tunnel: w1868 -> [w1926] mode=indexing
          tunnel: [w1923] -> w1881 mode=indexing
          tunnel: w1870 -> [w1922]
          tunnel: w1872 -> [w1927]
          n863 = Unbundle By Name(w1926) -> ("command"=w1925:string, "command data"=w1924:variant)
          n864 = call "App enquece.vi"("Priority Enquece"=TRUE, "error in (no error)"=w1922, "command data"=w1924, "command"=w1925, "queue in"=w1927) -> ("error out"=w1923:errorcluster)  [unwired: 5 in, 1 out]
        }
        n865 = Merge Errors(w1884, w1881) -> (w1885:errorcluster)
      }
      frame "Test Channel 2" {
        w1958 = 2  # DUT channel (1-11)
        w1959 = T10 {"command"="", "command data"=variant} ("element")
        n866 = disable-structure shown="LOGGING==TRUE" {
          disable-tunnel: w1953 -> [w1987 _]
          frame condition #0 (active) {
            n867 = Empty String/Path?(string/path=w1987) -> (empty?=w1990:bool)
            n868 = Select(t="Quece timeout", s=w1990, f=w1987) -> (s? t:f=w1986:string)
            n869 = call "string log (SubVI).vi"("Enum"=enum16{"Init", "Log", "Read"}."Log", "state Name"=w1986) -> ()  [unwired: 8 in, 2 out]
          }
          frame condition #1 {
          }
        }
        n870 = Build Array("Apps.UI Update", "MEAS.AllRelaysOFF", "Apps.WaitForEvent") -> (w1930:string[])
        n871 = for {
          tunnel: [w1978] -> w1941 mode=indexing
          shift-right: [w1979] -> w1943
          shift-left: w1936 -> [w1977]
          tunnel: w1930 -> [w1975] mode=indexing
          n872 = call "App enquece.vi"("Priority Enquece"=TRUE, "command"=w1975, "queue in"=w1977) -> ("error out"=w1978:errorcluster, "Queue out"=w1979:refnum<queue>)  [unwired: 7 in]
        }
        n873 = Merge Errors(w1941) -> (w1933:errorcluster)
        n874 = Build Array("Test DRV 7", "Test DRV 8", "Test DRV 9", "Test DRV 10", "Test DRV 11", "Test DRV 12") -> (w1950:string[])
        n875 = Reverse 1D Array(array=w1950) -> (reversed array=w1951:string[])
        n876 = for {
          tunnel: w1951 -> [w1980] mode=indexing
          tunnel: [w1984] -> w1940 mode=indexing
          shift-right: [w1983] -> w1942
          shift-left: w1943 -> [w1985]
          tunnel: w1933 -> [w1982]
          n877 = call "App enquece.vi"("Priority Enquece"=TRUE, "error in (no error)"=w1982, "command"=w1980, "queue in"=w1985) -> ("error out"=w1984:errorcluster, "Queue out"=w1983:refnum<queue>)  [unwired: 6 in]
        }
        n878 = Initialize Array(TRUE, 6 ("dimension size")) -> (w1962:bool[])
        n879 = To Variant(anything=T4."mux10_1_channel2" ("mux10_1(x6)_encode")) -> (Variant=w1970:variant)
        n880 = To Variant(anything=T5."demux1_10_channel2" ("demux1_10(x6)_encode")) -> (Variant=w1967:variant)
        n881 = To Variant(anything=w1962) -> (Variant=w1961:variant)
        n882 = Bundle By Name(cluster=w1959, "command"="MEAS.mux10-1", "command data"=w1970) -> (w1966:T10)
        n883 = Bundle By Name(cluster=w1959, "command"="MEAS.demux1-10", "command data"=w1967) -> (w1965:T10)
        n884 = Bundle By Name(cluster=w1959, "command"="MEAS.eMIC", "command data"=w1961) -> (w1960:T10)
        n885 = Merge Errors(w1940) -> (w1939:errorcluster)
        n886 = Build Array(w1966, w1965, w1960) -> (w1938:T10[])
        n887 = Reverse 1D Array(array=w1938) -> (reversed array=w1937:T10[])
        n888 = for {
          tunnel: w1937 -> [w1996] mode=indexing
          tunnel: [w1993] -> w1952 mode=indexing
          tunnel: w1939 -> [w1992]
          tunnel: w1942 -> [w1997]
          n889 = Unbundle By Name(w1996) -> ("command"=w1995:string, "command data"=w1994:variant)
          n890 = call "App enquece.vi"("Priority Enquece"=TRUE, "error in (no error)"=w1992, "command data"=w1994, "command"=w1995, "queue in"=w1997) -> ("error out"=w1993:errorcluster)  [unwired: 5 in, 1 out]
        }
        n891 = Merge Errors(w1955, w1952) -> (w1956:errorcluster)
      }
      frame "Test Channel 3" {
        w2027 = 3  # DUT channel (1-11)
        w2028 = T10 {"command"="", "command data"=variant} ("element")
        n892 = disable-structure shown="LOGGING==TRUE" {
          disable-tunnel: w2022 -> [w2057 _]
          frame condition #0 (active) {
            n893 = Empty String/Path?(string/path=w2057) -> (empty?=w2060:bool)
            n894 = Select(t="Quece timeout", s=w2060, f=w2057) -> (s? t:f=w2056:string)
            n895 = call "string log (SubVI).vi"("Enum"=enum16{"Init", "Log", "Read"}."Log", "state Name"=w2056) -> ()  [unwired: 8 in, 2 out]
          }
          frame condition #1 {
          }
        }
        n896 = Build Array("Apps.UI Update", "MEAS.AllRelaysOFF", "Apps.WaitForEvent") -> (w2002:string[])
        n897 = for {
          tunnel: [w2047] -> w2010 mode=indexing
          shift-right: [w2048] -> w2012
          shift-left: w2005 -> [w2046]
          tunnel: w2002 -> [w2045] mode=indexing
          n898 = call "App enquece.vi"("Priority Enquece"=TRUE, "command"=w2045, "queue in"=w2046) -> ("error out"=w2047:errorcluster, "Queue out"=w2048:refnum<queue>)  [unwired: 7 in]
        }
        n899 = Merge Errors(w2010) -> (w2001:errorcluster)
        n900 = Build Array("Test DRV 13", "Test DRV 14", "Test DRV 15", "Test DRV 16", "Test DRV 17", "Test DRV 18") -> (w2019:string[])
        n901 = Reverse 1D Array(array=w2019) -> (reversed array=w2020:string[])
        n902 = for {
          tunnel: w2020 -> [w2054] mode=indexing
          tunnel: [w2053] -> w2009 mode=indexing
          shift-right: [w2052] -> w2011
          shift-left: w2012 -> [w2055]
          tunnel: w2001 -> [w2051]
          n903 = call "App enquece.vi"("Priority Enquece"=TRUE, "error in (no error)"=w2051, "command"=w2054, "queue in"=w2055) -> ("error out"=w2053:errorcluster, "Queue out"=w2052:refnum<queue>)  [unwired: 6 in]
        }
        n904 = Initialize Array(TRUE, 6 ("dimension size")) -> (w2031:bool[])
        n905 = To Variant(anything=w2031) -> (Variant=w2030:variant)
        n906 = To Variant(anything=T5."demux1_10_channel3" ("demux1_10(x6)_encode")) -> (Variant=w2036:variant)
        n907 = To Variant(anything=T4."mux10_1_channel3" ("mux10_1(x6)_encode")) -> (Variant=w2040:variant)
        n908 = Bundle By Name(cluster=w2028, "command"="MEAS.mux10-1", "command data"=w2040) -> (w2035:T10)
        n909 = Bundle By Name(cluster=w2028, "command"="MEAS.demux1-10", "command data"=w2036) -> (w2034:T10)
        n910 = Bundle By Name(cluster=w2028, "command"="MEAS.eMIC", "command data"=w2030) -> (w2029:T10)
        n911 = Build Array(w2035, w2034, w2029) -> (w2007:T10[])
        n912 = Reverse 1D Array(array=w2007) -> (reversed array=w2006:T10[])
        n913 = Merge Errors(w2009) -> (w2008:errorcluster)
        n914 = for {
          tunnel: w2006 -> [w2066] mode=indexing
          tunnel: [w2063] -> w2021 mode=indexing
          tunnel: w2008 -> [w2062]
          tunnel: w2011 -> [w2067]
          n915 = Unbundle By Name(w2066) -> ("command"=w2065:string, "command data"=w2064:variant)
          n916 = call "App enquece.vi"("Priority Enquece"=TRUE, "error in (no error)"=w2062, "command data"=w2064, "command"=w2065, "queue in"=w2067) -> ("error out"=w2063:errorcluster)  [unwired: 5 in, 1 out]
        }
        n917 = Merge Errors(w2024, w2021) -> (w2025:errorcluster)
      }
      frame "Test Channel 4" {
        w2097 = 4  # DUT channel (1-11)
        w2098 = T10 {"command"="", "command data"=variant} ("element")
        n918 = disable-structure shown="LOGGING==TRUE" {
          disable-tunnel: w2092 -> [w2127 _]
          frame condition #0 (active) {
            n919 = Empty String/Path?(string/path=w2127) -> (empty?=w2130:bool)
            n920 = Select(t="Quece timeout", s=w2130, f=w2127) -> (s? t:f=w2126:string)
            n921 = call "string log (SubVI).vi"("Enum"=enum16{"Init", "Log", "Read"}."Log", "state Name"=w2126) -> ()  [unwired: 8 in, 2 out]
          }
          frame condition #1 {
          }
        }
        n922 = Build Array("Apps.UI Update", "MEAS.AllRelaysOFF", "Apps.WaitForEvent") -> (w2072:string[])
        n923 = for {
          tunnel: [w2117] -> w2080 mode=indexing
          shift-right: [w2118] -> w2082
          shift-left: w2075 -> [w2116]
          tunnel: w2072 -> [w2115] mode=indexing
          n924 = call "App enquece.vi"("Priority Enquece"=TRUE, "command"=w2115, "queue in"=w2116) -> ("error out"=w2117:errorcluster, "Queue out"=w2118:refnum<queue>)  [unwired: 7 in]
        }
        n925 = Merge Errors(w2080) -> (w2071:errorcluster)
        n926 = Build Array("Test DRV 19", "Test DRV 20", "Test DRV 21", "Test DRV 22", "Test DRV 23", "Test DRV 24") -> (w2089:string[])
        n927 = Reverse 1D Array(array=w2089) -> (reversed array=w2090:string[])
        n928 = for {
          tunnel: w2090 -> [w2124] mode=indexing
          tunnel: [w2123] -> w2079 mode=indexing
          shift-right: [w2122] -> w2081
          shift-left: w2082 -> [w2125]
          tunnel: w2071 -> [w2121]
          n929 = call "App enquece.vi"("Priority Enquece"=TRUE, "error in (no error)"=w2121, "command"=w2124, "queue in"=w2125) -> ("error out"=w2123:errorcluster, "Queue out"=w2122:refnum<queue>)  [unwired: 6 in]
        }
        n930 = Initialize Array(TRUE, 6 ("dimension size")) -> (w2101:bool[])
        n931 = To Variant(anything=T4."mux10_1_channel4" ("mux10_1(x6)_encode")) -> (Variant=w2110:variant)
        n932 = To Variant(anything=T5."demux1_10_channel4" ("demux1_10(x6)_encode")) -> (Variant=w2106:variant)
        n933 = To Variant(anything=w2101) -> (Variant=w2100:variant)
        n934 = Bundle By Name(cluster=w2098, "command"="MEAS.mux10-1", "command data"=w2110) -> (w2105:T10)
        n935 = Bundle By Name(cluster=w2098, "command"="MEAS.demux1-10", "command data"=w2106) -> (w2104:T10)
        n936 = Bundle By Name(cluster=w2098, "command"="MEAS.eMIC", "command data"=w2100) -> (w2099:T10)
        n937 = Merge Errors(w2079) -> (w2078:errorcluster)
        n938 = Build Array(w2105, w2104, w2099) -> (w2077:T10[])
        n939 = Reverse 1D Array(array=w2077) -> (reversed array=w2076:T10[])
        n940 = for {
          tunnel: w2076 -> [w2136] mode=indexing
          tunnel: [w2133] -> w2091 mode=indexing
          tunnel: w2078 -> [w2132]
          tunnel: w2081 -> [w2137]
          n941 = Unbundle By Name(w2136) -> ("command"=w2135:string, "command data"=w2134:variant)
          n942 = call "App enquece.vi"("Priority Enquece"=TRUE, "error in (no error)"=w2132, "command data"=w2134, "command"=w2135, "queue in"=w2137) -> ("error out"=w2133:errorcluster)  [unwired: 5 in, 1 out]
        }
        n943 = Merge Errors(w2094, w2091) -> (w2095:errorcluster)
      }
      frame "Test Channel 5" {
        w2167 = 5  # DUT channel (1-11)
        w2168 = T10 {"command"="", "command data"=variant} ("element")
        n944 = disable-structure shown="LOGGING==TRUE" {
          disable-tunnel: w2162 -> [w2197 _]
          frame condition #0 (active) {
            n945 = Empty String/Path?(string/path=w2197) -> (empty?=w2200:bool)
            n946 = Select(t="Quece timeout", s=w2200, f=w2197) -> (s? t:f=w2196:string)
            n947 = call "string log (SubVI).vi"("Enum"=enum16{"Init", "Log", "Read"}."Log", "state Name"=w2196) -> ()  [unwired: 8 in, 2 out]
          }
          frame condition #1 {
          }
        }
        n948 = Build Array("Apps.UI Update", "MEAS.AllRelaysOFF", "Apps.WaitForEvent") -> (w2143:string[])
        n949 = for {
          tunnel: [w2187] -> w2151 mode=indexing
          shift-right: [w2188] -> w2152
          shift-left: w2146 -> [w2186]
          tunnel: w2143 -> [w2185] mode=indexing
          n950 = call "App enquece.vi"("Priority Enquece"=TRUE, "command"=w2185, "queue in"=w2186) -> ("error out"=w2187:errorcluster, "Queue out"=w2188:refnum<queue>)  [unwired: 7 in]
        }
        n951 = Merge Errors(w2151) -> (w2142:errorcluster)
        n952 = Build Array("Test DRV 25", "Test DRV 26", "Test DRV 27", "Test DRV 28", "Test DRV 29", "Test DRV 30") -> (w2159:string[])
        n953 = Reverse 1D Array(array=w2159) -> (reversed array=w2160:string[])
        n954 = for {
          tunnel: w2160 -> [w2194] mode=indexing
          tunnel: [w2193] -> w2150 mode=indexing
          shift-right: [w2192] -> w2141
          shift-left: w2152 -> [w2195]
          tunnel: w2142 -> [w2191]
          n955 = call "App enquece.vi"("Priority Enquece"=TRUE, "error in (no error)"=w2191, "command"=w2194, "queue in"=w2195) -> ("error out"=w2193:errorcluster, "Queue out"=w2192:refnum<queue>)  [unwired: 6 in]
        }
        n956 = Initialize Array(TRUE, 6 ("dimension size")) -> (w2171:bool[])
        n957 = To Variant(anything=T4."mux10_1_channel5" ("mux10_1(x6)_encode")) -> (Variant=w2180:variant)
        n958 = To Variant(anything=T5."demux1_10_channel5" ("demux1_10(x6)_encode")) -> (Variant=w2176:variant)
        n959 = To Variant(anything=w2171) -> (Variant=w2170:variant)
        n960 = Bundle By Name(cluster=w2168, "command"="MEAS.mux10-1", "command data"=w2180) -> (w2175:T10)
        n961 = Bundle By Name(cluster=w2168, "command"="MEAS.demux1-10", "command data"=w2176) -> (w2174:T10)
        n962 = Bundle By Name(cluster=w2168, "command"="MEAS.eMIC", "command data"=w2170) -> (w2169:T10)
        n963 = Build Array(w2175, w2174, w2169) -> (w2148:T10[])
        n964 = Merge Errors(w2150) -> (w2149:errorcluster)
        n965 = Reverse 1D Array(array=w2148) -> (reversed array=w2147:T10[])
        n966 = for {
          tunnel: w2147 -> [w2207] mode=indexing
          tunnel: [w2204] -> w2161 mode=indexing
          tunnel: w2149 -> [w2203]
          tunnel: w2141 -> [w2201]
          n967 = Unbundle By Name(w2207) -> ("command"=w2206:string, "command data"=w2205:variant)
          n968 = call "App enquece.vi"("Priority Enquece"=TRUE, "error in (no error)"=w2203, "command data"=w2205, "command"=w2206, "queue in"=w2201) -> ("error out"=w2204:errorcluster)  [unwired: 5 in, 1 out]
        }
        n969 = Merge Errors(w2164, w2161) -> (w2165:errorcluster)
      }
      frame "Test Channel 6" {
        w2237 = 6  # DUT channel (1-11)
        w2238 = T10 {"command"="", "command data"=variant} ("element")
        n970 = disable-structure shown="LOGGING==TRUE" {
          disable-tunnel: w2232 -> [w2267 _]
          frame condition #0 (active) {
            n971 = Empty String/Path?(string/path=w2267) -> (empty?=w2270:bool)
            n972 = Select(t="Quece timeout", s=w2270, f=w2267) -> (s? t:f=w2266:string)
            n973 = call "string log (SubVI).vi"("Enum"=enum16{"Init", "Log", "Read"}."Log", "state Name"=w2266) -> ()  [unwired: 8 in, 2 out]
          }
          frame condition #1 {
          }
        }
        n974 = Build Array("Apps.UI Update", "MEAS.AllRelaysOFF", "Apps.WaitForEvent") -> (w2212:string[])
        n975 = for {
          tunnel: [w2257] -> w2220 mode=indexing
          shift-right: [w2258] -> w2222
          shift-left: w2215 -> [w2256]
          tunnel: w2212 -> [w2255] mode=indexing
          n976 = call "App enquece.vi"("Priority Enquece"=TRUE, "command"=w2255, "queue in"=w2256) -> ("error out"=w2257:errorcluster, "Queue out"=w2258:refnum<queue>)  [unwired: 7 in]
        }
        n977 = Merge Errors(w2220) -> (w2211:errorcluster)
        n978 = Build Array("Test DRV 31", "Test DRV 32", "Test DRV 33", "Test DRV 34", "Test DRV 35", "Test DRV 36") -> (w2229:string[])
        n979 = Reverse 1D Array(array=w2229) -> (reversed array=w2230:string[])
        n980 = for {
          tunnel: w2230 -> [w2264] mode=indexing
          tunnel: [w2263] -> w2219 mode=indexing
          shift-right: [w2262] -> w2221
          shift-left: w2222 -> [w2265]
          tunnel: w2211 -> [w2261]
          n981 = call "App enquece.vi"("Priority Enquece"=TRUE, "error in (no error)"=w2261, "command"=w2264, "queue in"=w2265) -> ("error out"=w2263:errorcluster, "Queue out"=w2262:refnum<queue>)  [unwired: 6 in]
        }
        n982 = Initialize Array(TRUE, 6 ("dimension size")) -> (w2241:bool[])
        n983 = To Variant(anything=T4."mux10_1_channel6" ("mux10_1(x6)_encode")) -> (Variant=w2250:variant)
        n984 = To Variant(anything=T5."demux1_10_channel6" ("demux1_10(x6)_encode")) -> (Variant=w2246:variant)
        n985 = To Variant(anything=w2241) -> (Variant=w2240:variant)
        n986 = Merge Errors(w2219) -> (w2218:errorcluster)
        n987 = Bundle By Name(cluster=w2238, "command"="MEAS.mux10-1", "command data"=w2250) -> (w2245:T10)
        n988 = Bundle By Name(cluster=w2238, "command"="MEAS.demux1-10", "command data"=w2246) -> (w2244:T10)
        n989 = Bundle By Name(cluster=w2238, "command"="MEAS.eMIC", "command data"=w2240) -> (w2239:T10)
        n990 = Build Array(w2245, w2244, w2239) -> (w2217:T10[])
        n991 = Reverse 1D Array(array=w2217) -> (reversed array=w2216:T10[])
        n992 = for {
          tunnel: w2216 -> [w2276] mode=indexing
          tunnel: [w2273] -> w2231 mode=indexing
          tunnel: w2218 -> [w2272]
          tunnel: w2221 -> [w2277]
          n993 = Unbundle By Name(w2276) -> ("command"=w2275:string, "command data"=w2274:variant)
          n994 = call "App enquece.vi"("Priority Enquece"=TRUE, "error in (no error)"=w2272, "command data"=w2274, "command"=w2275, "queue in"=w2277) -> ("error out"=w2273:errorcluster)  [unwired: 5 in, 1 out]
        }
        n995 = Merge Errors(w2234, w2231) -> (w2235:errorcluster)
      }
      frame "Test Channel 7" {
        w2307 = 7  # DUT channel (1-11)
        w2308 = T10 {"command"="", "command data"=variant} ("element")
        n996 = disable-structure shown="LOGGING==TRUE" {
          disable-tunnel: w2302 -> [w2337 _]
          frame condition #0 (active) {
            n997 = Empty String/Path?(string/path=w2337) -> (empty?=w2340:bool)
            n998 = Select(t="Quece timeout", s=w2340, f=w2337) -> (s? t:f=w2336:string)
            n999 = call "string log (SubVI).vi"("Enum"=enum16{"Init", "Log", "Read"}."Log", "state Name"=w2336) -> ()  [unwired: 8 in, 2 out]
          }
          frame condition #1 {
          }
        }
        n1000 = Build Array("Apps.UI Update", "MEAS.AllRelaysOFF", "Apps.WaitForEvent") -> (w2285:string[])
        n1001 = for {
          tunnel: [w2327] -> w2292 mode=indexing
          shift-right: [w2328] -> w2293
          shift-left: w2288 -> [w2326]
          tunnel: w2285 -> [w2325] mode=indexing
          n1002 = call "App enquece.vi"("Priority Enquece"=TRUE, "command"=w2325, "queue in"=w2326) -> ("error out"=w2327:errorcluster, "Queue out"=w2328:refnum<queue>)  [unwired: 7 in]
        }
        n1003 = Build Array("Test DRV 37", "Test DRV 38", "Test DRV 39", "Test DRV 40", "Test DRV 41", "Test DRV 42") -> (w2299:string[])
        n1004 = Merge Errors(w2292) -> (w2284:errorcluster)
        n1005 = Reverse 1D Array(array=w2299) -> (reversed array=w2300:string[])
        n1006 = for {
          tunnel: w2300 -> [w2334] mode=indexing
          tunnel: [w2333] -> w2291 mode=indexing
          shift-right: [w2332] -> w2283
          shift-left: w2293 -> [w2335]
          tunnel: w2284 -> [w2331]
          n1007 = call "App enquece.vi"("Priority Enquece"=TRUE, "error in (no error)"=w2331, "command"=w2334, "queue in"=w2335) -> ("error out"=w2333:errorcluster, "Queue out"=w2332:refnum<queue>)  [unwired: 6 in]
        }
        n1008 = Initialize Array(TRUE, 6 ("dimension size")) -> (w2311:bool[])
        n1009 = Merge Errors(w2291) -> (w2290:errorcluster)
        n1010 = To Variant(anything=w2311) -> (Variant=w2310:variant)
        n1011 = To Variant(anything=T4."mux10_1_channel7" ("mux10_1(x6)_encode")) -> (Variant=w2320:variant)
        n1012 = To Variant(anything=T5."demux1_10_channel7" ("demux1_10(x6)_encode")) -> (Variant=w2316:variant)
        n1013 = Bundle By Name(cluster=w2308, "command"="MEAS.mux10-1", "command data"=w2320) -> (w2315:T10)
        n1014 = Bundle By Name(cluster=w2308, "command"="MEAS.demux1-10", "command data"=w2316) -> (w2314:T10)
        n1015 = Bundle By Name(cluster=w2308, "command"="MEAS.eMIC", "command data"=w2310) -> (w2309:T10)
        n1016 = Build Array(w2315, w2314, w2309) -> (w2289:T10[])
        n1017 = Reverse 1D Array(array=w2289) -> (reversed array=w2282:T10[])
        n1018 = for {
          tunnel: w2282 -> [w2347] mode=indexing
          tunnel: [w2344] -> w2301 mode=indexing
          tunnel: w2290 -> [w2343]
          tunnel: w2283 -> [w2341]
          n1019 = Unbundle By Name(w2347) -> ("command"=w2346:string, "command data"=w2345:variant)
          n1020 = call "App enquece.vi"("Priority Enquece"=TRUE, "error in (no error)"=w2343, "command data"=w2345, "command"=w2346, "queue in"=w2341) -> ("error out"=w2344:errorcluster)  [unwired: 5 in, 1 out]
        }
        n1021 = Merge Errors(w2304, w2301) -> (w2305:errorcluster)
      }
      frame "Test Channel 8" {
        w2377 = 8  # DUT channel (1-11)
        w2378 = T10 {"command"="", "command data"=variant} ("element")
        n1022 = disable-structure shown="LOGGING==TRUE" {
          disable-tunnel: w2372 -> [w2407 _]
          frame condition #0 (active) {
            n1023 = Empty String/Path?(string/path=w2407) -> (empty?=w2410:bool)
            n1024 = Select(t="Quece timeout", s=w2410, f=w2407) -> (s? t:f=w2406:string)
            n1025 = call "string log (SubVI).vi"("Enum"=enum16{"Init", "Log", "Read"}."Log", "state Name"=w2406) -> ()  [unwired: 8 in, 2 out]
          }
          frame condition #1 {
          }
        }
        n1026 = Build Array("Apps.UI Update", "MEAS.AllRelaysOFF", "Apps.WaitForEvent") -> (w2353:string[])
        n1027 = for {
          tunnel: [w2397] -> w2361 mode=indexing
          shift-right: [w2398] -> w2363
          shift-left: w2356 -> [w2396]
          tunnel: w2353 -> [w2395] mode=indexing
          n1028 = call "App enquece.vi"("Priority Enquece"=TRUE, "command"=w2395, "queue in"=w2396) -> ("error out"=w2397:errorcluster, "Queue out"=w2398:refnum<queue>)  [unwired: 7 in]
        }
        n1029 = Merge Errors(w2361) -> (w2352:errorcluster)
        n1030 = Build Array("Test DRV 43", "Test DRV 44", "Test DRV 45", "Test DRV 46", "Test DRV 47", "Test DRV 48") -> (w2369:string[])
        n1031 = Reverse 1D Array(array=w2369) -> (reversed array=w2370:string[])
        n1032 = for {
          tunnel: w2370 -> [w2404] mode=indexing
          tunnel: [w2403] -> w2360 mode=indexing
          shift-right: [w2402] -> w2362
          shift-left: w2363 -> [w2405]
          tunnel: w2352 -> [w2401]
          n1033 = call "App enquece.vi"("Priority Enquece"=TRUE, "error in (no error)"=w2401, "command"=w2404, "queue in"=w2405) -> ("error out"=w2403:errorcluster, "Queue out"=w2402:refnum<queue>)  [unwired: 6 in]
        }
        n1034 = Initialize Array(TRUE, 6 ("dimension size")) -> (w2381:bool[])
        n1035 = To Variant(anything=T4."mux10_1_channel8" ("mux10_1(x6)_encode")) -> (Variant=w2390:variant)
        n1036 = To Variant(anything=T5."demux1_10_channel8" ("demux1_10(x6)_encode")) -> (Variant=w2386:variant)
        n1037 = To Variant(anything=w2381) -> (Variant=w2380:variant)
        n1038 = Bundle By Name(cluster=w2378, "command"="MEAS.mux10-1", "command data"=w2390) -> (w2385:T10)
        n1039 = Bundle By Name(cluster=w2378, "command"="MEAS.demux1-10", "command data"=w2386) -> (w2384:T10)
        n1040 = Bundle By Name(cluster=w2378, "command"="MEAS.eMIC", "command data"=w2380) -> (w2379:T10)
        n1041 = Build Array(w2385, w2384, w2379) -> (w2358:T10[])
        n1042 = Merge Errors(w2360) -> (w2359:errorcluster)
        n1043 = Reverse 1D Array(array=w2358) -> (reversed array=w2357:T10[])
        n1044 = for {
          tunnel: w2357 -> [w2416] mode=indexing
          tunnel: [w2413] -> w2371 mode=indexing
          tunnel: w2359 -> [w2412]
          tunnel: w2362 -> [w2417]
          n1045 = Unbundle By Name(w2416) -> ("command"=w2415:string, "command data"=w2414:variant)
          n1046 = call "App enquece.vi"("Priority Enquece"=TRUE, "error in (no error)"=w2412, "command data"=w2414, "command"=w2415, "queue in"=w2417) -> ("error out"=w2413:errorcluster)  [unwired: 5 in, 1 out]
        }
        n1047 = Merge Errors(w2374, w2371) -> (w2375:errorcluster)
      }
      frame "Test Channel 9" {
        w2448 = 9  # DUT channel (1-10)
        w2449 = T10 {"command"="", "command data"=variant} ("element")
        n1048 = disable-structure shown="LOGGING==TRUE" {
          disable-tunnel: w2443 -> [w2477 _]
          frame condition #0 (active) {
            n1049 = Empty String/Path?(string/path=w2477) -> (empty?=w2480:bool)
            n1050 = Select(t="Quece timeout", s=w2480, f=w2477) -> (s? t:f=w2476:string)
            n1051 = call "string log (SubVI).vi"("Enum"=enum16{"Init", "Log", "Read"}."Log", "state Name"=w2476) -> ()  [unwired: 8 in, 2 out]
          }
          frame condition #1 {
          }
        }
        n1052 = Build Array("Apps.UI Update", "MEAS.AllRelaysOFF", "Apps.WaitForEvent") -> (w2422:string[])
        n1053 = for {
          tunnel: [w2467] -> w2431 mode=indexing
          shift-right: [w2468] -> w2433
          shift-left: w2426 -> [w2466]
          tunnel: w2422 -> [w2465] mode=indexing
          n1054 = call "App enquece.vi"("Priority Enquece"=TRUE, "command"=w2465, "queue in"=w2466) -> ("error out"=w2467:errorcluster, "Queue out"=w2468:refnum<queue>)  [unwired: 7 in]
        }
        n1055 = Merge Errors(w2431) -> (w2421:errorcluster)
        n1056 = Build Array("Test DRV 49", "Test DRV 50", "Test DRV 51", "Test DRV 52", "Test DRV 53", "Test DRV 54") -> (w2440:string[])
        n1057 = Reverse 1D Array(array=w2440) -> (reversed array=w2441:string[])
        n1058 = for {
          tunnel: w2441 -> [w2474] mode=indexing
          tunnel: [w2473] -> w2430 mode=indexing
          shift-right: [w2472] -> w2432
          shift-left: w2433 -> [w2475]
          tunnel: w2421 -> [w2471]
          n1059 = call "App enquece.vi"("Priority Enquece"=TRUE, "error in (no error)"=w2471, "command"=w2474, "queue in"=w2475) -> ("error out"=w2473:errorcluster, "Queue out"=w2472:refnum<queue>)  [unwired: 6 in]
        }
        n1060 = Initialize Array(TRUE, 6 ("dimension size")) -> (w2452:bool[])
        n1061 = To Variant(anything=T4."mux10_1_channel9" ("mux10_1(x6)_encode")) -> (Variant=w2461:variant)
        n1062 = To Variant(anything=T5."demux1_10_channel9" ("demux1_10(x6)_encode")) -> (Variant=w2457:variant)
        n1063 = To Variant(anything=w2452) -> (Variant=w2451:variant)
        n1064 = Bundle By Name(cluster=w2449, "command"="MEAS.mux10-1", "command data"=w2461) -> (w2456:T10)
        n1065 = Bundle By Name(cluster=w2449, "command"="MEAS.demux1-10", "command data"=w2457) -> (w2455:T10)
        n1066 = Bundle By Name(cluster=w2449, "command"="MEAS.eMIC", "command data"=w2451) -> (w2450:T10)
        n1067 = Build Array(w2456, w2455, w2450) -> (w2428:T10[])
        n1068 = Merge Errors(w2430) -> (w2429:errorcluster)
        n1069 = Reverse 1D Array(array=w2428) -> (reversed array=w2427:T10[])
        n1070 = for {
          tunnel: w2427 -> [w2487] mode=indexing
          tunnel: [w2484] -> w2442 mode=indexing
          shift-right: [w2483] -> _
          shift-left: w2432 -> [w2488]
          tunnel: w2429 -> [w2482]
          n1071 = Unbundle By Name(w2487) -> ("command"=w2486:string, "command data"=w2485:variant)
          n1072 = call "App enquece.vi"("Priority Enquece"=TRUE, "error in (no error)"=w2482, "command data"=w2485, "command"=w2486, "queue in"=w2488) -> ("error out"=w2484:errorcluster, "Queue out"=w2483:refnum<queue>)  [unwired: 5 in]
        }
        n1073 = Merge Errors(w2445, w2442) -> (w2446:errorcluster)
      }
      frame "Test Channel 10" {
        w2519 = 10  # DUT channel (1-10)
        w2492 = T10 {"command"="", "command data"=variant} ("element")
        n1074 = disable-structure shown="LOGGING==TRUE" {
          disable-tunnel: w2514 -> [w2548 _]
          frame condition #0 (active) {
            n1075 = Empty String/Path?(string/path=w2548) -> (empty?=w2551:bool)
            n1076 = Select(t="Quece timeout", s=w2551, f=w2548) -> (s? t:f=w2547:string)
            n1077 = call "string log (SubVI).vi"("Enum"=enum16{"Init", "Log", "Read"}."Log", "state Name"=w2547) -> ()  [unwired: 8 in, 2 out]
          }
          frame condition #1 {
          }
        }
        n1078 = Build Array("Apps.UI Update", "MEAS.AllRelaysOFF", "Apps.WaitForEvent") -> (w2494:string[])
        n1079 = for {
          tunnel: [w2538] -> w2502 mode=indexing
          shift-right: [w2539] -> w2504
          shift-left: w2497 -> [w2537]
          tunnel: w2494 -> [w2536] mode=indexing
          n1080 = call "App enquece.vi"("Priority Enquece"=TRUE, "command"=w2536, "queue in"=w2537) -> ("error out"=w2538:errorcluster, "Queue out"=w2539:refnum<queue>)  [unwired: 7 in]
        }
        n1081 = Merge Errors(w2502) -> (w2493:errorcluster)
        n1082 = Build Array("Test DRV 55", "Test DRV 56", "Test DRV 57", "Test DRV 58", "Test DRV 59", "Test DRV 60") -> (w2511:string[])
        n1083 = Reverse 1D Array(array=w2511) -> (reversed array=w2512:string[])
        n1084 = for {
          tunnel: w2512 -> [w2545] mode=indexing
          tunnel: [w2544] -> w2501 mode=indexing
          shift-right: [w2543] -> w2503
          shift-left: w2504 -> [w2546]
          tunnel: w2493 -> [w2542]
          n1085 = call "App enquece.vi"("Priority Enquece"=TRUE, "error in (no error)"=w2542, "command"=w2545, "queue in"=w2546) -> ("error out"=w2544:errorcluster, "Queue out"=w2543:refnum<queue>)  [unwired: 6 in]
        }
        n1086 = Initialize Array(TRUE, 6 ("dimension size")) -> (w2522:bool[])
        n1087 = To Variant(anything=T4."mux10_1_channel10" ("mux10_1(x6)_encode")) -> (Variant=w2531:variant)
        n1088 = To Variant(anything=T5."demux1_10_channel10" ("demux1_10(x6)_encode")) -> (Variant=w2527:variant)
        n1089 = To Variant(anything=w2522) -> (Variant=w2521:variant)
        n1090 = Merge Errors(w2501) -> (w2500:errorcluster)
        n1091 = Bundle By Name(cluster=w2492, "command"="MEAS.mux10-1", "command data"=w2531) -> (w2526:T10)
        n1092 = Bundle By Name(cluster=w2492, "command"="MEAS.demux1-10", "command data"=w2527) -> (w2525:T10)
        n1093 = Bundle By Name(cluster=w2492, "command"="MEAS.eMIC", "command data"=w2521) -> (w2520:T10)
        n1094 = Build Array(w2526, w2525, w2520) -> (w2499:T10[])
        n1095 = Reverse 1D Array(array=w2499) -> (reversed array=w2498:T10[])
        n1096 = for {
          tunnel: w2498 -> [w2557] mode=indexing
          tunnel: [w2554] -> w2513 mode=indexing
          tunnel: w2500 -> [w2553]
          tunnel: w2503 -> [w2558]
          n1097 = Unbundle By Name(w2557) -> ("command"=w2556:string, "command data"=w2555:variant)
          n1098 = call "App enquece.vi"("Priority Enquece"=TRUE, "error in (no error)"=w2553, "command data"=w2555, "command"=w2556, "queue in"=w2558) -> ("error out"=w2554:errorcluster)  [unwired: 5 in, 1 out]
        }
        n1099 = Merge Errors(w2516, w2513) -> (w2517:errorcluster)
      }
      frame "Test DRV 1" {
        w2560 = 0  # DUT index(0-59)
        w2564 = T10 {"command"="", "command data"=variant} ("element")
        w2562 = "MEAS.mux6_1"
        n1100 = disable-structure shown="LOGGING==TRUE" {
          disable-tunnel: w2566 -> [w2587 _]
          frame condition #0 (active) {
            n1101 = Empty String/Path?(string/path=w2587) -> (empty?=w2590:bool)
            n1102 = Select(t="Quece timeout", s=w2590, f=w2587) -> (s? t:f=w2586:string)
            n1103 = call "string log (SubVI).vi"("Enum"=enum16{"Init", "Log", "Read"}."Log", "state Name"=w2586) -> ()  [unwired: 8 in, 2 out]
          }
          frame condition #1 {
          }
        }
        n1104 = To Variant(anything=T3."mux6_1_channel1_3" ("mux6_1(3wires)_encode")) -> (Variant=w2576:variant)
        n1105 = To Variant(anything=T3."mux6-1_channel0" ("mux6_1(3wires)_encode")) -> (Variant=w2561:variant)
        n1106 = To Variant(anything=T3."mux6-1_channel1_2" ("mux6_1(3wires)_encode")) -> (Variant=w2574:variant)
        n1107 = Bundle By Name(cluster=w2564, "command"=w2562, "command data"=w2574) -> (w2573:T10)
        n1108 = Bundle By Name(cluster=w2564, "command"=w2562, "command data"=w2576) -> (w2572:T10)
        n1109 = Bundle By Name(cluster=w2564, "command"=w2562, "command data"=w2561) -> (w2563:T10)
        n1110 = Bundle By Name(cluster=w2564, "command"="MEAS.DMM dual read") -> (w2570:T10)
        n1111 = Build Array(w2573, w2572, w2570, w2563) -> (w2568:T10[])
        n1112 = Reverse 1D Array(array=w2568) -> (reversed array=w2569:T10[])
        n1113 = for {
          tunnel: [w2596] -> w2581 mode=indexing
          tunnel: w2578 -> [w2595]
          tunnel: w2569 -> [w2594] mode=indexing
          n1114 = Unbundle By Name(w2594) -> ("command"=w2593:string, "command data"=w2592:variant)
          n1115 = call "App enquece.vi"("Priority Enquece"=TRUE, "command data"=w2592, "command"=w2593, "queue in"=w2595) -> ("error out"=w2596:errorcluster)  [unwired: 6 in, 1 out]
        }
        n1116 = Merge Errors(w2579, w2581) -> (w2580:errorcluster)
      }
      frame "Test DRV 2" {
        w2604 = 1  # DUT index(0-59)
        w2601 = T10 {"command"="", "command data"=variant} ("element")
        w2599 = "MEAS.mux6_1"
        n1117 = disable-structure shown="LOGGING==TRUE" {
          disable-tunnel: w2603 -> [w2625 _]
          frame condition #0 (active) {
            n1118 = Empty String/Path?(string/path=w2625) -> (empty?=w2628:bool)
            n1119 = Select(t="Quece timeout", s=w2628, f=w2625) -> (s? t:f=w2624:string)
            n1120 = call "string log (SubVI).vi"("Enum"=enum16{"Init", "Log", "Read"}."Log", "state Name"=w2624) -> ()  [unwired: 8 in, 2 out]
          }
          frame condition #1 {
          }
        }
        n1121 = To Variant(anything=T3."mux6-1_channel0" ("mux6_1(3wires)_encode")) -> (Variant=w2598:variant)
        n1122 = To Variant(anything=T3."mux6_1_channel2_3" ("mux6_1(3wires)_encode")) -> (Variant=w2614:variant)
        n1123 = To Variant(anything=T3."mux6_1_channel2_2" ("mux6_1(3wires)_encode")) -> (Variant=w2612:variant)
        n1124 = Bundle By Name(cluster=w2601, "command"=w2599, "command data"=w2612) -> (w2611:T10)
        n1125 = Bundle By Name(cluster=w2601, "command"=w2599, "command data"=w2614) -> (w2610:T10)
        n1126 = Bundle By Name(cluster=w2601, "command"=w2599, "command data"=w2598) -> (w2600:T10)
        n1127 = Bundle By Name(cluster=w2601, "command"="MEAS.DMM dual read") -> (w2608:T10)
        n1128 = Build Array(w2611, w2610, w2608, w2600) -> (w2606:T10[])
        n1129 = Reverse 1D Array(array=w2606) -> (reversed array=w2607:T10[])
        n1130 = for {
          tunnel: [w2634] -> w2619 mode=indexing
          tunnel: w2616 -> [w2633]
          tunnel: w2607 -> [w2632] mode=indexing
          n1131 = Unbundle By Name(w2632) -> ("command"=w2631:string, "command data"=w2630:variant)
          n1132 = call "App enquece.vi"("Priority Enquece"=TRUE, "command data"=w2630, "command"=w2631, "queue in"=w2633) -> ("error out"=w2634:errorcluster)  [unwired: 6 in, 1 out]
        }
        n1133 = Merge Errors(w2617, w2619) -> (w2618:errorcluster)
      }
      frame "Test DRV 3" {
        w2642 = 2  # DUT index(0-59)
        w2639 = T10 {"command"="", "command data"=variant} ("element")
        w2637 = "MEAS.mux6_1"
        n1134 = disable-structure shown="LOGGING==TRUE" {
          disable-tunnel: w2641 -> [w2663 _]
          frame condition #0 (active) {
            n1135 = Empty String/Path?(string/path=w2663) -> (empty?=w2666:bool)
            n1136 = Select(t="Quece timeout", s=w2666, f=w2663) -> (s? t:f=w2662:string)
            n1137 = call "string log (SubVI).vi"("Enum"=enum16{"Init", "Log", "Read"}."Log", "state Name"=w2662) -> ()  [unwired: 8 in, 2 out]
          }
          frame condition #1 {
          }
        }
        n1138 = To Variant(anything=T3."mux6-1_channel0" ("mux6_1(3wires)_encode")) -> (Variant=w2636:variant)
        n1139 = To Variant(anything=T3."mux6_1_channel3_3" ("mux6_1(3wires)_encode")) -> (Variant=w2652:variant)
        n1140 = To Variant(anything=T3."mux6_1_channel3_2" ("mux6_1(3wires)_encode")) -> (Variant=w2650:variant)
        n1141 = Bundle By Name(cluster=w2639, "command"=w2637, "command data"=w2650) -> (w2649:T10)
        n1142 = Bundle By Name(cluster=w2639, "command"=w2637, "command data"=w2652) -> (w2648:T10)
        n1143 = Bundle By Name(cluster=w2639, "command"=w2637, "command data"=w2636) -> (w2638:T10)
        n1144 = Bundle By Name(cluster=w2639, "command"="MEAS.DMM dual read") -> (w2646:T10)
        n1145 = Build Array(w2649, w2648, w2646, w2638) -> (w2644:T10[])
        n1146 = Reverse 1D Array(array=w2644) -> (reversed array=w2645:T10[])
        n1147 = for {
          tunnel: [w2672] -> w2657 mode=indexing
          tunnel: w2654 -> [w2671]
          tunnel: w2645 -> [w2670] mode=indexing
          n1148 = Unbundle By Name(w2670) -> ("command"=w2669:string, "command data"=w2668:variant)
          n1149 = call "App enquece.vi"("Priority Enquece"=TRUE, "command data"=w2668, "command"=w2669, "queue in"=w2671) -> ("error out"=w2672:errorcluster)  [unwired: 6 in, 1 out]
        }
        n1150 = Merge Errors(w2655, w2657) -> (w2656:errorcluster)
      }
      frame "Test DRV 4" {
        w2680 = 3  # DUT index(0-59)
        w2677 = T10 {"command"="", "command data"=variant} ("element")
        w2675 = "MEAS.mux6_1"
        n1151 = disable-structure shown="LOGGING==TRUE" {
          disable-tunnel: w2679 -> [w2701 _]
          frame condition #0 (active) {
            n1152 = Empty String/Path?(string/path=w2701) -> (empty?=w2704:bool)
            n1153 = Select(t="Quece timeout", s=w2704, f=w2701) -> (s? t:f=w2700:string)
            n1154 = call "string log (SubVI).vi"("Enum"=enum16{"Init", "Log", "Read"}."Log", "state Name"=w2700) -> ()  [unwired: 8 in, 2 out]
          }
          frame condition #1 {
          }
        }
        n1155 = To Variant(anything=T3."mux6-1_channel0" ("mux6_1(3wires)_encode")) -> (Variant=w2674:variant)
        n1156 = To Variant(anything=T3."mux6_1_channel4_3" ("mux6_1(3wires)_encode")) -> (Variant=w2690:variant)
        n1157 = To Variant(anything=T3."mux6_1_channel4_2" ("mux6_1(3wires)_encode")) -> (Variant=w2688:variant)
        n1158 = Bundle By Name(cluster=w2677, "command"=w2675, "command data"=w2688) -> (w2687:T10)
        n1159 = Bundle By Name(cluster=w2677, "command"=w2675, "command data"=w2690) -> (w2686:T10)
        n1160 = Bundle By Name(cluster=w2677, "command"=w2675, "command data"=w2674) -> (w2676:T10)
        n1161 = Bundle By Name(cluster=w2677, "command"="MEAS.DMM dual read") -> (w2684:T10)
        n1162 = Build Array(w2687, w2686, w2684, w2676) -> (w2682:T10[])
        n1163 = Reverse 1D Array(array=w2682) -> (reversed array=w2683:T10[])
        n1164 = for {
          tunnel: [w2710] -> w2695 mode=indexing
          tunnel: w2692 -> [w2709]
          tunnel: w2683 -> [w2708] mode=indexing
          n1165 = Unbundle By Name(w2708) -> ("command"=w2707:string, "command data"=w2706:variant)
          n1166 = call "App enquece.vi"("Priority Enquece"=TRUE, "command data"=w2706, "command"=w2707, "queue in"=w2709) -> ("error out"=w2710:errorcluster)  [unwired: 6 in, 1 out]
        }
        n1167 = Merge Errors(w2693, w2695) -> (w2694:errorcluster)
      }
      frame "Test DRV 5" {
        w2718 = 4  # DUT index(0-59)
        w2715 = T10 {"command"="", "command data"=variant} ("element")
        w2713 = "MEAS.mux6_1"
        n1168 = disable-structure shown="LOGGING==TRUE" {
          disable-tunnel: w2717 -> [w2739 _]
          frame condition #0 (active) {
            n1169 = Empty String/Path?(string/path=w2739) -> (empty?=w2742:bool)
            n1170 = Select(t="Quece timeout", s=w2742, f=w2739) -> (s? t:f=w2738:string)
            n1171 = call "string log (SubVI).vi"("Enum"=enum16{"Init", "Log", "Read"}."Log", "state Name"=w2738) -> ()  [unwired: 8 in, 2 out]
          }
          frame condition #1 {
          }
        }
        n1172 = To Variant(anything=T3."mux6-1_channel0" ("mux6_1(3wires)_encode")) -> (Variant=w2712:variant)
        n1173 = To Variant(anything=T3."mux6_1_channel5_3" ("mux6_1(3wires)_encode")) -> (Variant=w2728:variant)
        n1174 = To Variant(anything=T3."mux6_1_channel5_2" ("mux6_1(3wires)_encode")) -> (Variant=w2726:variant)
        n1175 = Bundle By Name(cluster=w2715, "command"=w2713, "command data"=w2726) -> (w2725:T10)
        n1176 = Bundle By Name(cluster=w2715, "command"=w2713, "command data"=w2728) -> (w2724:T10)
        n1177 = Bundle By Name(cluster=w2715, "command"=w2713, "command data"=w2712) -> (w2714:T10)
        n1178 = Bundle By Name(cluster=w2715, "command"="MEAS.DMM dual read") -> (w2722:T10)
        n1179 = Build Array(w2725, w2724, w2722, w2714) -> (w2720:T10[])
        n1180 = Reverse 1D Array(array=w2720) -> (reversed array=w2721:T10[])
        n1181 = for {
          tunnel: [w2748] -> w2733 mode=indexing
          tunnel: w2730 -> [w2747]
          tunnel: w2721 -> [w2746] mode=indexing
          n1182 = Unbundle By Name(w2746) -> ("command"=w2745:string, "command data"=w2744:variant)
          n1183 = call "App enquece.vi"("Priority Enquece"=TRUE, "command data"=w2744, "command"=w2745, "queue in"=w2747) -> ("error out"=w2748:errorcluster)  [unwired: 6 in, 1 out]
        }
        n1184 = Merge Errors(w2731, w2733) -> (w2732:errorcluster)
      }
      frame "Test DRV 6" {
        w2756 = 5  # DUT index(0-59)
        w2753 = T10 {"command"="", "command data"=variant} ("element")
        w2751 = "MEAS.mux6_1"
        n1185 = disable-structure shown="LOGGING==TRUE" {
          disable-tunnel: w2755 -> [w2777 _]
          frame condition #0 (active) {
            n1186 = Empty String/Path?(string/path=w2777) -> (empty?=w2780:bool)
            n1187 = Select(t="Quece timeout", s=w2780, f=w2777) -> (s? t:f=w2776:string)
            n1188 = call "string log (SubVI).vi"("Enum"=enum16{"Init", "Log", "Read"}."Log", "state Name"=w2776) -> ()  [unwired: 8 in, 2 out]
          }
          frame condition #1 {
          }
        }
        n1189 = To Variant(anything=T3."mux6-1_channel0" ("mux6_1(3wires)_encode")) -> (Variant=w2750:variant)
        n1190 = To Variant(anything=T3."mux6_1_channel6_3" ("mux6_1(3wires)_encode")) -> (Variant=w2766:variant)
        n1191 = To Variant(anything=T3."mux6_1_channel6_2" ("mux6_1(3wires)_encode")) -> (Variant=w2764:variant)
        n1192 = Bundle By Name(cluster=w2753, "command"=w2751, "command data"=w2764) -> (w2763:T10)
        n1193 = Bundle By Name(cluster=w2753, "command"=w2751, "command data"=w2766) -> (w2762:T10)
        n1194 = Bundle By Name(cluster=w2753, "command"=w2751, "command data"=w2750) -> (w2752:T10)
        n1195 = Bundle By Name(cluster=w2753, "command"="MEAS.DMM dual read") -> (w2760:T10)
        n1196 = Build Array(w2763, w2762, w2760, w2752) -> (w2758:T10[])
        n1197 = Reverse 1D Array(array=w2758) -> (reversed array=w2759:T10[])
        n1198 = for {
          tunnel: [w2786] -> w2771 mode=indexing
          tunnel: w2768 -> [w2785]
          tunnel: w2759 -> [w2784] mode=indexing
          n1199 = Unbundle By Name(w2784) -> ("command"=w2783:string, "command data"=w2782:variant)
          n1200 = call "App enquece.vi"("Priority Enquece"=TRUE, "command data"=w2782, "command"=w2783, "queue in"=w2785) -> ("error out"=w2786:errorcluster)  [unwired: 6 in, 1 out]
        }
        n1201 = Merge Errors(w2769, w2771) -> (w2770:errorcluster)
      }
      frame "Test DRV 7" {
        w2794 = 6  # DUT index(0-59)
        w2791 = T10 {"command"="", "command data"=variant} ("element")
        w2789 = "MEAS.mux6_1"
        n1202 = disable-structure shown="LOGGING==TRUE" {
          disable-tunnel: w2793 -> [w2815 _]
          frame condition #0 (active) {
            n1203 = Empty String/Path?(string/path=w2815) -> (empty?=w2818:bool)
            n1204 = Select(t="Quece timeout", s=w2818, f=w2815) -> (s? t:f=w2814:string)
            n1205 = call "string log (SubVI).vi"("Enum"=enum16{"Init", "Log", "Read"}."Log", "state Name"=w2814) -> ()  [unwired: 8 in, 2 out]
          }
          frame condition #1 {
          }
        }
        n1206 = To Variant(anything=T3."mux6-1_channel0" ("mux6_1(3wires)_encode")) -> (Variant=w2788:variant)
        n1207 = To Variant(anything=T3."mux6_1_channel1_3" ("mux6_1(3wires)_encode")) -> (Variant=w2804:variant)
        n1208 = To Variant(anything=T3."mux6-1_channel1_2" ("mux6_1(3wires)_encode")) -> (Variant=w2802:variant)
        n1209 = Bundle By Name(cluster=w2791, "command"=w2789, "command data"=w2802) -> (w2801:T10)
        n1210 = Bundle By Name(cluster=w2791, "command"=w2789, "command data"=w2804) -> (w2800:T10)
        n1211 = Bundle By Name(cluster=w2791, "command"=w2789, "command data"=w2788) -> (w2790:T10)
        n1212 = Bundle By Name(cluster=w2791, "command"="MEAS.DMM dual read") -> (w2798:T10)
        n1213 = Build Array(w2801, w2800, w2798, w2790) -> (w2796:T10[])
        n1214 = Reverse 1D Array(array=w2796) -> (reversed array=w2797:T10[])
        n1215 = for {
          tunnel: [w2824] -> w2809 mode=indexing
          tunnel: w2806 -> [w2823]
          tunnel: w2797 -> [w2822] mode=indexing
          n1216 = Unbundle By Name(w2822) -> ("command"=w2821:string, "command data"=w2820:variant)
          n1217 = call "App enquece.vi"("Priority Enquece"=TRUE, "command data"=w2820, "command"=w2821, "queue in"=w2823) -> ("error out"=w2824:errorcluster)  [unwired: 6 in, 1 out]
        }
        n1218 = Merge Errors(w2807, w2809) -> (w2808:errorcluster)
      }
      frame "Test DRV 8" {
        w2832 = 7  # DUT index(0-59)
        w2829 = T10 {"command"="", "command data"=variant} ("element")
        w2827 = "MEAS.mux6_1"
        n1219 = disable-structure shown="LOGGING==TRUE" {
          disable-tunnel: w2831 -> [w2853 _]
          frame condition #0 (active) {
            n1220 = Empty String/Path?(string/path=w2853) -> (empty?=w2856:bool)
            n1221 = Select(t="Quece timeout", s=w2856, f=w2853) -> (s? t:f=w2852:string)
            n1222 = call "string log (SubVI).vi"("Enum"=enum16{"Init", "Log", "Read"}."Log", "state Name"=w2852) -> ()  [unwired: 8 in, 2 out]
          }
          frame condition #1 {
          }
        }
        n1223 = To Variant(anything=T3."mux6-1_channel0" ("mux6_1(3wires)_encode")) -> (Variant=w2826:variant)
        n1224 = To Variant(anything=T3."mux6_1_channel2_3" ("mux6_1(3wires)_encode")) -> (Variant=w2842:variant)
        n1225 = To Variant(anything=T3."mux6_1_channel2_2" ("mux6_1(3wires)_encode")) -> (Variant=w2840:variant)
        n1226 = Bundle By Name(cluster=w2829, "command"=w2827, "command data"=w2840) -> (w2839:T10)
        n1227 = Bundle By Name(cluster=w2829, "command"=w2827, "command data"=w2842) -> (w2838:T10)
        n1228 = Bundle By Name(cluster=w2829, "command"=w2827, "command data"=w2826) -> (w2828:T10)
        n1229 = Bundle By Name(cluster=w2829, "command"="MEAS.DMM dual read") -> (w2836:T10)
        n1230 = Build Array(w2839, w2838, w2836, w2828) -> (w2834:T10[])
        n1231 = Reverse 1D Array(array=w2834) -> (reversed array=w2835:T10[])
        n1232 = for {
          tunnel: [w2862] -> w2847 mode=indexing
          tunnel: w2844 -> [w2861]
          tunnel: w2835 -> [w2860] mode=indexing
          n1233 = Unbundle By Name(w2860) -> ("command"=w2859:string, "command data"=w2858:variant)
          n1234 = call "App enquece.vi"("Priority Enquece"=TRUE, "command data"=w2858, "command"=w2859, "queue in"=w2861) -> ("error out"=w2862:errorcluster)  [unwired: 6 in, 1 out]
        }
        n1235 = Merge Errors(w2845, w2847) -> (w2846:errorcluster)
      }
      frame "Test DRV 9" {
        w2870 = 8  # DUT index(0-59)
        w2867 = T10 {"command"="", "command data"=variant} ("element")
        w2865 = "MEAS.mux6_1"
        n1236 = disable-structure shown="LOGGING==TRUE" {
          disable-tunnel: w2869 -> [w2891 _]
          frame condition #0 (active) {
            n1237 = Empty String/Path?(string/path=w2891) -> (empty?=w2894:bool)
            n1238 = Select(t="Quece timeout", s=w2894, f=w2891) -> (s? t:f=w2890:string)
            n1239 = call "string log (SubVI).vi"("Enum"=enum16{"Init", "Log", "Read"}."Log", "state Name"=w2890) -> ()  [unwired: 8 in, 2 out]
          }
          frame condition #1 {
          }
        }
        n1240 = To Variant(anything=T3."mux6-1_channel0" ("mux6_1(3wires)_encode")) -> (Variant=w2864:variant)
        n1241 = To Variant(anything=T3."mux6_1_channel3_3" ("mux6_1(3wires)_encode")) -> (Variant=w2880:variant)
        n1242 = To Variant(anything=T3."mux6_1_channel3_2" ("mux6_1(3wires)_encode")) -> (Variant=w2878:variant)
        n1243 = Bundle By Name(cluster=w2867, "command"=w2865, "command data"=w2878) -> (w2877:T10)
        n1244 = Bundle By Name(cluster=w2867, "command"=w2865, "command data"=w2880) -> (w2876:T10)
        n1245 = Bundle By Name(cluster=w2867, "command"=w2865, "command data"=w2864) -> (w2866:T10)
        n1246 = Bundle By Name(cluster=w2867, "command"="MEAS.DMM dual read") -> (w2874:T10)
        n1247 = Build Array(w2877, w2876, w2874, w2866) -> (w2872:T10[])
        n1248 = Reverse 1D Array(array=w2872) -> (reversed array=w2873:T10[])
        n1249 = for {
          tunnel: [w2900] -> w2885 mode=indexing
          tunnel: w2882 -> [w2899]
          tunnel: w2873 -> [w2898] mode=indexing
          n1250 = Unbundle By Name(w2898) -> ("command"=w2897:string, "command data"=w2896:variant)
          n1251 = call "App enquece.vi"("Priority Enquece"=TRUE, "command data"=w2896, "command"=w2897, "queue in"=w2899) -> ("error out"=w2900:errorcluster)  [unwired: 6 in, 1 out]
        }
        n1252 = Merge Errors(w2883, w2885) -> (w2884:errorcluster)
      }
      frame "Test DRV 10" {
        w2908 = 9  # DUT index(0-59)
        w2905 = T10 {"command"="", "command data"=variant} ("element")
        w2903 = "MEAS.mux6_1"
        n1253 = disable-structure shown="LOGGING==TRUE" {
          disable-tunnel: w2907 -> [w2929 _]
          frame condition #0 (active) {
            n1254 = Empty String/Path?(string/path=w2929) -> (empty?=w2932:bool)
            n1255 = Select(t="Quece timeout", s=w2932, f=w2929) -> (s? t:f=w2928:string)
            n1256 = call "string log (SubVI).vi"("Enum"=enum16{"Init", "Log", "Read"}."Log", "state Name"=w2928) -> ()  [unwired: 8 in, 2 out]
          }
          frame condition #1 {
          }
        }
        n1257 = To Variant(anything=T3."mux6-1_channel0" ("mux6_1(3wires)_encode")) -> (Variant=w2902:variant)
        n1258 = To Variant(anything=T3."mux6_1_channel4_3" ("mux6_1(3wires)_encode")) -> (Variant=w2918:variant)
        n1259 = To Variant(anything=T3."mux6_1_channel4_2" ("mux6_1(3wires)_encode")) -> (Variant=w2916:variant)
        n1260 = Bundle By Name(cluster=w2905, "command"=w2903, "command data"=w2916) -> (w2915:T10)
        n1261 = Bundle By Name(cluster=w2905, "command"=w2903, "command data"=w2918) -> (w2914:T10)
        n1262 = Bundle By Name(cluster=w2905, "command"=w2903, "command data"=w2902) -> (w2904:T10)
        n1263 = Bundle By Name(cluster=w2905, "command"="MEAS.DMM dual read") -> (w2912:T10)
        n1264 = Build Array(w2915, w2914, w2912, w2904) -> (w2910:T10[])
        n1265 = Reverse 1D Array(array=w2910) -> (reversed array=w2911:T10[])
        n1266 = for {
          tunnel: [w2938] -> w2923 mode=indexing
          tunnel: w2920 -> [w2937]
          tunnel: w2911 -> [w2936] mode=indexing
          n1267 = Unbundle By Name(w2936) -> ("command"=w2935:string, "command data"=w2934:variant)
          n1268 = call "App enquece.vi"("Priority Enquece"=TRUE, "command data"=w2934, "command"=w2935, "queue in"=w2937) -> ("error out"=w2938:errorcluster)  [unwired: 6 in, 1 out]
        }
        n1269 = Merge Errors(w2921, w2923) -> (w2922:errorcluster)
      }
      frame "Test DRV 11" {
        w2946 = 10  # DUT index(0-59)
        w2943 = T10 {"command"="", "command data"=variant} ("element")
        w2941 = "MEAS.mux6_1"
        n1270 = disable-structure shown="LOGGING==TRUE" {
          disable-tunnel: w2945 -> [w2967 _]
          frame condition #0 (active) {
            n1271 = Empty String/Path?(string/path=w2967) -> (empty?=w2970:bool)
            n1272 = Select(t="Quece timeout", s=w2970, f=w2967) -> (s? t:f=w2966:string)
            n1273 = call "string log (SubVI).vi"("Enum"=enum16{"Init", "Log", "Read"}."Log", "state Name"=w2966) -> ()  [unwired: 8 in, 2 out]
          }
          frame condition #1 {
          }
        }
        n1274 = To Variant(anything=T3."mux6-1_channel0" ("mux6_1(3wires)_encode")) -> (Variant=w2940:variant)
        n1275 = To Variant(anything=T3."mux6_1_channel5_3" ("mux6_1(3wires)_encode")) -> (Variant=w2956:variant)
        n1276 = To Variant(anything=T3."mux6_1_channel5_2" ("mux6_1(3wires)_encode")) -> (Variant=w2954:variant)
        n1277 = Bundle By Name(cluster=w2943, "command"=w2941, "command data"=w2954) -> (w2953:T10)
        n1278 = Bundle By Name(cluster=w2943, "command"=w2941, "command data"=w2956) -> (w2952:T10)
        n1279 = Bundle By Name(cluster=w2943, "command"=w2941, "command data"=w2940) -> (w2942:T10)
        n1280 = Bundle By Name(cluster=w2943, "command"="MEAS.DMM dual read") -> (w2950:T10)
        n1281 = Build Array(w2953, w2952, w2950, w2942) -> (w2948:T10[])
        n1282 = Reverse 1D Array(array=w2948) -> (reversed array=w2949:T10[])
        n1283 = for {
          tunnel: [w2976] -> w2961 mode=indexing
          tunnel: w2958 -> [w2975]
          tunnel: w2949 -> [w2974] mode=indexing
          n1284 = Unbundle By Name(w2974) -> ("command"=w2973:string, "command data"=w2972:variant)
          n1285 = call "App enquece.vi"("Priority Enquece"=TRUE, "command data"=w2972, "command"=w2973, "queue in"=w2975) -> ("error out"=w2976:errorcluster)  [unwired: 6 in, 1 out]
        }
        n1286 = Merge Errors(w2959, w2961) -> (w2960:errorcluster)
      }
      frame "Test DRV 12" {
        w2984 = 11  # DUT index(0-59)
        w2981 = T10 {"command"="", "command data"=variant} ("element")
        w2979 = "MEAS.mux6_1"
        n1287 = disable-structure shown="LOGGING==TRUE" {
          disable-tunnel: w2983 -> [w3005 _]
          frame condition #0 (active) {
            n1288 = Empty String/Path?(string/path=w3005) -> (empty?=w3008:bool)
            n1289 = Select(t="Quece timeout", s=w3008, f=w3005) -> (s? t:f=w3004:string)
            n1290 = call "string log (SubVI).vi"("Enum"=enum16{"Init", "Log", "Read"}."Log", "state Name"=w3004) -> ()  [unwired: 8 in, 2 out]
          }
          frame condition #1 {
          }
        }
        n1291 = To Variant(anything=T3."mux6-1_channel0" ("mux6_1(3wires)_encode")) -> (Variant=w2978:variant)
        n1292 = To Variant(anything=T3."mux6_1_channel6_3" ("mux6_1(3wires)_encode")) -> (Variant=w2994:variant)
        n1293 = To Variant(anything=T3."mux6_1_channel6_2" ("mux6_1(3wires)_encode")) -> (Variant=w2992:variant)
        n1294 = Bundle By Name(cluster=w2981, "command"=w2979, "command data"=w2992) -> (w2991:T10)
        n1295 = Bundle By Name(cluster=w2981, "command"=w2979, "command data"=w2994) -> (w2990:T10)
        n1296 = Bundle By Name(cluster=w2981, "command"=w2979, "command data"=w2978) -> (w2980:T10)
        n1297 = Bundle By Name(cluster=w2981, "command"="MEAS.DMM dual read") -> (w2988:T10)
        n1298 = Build Array(w2991, w2990, w2988, w2980) -> (w2986:T10[])
        n1299 = Reverse 1D Array(array=w2986) -> (reversed array=w2987:T10[])
        n1300 = for {
          tunnel: [w3014] -> w2999 mode=indexing
          tunnel: w2996 -> [w3013]
          tunnel: w2987 -> [w3012] mode=indexing
          n1301 = Unbundle By Name(w3012) -> ("command"=w3011:string, "command data"=w3010:variant)
          n1302 = call "App enquece.vi"("Priority Enquece"=TRUE, "command data"=w3010, "command"=w3011, "queue in"=w3013) -> ("error out"=w3014:errorcluster)  [unwired: 6 in, 1 out]
        }
        n1303 = Merge Errors(w2997, w2999) -> (w2998:errorcluster)
      }
      frame "Test DRV 13" {
        w3022 = 12  # DUT index(0-59)
        w3019 = T10 {"command"="", "command data"=variant} ("element")
        w3017 = "MEAS.mux6_1"
        n1304 = disable-structure shown="LOGGING==TRUE" {
          disable-tunnel: w3021 -> [w3043 _]
          frame condition #0 (active) {
            n1305 = Empty String/Path?(string/path=w3043) -> (empty?=w3046:bool)
            n1306 = Select(t="Quece timeout", s=w3046, f=w3043) -> (s? t:f=w3042:string)
            n1307 = call "string log (SubVI).vi"("Enum"=enum16{"Init", "Log", "Read"}."Log", "state Name"=w3042) -> ()  [unwired: 8 in, 2 out]
          }
          frame condition #1 {
          }
        }
        n1308 = To Variant(anything=T3."mux6-1_channel0" ("mux6_1(3wires)_encode")) -> (Variant=w3016:variant)
        n1309 = To Variant(anything=T3."mux6_1_channel1_3" ("mux6_1(3wires)_encode")) -> (Variant=w3032:variant)
        n1310 = To Variant(anything=T3."mux6-1_channel1_2" ("mux6_1(3wires)_encode")) -> (Variant=w3030:variant)
        n1311 = Bundle By Name(cluster=w3019, "command"=w3017, "command data"=w3030) -> (w3029:T10)
        n1312 = Bundle By Name(cluster=w3019, "command"=w3017, "command data"=w3032) -> (w3028:T10)
        n1313 = Bundle By Name(cluster=w3019, "command"=w3017, "command data"=w3016) -> (w3018:T10)
        n1314 = Bundle By Name(cluster=w3019, "command"="MEAS.DMM dual read") -> (w3026:T10)
        n1315 = Build Array(w3029, w3028, w3026, w3018) -> (w3024:T10[])
        n1316 = Reverse 1D Array(array=w3024) -> (reversed array=w3025:T10[])
        n1317 = for {
          tunnel: [w3052] -> w3037 mode=indexing
          tunnel: w3034 -> [w3051]
          tunnel: w3025 -> [w3050] mode=indexing
          n1318 = Unbundle By Name(w3050) -> ("command"=w3049:string, "command data"=w3048:variant)
          n1319 = call "App enquece.vi"("Priority Enquece"=TRUE, "command data"=w3048, "command"=w3049, "queue in"=w3051) -> ("error out"=w3052:errorcluster)  [unwired: 6 in, 1 out]
        }
        n1320 = Merge Errors(w3035, w3037) -> (w3036:errorcluster)
      }
      frame "Test DRV 14" {
        w3060 = 13  # DUT index(0-59)
        w3057 = T10 {"command"="", "command data"=variant} ("element")
        w3055 = "MEAS.mux6_1"
        n1321 = disable-structure shown="LOGGING==TRUE" {
          disable-tunnel: w3059 -> [w3081 _]
          frame condition #0 (active) {
            n1322 = Empty String/Path?(string/path=w3081) -> (empty?=w3084:bool)
            n1323 = Select(t="Quece timeout", s=w3084, f=w3081) -> (s? t:f=w3080:string)
            n1324 = call "string log (SubVI).vi"("Enum"=enum16{"Init", "Log", "Read"}."Log", "state Name"=w3080) -> ()  [unwired: 8 in, 2 out]
          }
          frame condition #1 {
          }
        }
        n1325 = To Variant(anything=T3."mux6_1_channel2_3" ("mux6_1(3wires)_encode")) -> (Variant=w3070:variant)
        n1326 = To Variant(anything=T3."mux6-1_channel0" ("mux6_1(3wires)_encode")) -> (Variant=w3054:variant)
        n1327 = To Variant(anything=T3."mux6_1_channel2_2" ("mux6_1(3wires)_encode")) -> (Variant=w3068:variant)
        n1328 = Bundle By Name(cluster=w3057, "command"=w3055, "command data"=w3068) -> (w3067:T10)
        n1329 = Bundle By Name(cluster=w3057, "command"=w3055, "command data"=w3070) -> (w3066:T10)
        n1330 = Bundle By Name(cluster=w3057, "command"=w3055, "command data"=w3054) -> (w3056:T10)
        n1331 = Bundle By Name(cluster=w3057, "command"="MEAS.DMM dual read") -> (w3064:T10)
        n1332 = Build Array(w3067, w3066, w3064, w3056) -> (w3062:T10[])
        n1333 = Reverse 1D Array(array=w3062) -> (reversed array=w3063:T10[])
        n1334 = for {
          tunnel: [w3090] -> w3075 mode=indexing
          tunnel: w3072 -> [w3089]
          tunnel: w3063 -> [w3088] mode=indexing
          n1335 = Unbundle By Name(w3088) -> ("command"=w3087:string, "command data"=w3086:variant)
          n1336 = call "App enquece.vi"("Priority Enquece"=TRUE, "command data"=w3086, "command"=w3087, "queue in"=w3089) -> ("error out"=w3090:errorcluster)  [unwired: 6 in, 1 out]
        }
        n1337 = Merge Errors(w3073, w3075) -> (w3074:errorcluster)
      }
      frame "Test DRV 15" {
        w3098 = 14  # DUT index(0-59)
        w3095 = T10 {"command"="", "command data"=variant} ("element")
        w3093 = "MEAS.mux6_1"
        n1338 = disable-structure shown="LOGGING==TRUE" {
          disable-tunnel: w3097 -> [w3119 _]
          frame condition #0 (active) {
            n1339 = Empty String/Path?(string/path=w3119) -> (empty?=w3122:bool)
            n1340 = Select(t="Quece timeout", s=w3122, f=w3119) -> (s? t:f=w3118:string)
            n1341 = call "string log (SubVI).vi"("Enum"=enum16{"Init", "Log", "Read"}."Log", "state Name"=w3118) -> ()  [unwired: 8 in, 2 out]
          }
          frame condition #1 {
          }
        }
        n1342 = To Variant(anything=T3."mux6-1_channel0" ("mux6_1(3wires)_encode")) -> (Variant=w3092:variant)
        n1343 = To Variant(anything=T3."mux6_1_channel3_3" ("mux6_1(3wires)_encode")) -> (Variant=w3108:variant)
        n1344 = To Variant(anything=T3."mux6_1_channel3_2" ("mux6_1(3wires)_encode")) -> (Variant=w3106:variant)
        n1345 = Bundle By Name(cluster=w3095, "command"=w3093, "command data"=w3106) -> (w3105:T10)
        n1346 = Bundle By Name(cluster=w3095, "command"=w3093, "command data"=w3108) -> (w3104:T10)
        n1347 = Bundle By Name(cluster=w3095, "command"=w3093, "command data"=w3092) -> (w3094:T10)
        n1348 = Bundle By Name(cluster=w3095, "command"="MEAS.DMM dual read") -> (w3102:T10)
        n1349 = Build Array(w3105, w3104, w3102, w3094) -> (w3100:T10[])
        n1350 = Reverse 1D Array(array=w3100) -> (reversed array=w3101:T10[])
        n1351 = for {
          tunnel: [w3128] -> w3113 mode=indexing
          tunnel: w3110 -> [w3127]
          tunnel: w3101 -> [w3126] mode=indexing
          n1352 = Unbundle By Name(w3126) -> ("command"=w3125:string, "command data"=w3124:variant)
          n1353 = call "App enquece.vi"("Priority Enquece"=TRUE, "command data"=w3124, "command"=w3125, "queue in"=w3127) -> ("error out"=w3128:errorcluster)  [unwired: 6 in, 1 out]
        }
        n1354 = Merge Errors(w3111, w3113) -> (w3112:errorcluster)
      }
      frame "Test DRV 16" {
        w3136 = 15  # DUT index(0-59)
        w3133 = T10 {"command"="", "command data"=variant} ("element")
        w3131 = "MEAS.mux6_1"
        n1355 = disable-structure shown="LOGGING==TRUE" {
          disable-tunnel: w3135 -> [w3157 _]
          frame condition #0 (active) {
            n1356 = Empty String/Path?(string/path=w3157) -> (empty?=w3160:bool)
            n1357 = Select(t="Quece timeout", s=w3160, f=w3157) -> (s? t:f=w3156:string)
            n1358 = call "string log (SubVI).vi"("Enum"=enum16{"Init", "Log", "Read"}."Log", "state Name"=w3156) -> ()  [unwired: 8 in, 2 out]
          }
          frame condition #1 {
          }
        }
        n1359 = To Variant(anything=T3."mux6-1_channel0" ("mux6_1(3wires)_encode")) -> (Variant=w3130:variant)
        n1360 = To Variant(anything=T3."mux6_1_channel4_3" ("mux6_1(3wires)_encode")) -> (Variant=w3146:variant)
        n1361 = To Variant(anything=T3."mux6_1_channel4_2" ("mux6_1(3wires)_encode")) -> (Variant=w3144:variant)
        n1362 = Bundle By Name(cluster=w3133, "command"=w3131, "command data"=w3144) -> (w3143:T10)
        n1363 = Bundle By Name(cluster=w3133, "command"=w3131, "command data"=w3146) -> (w3142:T10)
        n1364 = Bundle By Name(cluster=w3133, "command"=w3131, "command data"=w3130) -> (w3132:T10)
        n1365 = Bundle By Name(cluster=w3133, "command"="MEAS.DMM dual read") -> (w3140:T10)
        n1366 = Build Array(w3143, w3142, w3140, w3132) -> (w3138:T10[])
        n1367 = Reverse 1D Array(array=w3138) -> (reversed array=w3139:T10[])
        n1368 = for {
          tunnel: [w3166] -> w3151 mode=indexing
          tunnel: w3148 -> [w3165]
          tunnel: w3139 -> [w3164] mode=indexing
          n1369 = Unbundle By Name(w3164) -> ("command"=w3163:string, "command data"=w3162:variant)
          n1370 = call "App enquece.vi"("Priority Enquece"=TRUE, "command data"=w3162, "command"=w3163, "queue in"=w3165) -> ("error out"=w3166:errorcluster)  [unwired: 6 in, 1 out]
        }
        n1371 = Merge Errors(w3149, w3151) -> (w3150:errorcluster)
      }
      frame "Test DRV 17" {
        w3174 = 16  # DUT index(0-59)
        w3171 = T10 {"command"="", "command data"=variant} ("element")
        w3169 = "MEAS.mux6_1"
        n1372 = disable-structure shown="LOGGING==TRUE" {
          disable-tunnel: w3173 -> [w3195 _]
          frame condition #0 (active) {
            n1373 = Empty String/Path?(string/path=w3195) -> (empty?=w3198:bool)
            n1374 = Select(t="Quece timeout", s=w3198, f=w3195) -> (s? t:f=w3194:string)
            n1375 = call "string log (SubVI).vi"("Enum"=enum16{"Init", "Log", "Read"}."Log", "state Name"=w3194) -> ()  [unwired: 8 in, 2 out]
          }
          frame condition #1 {
          }
        }
        n1376 = To Variant(anything=T3."mux6-1_channel0" ("mux6_1(3wires)_encode")) -> (Variant=w3168:variant)
        n1377 = To Variant(anything=T3."mux6_1_channel5_3" ("mux6_1(3wires)_encode")) -> (Variant=w3184:variant)
        n1378 = To Variant(anything=T3."mux6_1_channel5_2" ("mux6_1(3wires)_encode")) -> (Variant=w3182:variant)
        n1379 = Bundle By Name(cluster=w3171, "command"=w3169, "command data"=w3182) -> (w3181:T10)
        n1380 = Bundle By Name(cluster=w3171, "command"=w3169, "command data"=w3184) -> (w3180:T10)
        n1381 = Bundle By Name(cluster=w3171, "command"=w3169, "command data"=w3168) -> (w3170:T10)
        n1382 = Bundle By Name(cluster=w3171, "command"="MEAS.DMM dual read") -> (w3178:T10)
        n1383 = Build Array(w3181, w3180, w3178, w3170) -> (w3176:T10[])
        n1384 = Reverse 1D Array(array=w3176) -> (reversed array=w3177:T10[])
        n1385 = for {
          tunnel: [w3204] -> w3189 mode=indexing
          tunnel: w3186 -> [w3203]
          tunnel: w3177 -> [w3202] mode=indexing
          n1386 = Unbundle By Name(w3202) -> ("command"=w3201:string, "command data"=w3200:variant)
          n1387 = call "App enquece.vi"("Priority Enquece"=TRUE, "command data"=w3200, "command"=w3201, "queue in"=w3203) -> ("error out"=w3204:errorcluster)  [unwired: 6 in, 1 out]
        }
        n1388 = Merge Errors(w3187, w3189) -> (w3188:errorcluster)
      }
      frame "Test DRV 18" {
        w3212 = 17  # DUT index(0-59)
        w3209 = T10 {"command"="", "command data"=variant} ("element")
        w3207 = "MEAS.mux6_1"
        n1389 = disable-structure shown="LOGGING==TRUE" {
          disable-tunnel: w3211 -> [w3233 _]
          frame condition #0 (active) {
            n1390 = Empty String/Path?(string/path=w3233) -> (empty?=w3236:bool)
            n1391 = Select(t="Quece timeout", s=w3236, f=w3233) -> (s? t:f=w3232:string)
            n1392 = call "string log (SubVI).vi"("Enum"=enum16{"Init", "Log", "Read"}."Log", "state Name"=w3232) -> ()  [unwired: 8 in, 2 out]
          }
          frame condition #1 {
          }
        }
        n1393 = To Variant(anything=T3."mux6-1_channel0" ("mux6_1(3wires)_encode")) -> (Variant=w3206:variant)
        n1394 = To Variant(anything=T3."mux6_1_channel6_3" ("mux6_1(3wires)_encode")) -> (Variant=w3222:variant)
        n1395 = To Variant(anything=T3."mux6_1_channel6_2" ("mux6_1(3wires)_encode")) -> (Variant=w3220:variant)
        n1396 = Bundle By Name(cluster=w3209, "command"=w3207, "command data"=w3220) -> (w3219:T10)
        n1397 = Bundle By Name(cluster=w3209, "command"=w3207, "command data"=w3222) -> (w3218:T10)
        n1398 = Bundle By Name(cluster=w3209, "command"=w3207, "command data"=w3206) -> (w3208:T10)
        n1399 = Bundle By Name(cluster=w3209, "command"="MEAS.DMM dual read") -> (w3216:T10)
        n1400 = Build Array(w3219, w3218, w3216, w3208) -> (w3214:T10[])
        n1401 = Reverse 1D Array(array=w3214) -> (reversed array=w3215:T10[])
        n1402 = for {
          tunnel: [w3242] -> w3227 mode=indexing
          tunnel: w3224 -> [w3241]
          tunnel: w3215 -> [w3240] mode=indexing
          n1403 = Unbundle By Name(w3240) -> ("command"=w3239:string, "command data"=w3238:variant)
          n1404 = call "App enquece.vi"("Priority Enquece"=TRUE, "command data"=w3238, "command"=w3239, "queue in"=w3241) -> ("error out"=w3242:errorcluster)  [unwired: 6 in, 1 out]
        }
        n1405 = Merge Errors(w3225, w3227) -> (w3226:errorcluster)
      }
      frame "Test DRV 19" {
        w3250 = 18  # DUT index(0-59)
        w3247 = T10 {"command"="", "command data"=variant} ("element")
        w3245 = "MEAS.mux6_1"
        n1406 = disable-structure shown="LOGGING==TRUE" {
          disable-tunnel: w3249 -> [w3271 _]
          frame condition #0 (active) {
            n1407 = Empty String/Path?(string/path=w3271) -> (empty?=w3274:bool)
            n1408 = Select(t="Quece timeout", s=w3274, f=w3271) -> (s? t:f=w3270:string)
            n1409 = call "string log (SubVI).vi"("Enum"=enum16{"Init", "Log", "Read"}."Log", "state Name"=w3270) -> ()  [unwired: 8 in, 2 out]
          }
          frame condition #1 {
          }
        }
        n1410 = To Variant(anything=T3."mux6-1_channel0" ("mux6_1(3wires)_encode")) -> (Variant=w3244:variant)
        n1411 = To Variant(anything=T3."mux6_1_channel1_3" ("mux6_1(3wires)_encode")) -> (Variant=w3260:variant)
        n1412 = To Variant(anything=T3."mux6-1_channel1_2" ("mux6_1(3wires)_encode")) -> (Variant=w3258:variant)
        n1413 = Bundle By Name(cluster=w3247, "command"=w3245, "command data"=w3258) -> (w3257:T10)
        n1414 = Bundle By Name(cluster=w3247, "command"=w3245, "command data"=w3260) -> (w3256:T10)
        n1415 = Bundle By Name(cluster=w3247, "command"=w3245, "command data"=w3244) -> (w3246:T10)
        n1416 = Bundle By Name(cluster=w3247, "command"="MEAS.DMM dual read") -> (w3254:T10)
        n1417 = Build Array(w3257, w3256, w3254, w3246) -> (w3252:T10[])
        n1418 = Reverse 1D Array(array=w3252) -> (reversed array=w3253:T10[])
        n1419 = for {
          tunnel: [w3280] -> w3265 mode=indexing
          tunnel: w3262 -> [w3279]
          tunnel: w3253 -> [w3278] mode=indexing
          n1420 = Unbundle By Name(w3278) -> ("command"=w3277:string, "command data"=w3276:variant)
          n1421 = call "App enquece.vi"("Priority Enquece"=TRUE, "command data"=w3276, "command"=w3277, "queue in"=w3279) -> ("error out"=w3280:errorcluster)  [unwired: 6 in, 1 out]
        }
        n1422 = Merge Errors(w3263, w3265) -> (w3264:errorcluster)
      }
      frame "Test DRV 20" {
        w3288 = 19  # DUT index(0-59)
        w3285 = T10 {"command"="", "command data"=variant} ("element")
        w3283 = "MEAS.mux6_1"
        n1423 = disable-structure shown="LOGGING==TRUE" {
          disable-tunnel: w3287 -> [w3309 _]
          frame condition #0 (active) {
            n1424 = Empty String/Path?(string/path=w3309) -> (empty?=w3312:bool)
            n1425 = Select(t="Quece timeout", s=w3312, f=w3309) -> (s? t:f=w3308:string)
            n1426 = call "string log (SubVI).vi"("Enum"=enum16{"Init", "Log", "Read"}."Log", "state Name"=w3308) -> ()  [unwired: 8 in, 2 out]
          }
          frame condition #1 {
          }
        }
        n1427 = To Variant(anything=T3."mux6-1_channel0" ("mux6_1(3wires)_encode")) -> (Variant=w3282:variant)
        n1428 = To Variant(anything=T3."mux6_1_channel2_3" ("mux6_1(3wires)_encode")) -> (Variant=w3298:variant)
        n1429 = To Variant(anything=T3."mux6_1_channel2_2" ("mux6_1(3wires)_encode")) -> (Variant=w3296:variant)
        n1430 = Bundle By Name(cluster=w3285, "command"=w3283, "command data"=w3296) -> (w3295:T10)
        n1431 = Bundle By Name(cluster=w3285, "command"=w3283, "command data"=w3298) -> (w3294:T10)
        n1432 = Bundle By Name(cluster=w3285, "command"=w3283, "command data"=w3282) -> (w3284:T10)
        n1433 = Bundle By Name(cluster=w3285, "command"="MEAS.DMM dual read") -> (w3292:T10)
        n1434 = Build Array(w3295, w3294, w3292, w3284) -> (w3290:T10[])
        n1435 = Reverse 1D Array(array=w3290) -> (reversed array=w3291:T10[])
        n1436 = for {
          tunnel: [w3318] -> w3303 mode=indexing
          tunnel: w3300 -> [w3317]
          tunnel: w3291 -> [w3316] mode=indexing
          n1437 = Unbundle By Name(w3316) -> ("command"=w3315:string, "command data"=w3314:variant)
          n1438 = call "App enquece.vi"("Priority Enquece"=TRUE, "command data"=w3314, "command"=w3315, "queue in"=w3317) -> ("error out"=w3318:errorcluster)  [unwired: 6 in, 1 out]
        }
        n1439 = Merge Errors(w3301, w3303) -> (w3302:errorcluster)
      }
      frame "Test DRV 21" {
        w3326 = 20  # DUT index(0-59)
        w3323 = T10 {"command"="", "command data"=variant} ("element")
        w3321 = "MEAS.mux6_1"
        n1440 = disable-structure shown="LOGGING==TRUE" {
          disable-tunnel: w3325 -> [w3347 _]
          frame condition #0 (active) {
            n1441 = Empty String/Path?(string/path=w3347) -> (empty?=w3350:bool)
            n1442 = Select(t="Quece timeout", s=w3350, f=w3347) -> (s? t:f=w3346:string)
            n1443 = call "string log (SubVI).vi"("Enum"=enum16{"Init", "Log", "Read"}."Log", "state Name"=w3346) -> ()  [unwired: 8 in, 2 out]
          }
          frame condition #1 {
          }
        }
        n1444 = To Variant(anything=T3."mux6-1_channel0" ("mux6_1(3wires)_encode")) -> (Variant=w3320:variant)
        n1445 = To Variant(anything=T3."mux6_1_channel3_3" ("mux6_1(3wires)_encode")) -> (Variant=w3336:variant)
        n1446 = To Variant(anything=T3."mux6_1_channel3_2" ("mux6_1(3wires)_encode")) -> (Variant=w3334:variant)
        n1447 = Bundle By Name(cluster=w3323, "command"=w3321, "command data"=w3334) -> (w3333:T10)
        n1448 = Bundle By Name(cluster=w3323, "command"=w3321, "command data"=w3336) -> (w3332:T10)
        n1449 = Bundle By Name(cluster=w3323, "command"=w3321, "command data"=w3320) -> (w3322:T10)
        n1450 = Bundle By Name(cluster=w3323, "command"="MEAS.DMM dual read") -> (w3330:T10)
        n1451 = Build Array(w3333, w3332, w3330, w3322) -> (w3328:T10[])
        n1452 = Reverse 1D Array(array=w3328) -> (reversed array=w3329:T10[])
        n1453 = for {
          tunnel: [w3356] -> w3341 mode=indexing
          tunnel: w3338 -> [w3355]
          tunnel: w3329 -> [w3354] mode=indexing
          n1454 = Unbundle By Name(w3354) -> ("command"=w3353:string, "command data"=w3352:variant)
          n1455 = call "App enquece.vi"("Priority Enquece"=TRUE, "command data"=w3352, "command"=w3353, "queue in"=w3355) -> ("error out"=w3356:errorcluster)  [unwired: 6 in, 1 out]
        }
        n1456 = Merge Errors(w3339, w3341) -> (w3340:errorcluster)
      }
      frame "Test DRV 22" {
        w3364 = 21  # DUT index(0-59)
        w3361 = T10 {"command"="", "command data"=variant} ("element")
        w3359 = "MEAS.mux6_1"
        n1457 = disable-structure shown="LOGGING==TRUE" {
          disable-tunnel: w3363 -> [w3385 _]
          frame condition #0 (active) {
            n1458 = Empty String/Path?(string/path=w3385) -> (empty?=w3388:bool)
            n1459 = Select(t="Quece timeout", s=w3388, f=w3385) -> (s? t:f=w3384:string)
            n1460 = call "string log (SubVI).vi"("Enum"=enum16{"Init", "Log", "Read"}."Log", "state Name"=w3384) -> ()  [unwired: 8 in, 2 out]
          }
          frame condition #1 {
          }
        }
        n1461 = To Variant(anything=T3."mux6-1_channel0" ("mux6_1(3wires)_encode")) -> (Variant=w3358:variant)
        n1462 = To Variant(anything=T3."mux6_1_channel4_3" ("mux6_1(3wires)_encode")) -> (Variant=w3374:variant)
        n1463 = To Variant(anything=T3."mux6_1_channel4_2" ("mux6_1(3wires)_encode")) -> (Variant=w3372:variant)
        n1464 = Bundle By Name(cluster=w3361, "command"=w3359, "command data"=w3372) -> (w3371:T10)
        n1465 = Bundle By Name(cluster=w3361, "command"=w3359, "command data"=w3374) -> (w3370:T10)
        n1466 = Bundle By Name(cluster=w3361, "command"=w3359, "command data"=w3358) -> (w3360:T10)
        n1467 = Bundle By Name(cluster=w3361, "command"="MEAS.DMM dual read") -> (w3368:T10)
        n1468 = Build Array(w3371, w3370, w3368, w3360) -> (w3366:T10[])
        n1469 = Reverse 1D Array(array=w3366) -> (reversed array=w3367:T10[])
        n1470 = for {
          tunnel: [w3394] -> w3379 mode=indexing
          tunnel: w3376 -> [w3393]
          tunnel: w3367 -> [w3392] mode=indexing
          n1471 = Unbundle By Name(w3392) -> ("command"=w3391:string, "command data"=w3390:variant)
          n1472 = call "App enquece.vi"("Priority Enquece"=TRUE, "command data"=w3390, "command"=w3391, "queue in"=w3393) -> ("error out"=w3394:errorcluster)  [unwired: 6 in, 1 out]
        }
        n1473 = Merge Errors(w3377, w3379) -> (w3378:errorcluster)
      }
      frame "Test DRV 23" {
        w3402 = 22  # DUT index(0-59)
        w3399 = T10 {"command"="", "command data"=variant} ("element")
        w3397 = "MEAS.mux6_1"
        n1474 = disable-structure shown="LOGGING==TRUE" {
          disable-tunnel: w3401 -> [w3423 _]
          frame condition #0 (active) {
            n1475 = Empty String/Path?(string/path=w3423) -> (empty?=w3426:bool)
            n1476 = Select(t="Quece timeout", s=w3426, f=w3423) -> (s? t:f=w3422:string)
            n1477 = call "string log (SubVI).vi"("Enum"=enum16{"Init", "Log", "Read"}."Log", "state Name"=w3422) -> ()  [unwired: 8 in, 2 out]
          }
          frame condition #1 {
          }
        }
        n1478 = To Variant(anything=T3."mux6-1_channel0" ("mux6_1(3wires)_encode")) -> (Variant=w3396:variant)
        n1479 = To Variant(anything=T3."mux6_1_channel5_3" ("mux6_1(3wires)_encode")) -> (Variant=w3412:variant)
        n1480 = To Variant(anything=T3."mux6_1_channel5_2" ("mux6_1(3wires)_encode")) -> (Variant=w3410:variant)
        n1481 = Bundle By Name(cluster=w3399, "command"=w3397, "command data"=w3410) -> (w3409:T10)
        n1482 = Bundle By Name(cluster=w3399, "command"=w3397, "command data"=w3412) -> (w3408:T10)
        n1483 = Bundle By Name(cluster=w3399, "command"=w3397, "command data"=w3396) -> (w3398:T10)
        n1484 = Bundle By Name(cluster=w3399, "command"="MEAS.DMM dual read") -> (w3406:T10)
        n1485 = Build Array(w3409, w3408, w3406, w3398) -> (w3404:T10[])
        n1486 = Reverse 1D Array(array=w3404) -> (reversed array=w3405:T10[])
        n1487 = for {
          tunnel: [w3432] -> w3417 mode=indexing
          tunnel: w3414 -> [w3431]
          tunnel: w3405 -> [w3430] mode=indexing
          n1488 = Unbundle By Name(w3430) -> ("command"=w3429:string, "command data"=w3428:variant)
          n1489 = call "App enquece.vi"("Priority Enquece"=TRUE, "command data"=w3428, "command"=w3429, "queue in"=w3431) -> ("error out"=w3432:errorcluster)  [unwired: 6 in, 1 out]
        }
        n1490 = Merge Errors(w3415, w3417) -> (w3416:errorcluster)
      }
      frame "Test DRV 24" {
        w3440 = 23  # DUT index(0-59)
        w3437 = T10 {"command"="", "command data"=variant} ("element")
        w3435 = "MEAS.mux6_1"
        n1491 = disable-structure shown="LOGGING==TRUE" {
          disable-tunnel: w3439 -> [w3461 _]
          frame condition #0 (active) {
            n1492 = Empty String/Path?(string/path=w3461) -> (empty?=w3464:bool)
            n1493 = Select(t="Quece timeout", s=w3464, f=w3461) -> (s? t:f=w3460:string)
            n1494 = call "string log (SubVI).vi"("Enum"=enum16{"Init", "Log", "Read"}."Log", "state Name"=w3460) -> ()  [unwired: 8 in, 2 out]
          }
          frame condition #1 {
          }
        }
        n1495 = To Variant(anything=T3."mux6-1_channel0" ("mux6_1(3wires)_encode")) -> (Variant=w3434:variant)
        n1496 = To Variant(anything=T3."mux6_1_channel6_3" ("mux6_1(3wires)_encode")) -> (Variant=w3450:variant)
        n1497 = To Variant(anything=T3."mux6_1_channel6_2" ("mux6_1(3wires)_encode")) -> (Variant=w3448:variant)
        n1498 = Bundle By Name(cluster=w3437, "command"=w3435, "command data"=w3448) -> (w3447:T10)
        n1499 = Bundle By Name(cluster=w3437, "command"=w3435, "command data"=w3450) -> (w3446:T10)
        n1500 = Bundle By Name(cluster=w3437, "command"=w3435, "command data"=w3434) -> (w3436:T10)
        n1501 = Bundle By Name(cluster=w3437, "command"="MEAS.DMM dual read") -> (w3444:T10)
        n1502 = Build Array(w3447, w3446, w3444, w3436) -> (w3442:T10[])
        n1503 = Reverse 1D Array(array=w3442) -> (reversed array=w3443:T10[])
        n1504 = for {
          tunnel: [w3470] -> w3455 mode=indexing
          tunnel: w3452 -> [w3469]
          tunnel: w3443 -> [w3468] mode=indexing
          n1505 = Unbundle By Name(w3468) -> ("command"=w3467:string, "command data"=w3466:variant)
          n1506 = call "App enquece.vi"("Priority Enquece"=TRUE, "command data"=w3466, "command"=w3467, "queue in"=w3469) -> ("error out"=w3470:errorcluster)  [unwired: 6 in, 1 out]
        }
        n1507 = Merge Errors(w3453, w3455) -> (w3454:errorcluster)
      }
      frame "Test DRV 25" {
        w3478 = 24  # DUT index(0-59)
        w3475 = T10 {"command"="", "command data"=variant} ("element")
        w3473 = "MEAS.mux6_1"
        n1508 = disable-structure shown="LOGGING==TRUE" {
          disable-tunnel: w3477 -> [w3499 _]
          frame condition #0 (active) {
            n1509 = Empty String/Path?(string/path=w3499) -> (empty?=w3502:bool)
            n1510 = Select(t="Quece timeout", s=w3502, f=w3499) -> (s? t:f=w3498:string)
            n1511 = call "string log (SubVI).vi"("Enum"=enum16{"Init", "Log", "Read"}."Log", "state Name"=w3498) -> ()  [unwired: 8 in, 2 out]
          }
          frame condition #1 {
          }
        }
        n1512 = To Variant(anything=T3."mux6-1_channel0" ("mux6_1(3wires)_encode")) -> (Variant=w3472:variant)
        n1513 = To Variant(anything=T3."mux6_1_channel1_3" ("mux6_1(3wires)_encode")) -> (Variant=w3488:variant)
        n1514 = To Variant(anything=T3."mux6-1_channel1_2" ("mux6_1(3wires)_encode")) -> (Variant=w3486:variant)
        n1515 = Bundle By Name(cluster=w3475, "command"=w3473, "command data"=w3486) -> (w3485:T10)
        n1516 = Bundle By Name(cluster=w3475, "command"=w3473, "command data"=w3488) -> (w3484:T10)
        n1517 = Bundle By Name(cluster=w3475, "command"=w3473, "command data"=w3472) -> (w3474:T10)
        n1518 = Bundle By Name(cluster=w3475, "command"="MEAS.DMM dual read") -> (w3482:T10)
        n1519 = Build Array(w3485, w3484, w3482, w3474) -> (w3480:T10[])
        n1520 = Reverse 1D Array(array=w3480) -> (reversed array=w3481:T10[])
        n1521 = for {
          tunnel: [w3508] -> w3493 mode=indexing
          tunnel: w3490 -> [w3507]
          tunnel: w3481 -> [w3506] mode=indexing
          n1522 = Unbundle By Name(w3506) -> ("command"=w3505:string, "command data"=w3504:variant)
          n1523 = call "App enquece.vi"("Priority Enquece"=TRUE, "command data"=w3504, "command"=w3505, "queue in"=w3507) -> ("error out"=w3508:errorcluster)  [unwired: 6 in, 1 out]
        }
        n1524 = Merge Errors(w3491, w3493) -> (w3492:errorcluster)
      }
      frame "Test DRV 26" {
        w3516 = 25  # DUT index(0-59)
        w3513 = T10 {"command"="", "command data"=variant} ("element")
        w3511 = "MEAS.mux6_1"
        n1525 = disable-structure shown="LOGGING==TRUE" {
          disable-tunnel: w3515 -> [w3537 _]
          frame condition #0 (active) {
            n1526 = Empty String/Path?(string/path=w3537) -> (empty?=w3540:bool)
            n1527 = Select(t="Quece timeout", s=w3540, f=w3537) -> (s? t:f=w3536:string)
            n1528 = call "string log (SubVI).vi"("Enum"=enum16{"Init", "Log", "Read"}."Log", "state Name"=w3536) -> ()  [unwired: 8 in, 2 out]
          }
          frame condition #1 {
          }
        }
        n1529 = To Variant(anything=T3."mux6-1_channel0" ("mux6_1(3wires)_encode")) -> (Variant=w3510:variant)
        n1530 = To Variant(anything=T3."mux6_1_channel2_3" ("mux6_1(3wires)_encode")) -> (Variant=w3526:variant)
        n1531 = To Variant(anything=T3."mux6_1_channel2_2" ("mux6_1(3wires)_encode")) -> (Variant=w3524:variant)
        n1532 = Bundle By Name(cluster=w3513, "command"=w3511, "command data"=w3524) -> (w3523:T10)
        n1533 = Bundle By Name(cluster=w3513, "command"=w3511, "command data"=w3526) -> (w3522:T10)
        n1534 = Bundle By Name(cluster=w3513, "command"=w3511, "command data"=w3510) -> (w3512:T10)
        n1535 = Bundle By Name(cluster=w3513, "command"="MEAS.DMM dual read") -> (w3520:T10)
        n1536 = Build Array(w3523, w3522, w3520, w3512) -> (w3518:T10[])
        n1537 = Reverse 1D Array(array=w3518) -> (reversed array=w3519:T10[])
        n1538 = for {
          tunnel: [w3546] -> w3531 mode=indexing
          tunnel: w3528 -> [w3545]
          tunnel: w3519 -> [w3544] mode=indexing
          n1539 = Unbundle By Name(w3544) -> ("command"=w3543:string, "command data"=w3542:variant)
          n1540 = call "App enquece.vi"("Priority Enquece"=TRUE, "command data"=w3542, "command"=w3543, "queue in"=w3545) -> ("error out"=w3546:errorcluster)  [unwired: 6 in, 1 out]
        }
        n1541 = Merge Errors(w3529, w3531) -> (w3530:errorcluster)
      }
      frame "Test DRV 27" {
        w3554 = 26  # DUT index(0-59)
        w3551 = T10 {"command"="", "command data"=variant} ("element")
        w3549 = "MEAS.mux6_1"
        n1542 = disable-structure shown="LOGGING==TRUE" {
          disable-tunnel: w3553 -> [w3575 _]
          frame condition #0 (active) {
            n1543 = Empty String/Path?(string/path=w3575) -> (empty?=w3578:bool)
            n1544 = Select(t="Quece timeout", s=w3578, f=w3575) -> (s? t:f=w3574:string)
            n1545 = call "string log (SubVI).vi"("Enum"=enum16{"Init", "Log", "Read"}."Log", "state Name"=w3574) -> ()  [unwired: 8 in, 2 out]
          }
          frame condition #1 {
          }
        }
        n1546 = To Variant(anything=T3."mux6-1_channel0" ("mux6_1(3wires)_encode")) -> (Variant=w3548:variant)
        n1547 = To Variant(anything=T3."mux6_1_channel3_3" ("mux6_1(3wires)_encode")) -> (Variant=w3564:variant)
        n1548 = To Variant(anything=T3."mux6_1_channel3_2" ("mux6_1(3wires)_encode")) -> (Variant=w3562:variant)
        n1549 = Bundle By Name(cluster=w3551, "command"=w3549, "command data"=w3562) -> (w3561:T10)
        n1550 = Bundle By Name(cluster=w3551, "command"=w3549, "command data"=w3564) -> (w3560:T10)
        n1551 = Bundle By Name(cluster=w3551, "command"=w3549, "command data"=w3548) -> (w3550:T10)
        n1552 = Bundle By Name(cluster=w3551, "command"="MEAS.DMM dual read") -> (w3558:T10)
        n1553 = Build Array(w3561, w3560, w3558, w3550) -> (w3556:T10[])
        n1554 = Reverse 1D Array(array=w3556) -> (reversed array=w3557:T10[])
        n1555 = for {
          tunnel: [w3584] -> w3569 mode=indexing
          tunnel: w3566 -> [w3583]
          tunnel: w3557 -> [w3582] mode=indexing
          n1556 = Unbundle By Name(w3582) -> ("command"=w3581:string, "command data"=w3580:variant)
          n1557 = call "App enquece.vi"("Priority Enquece"=TRUE, "command data"=w3580, "command"=w3581, "queue in"=w3583) -> ("error out"=w3584:errorcluster)  [unwired: 6 in, 1 out]
        }
        n1558 = Merge Errors(w3567, w3569) -> (w3568:errorcluster)
      }
      frame "Test DRV 28" {
        w3592 = 27  # DUT index(0-59)
        w3589 = T10 {"command"="", "command data"=variant} ("element")
        w3587 = "MEAS.mux6_1"
        n1559 = disable-structure shown="LOGGING==TRUE" {
          disable-tunnel: w3591 -> [w3613 _]
          frame condition #0 (active) {
            n1560 = Empty String/Path?(string/path=w3613) -> (empty?=w3616:bool)
            n1561 = Select(t="Quece timeout", s=w3616, f=w3613) -> (s? t:f=w3612:string)
            n1562 = call "string log (SubVI).vi"("Enum"=enum16{"Init", "Log", "Read"}."Log", "state Name"=w3612) -> ()  [unwired: 8 in, 2 out]
          }
          frame condition #1 {
          }
        }
        n1563 = To Variant(anything=T3."mux6-1_channel0" ("mux6_1(3wires)_encode")) -> (Variant=w3586:variant)
        n1564 = To Variant(anything=T3."mux6_1_channel4_3" ("mux6_1(3wires)_encode")) -> (Variant=w3602:variant)
        n1565 = To Variant(anything=T3."mux6_1_channel4_2" ("mux6_1(3wires)_encode")) -> (Variant=w3600:variant)
        n1566 = Bundle By Name(cluster=w3589, "command"=w3587, "command data"=w3600) -> (w3599:T10)
        n1567 = Bundle By Name(cluster=w3589, "command"=w3587, "command data"=w3602) -> (w3598:T10)
        n1568 = Bundle By Name(cluster=w3589, "command"=w3587, "command data"=w3586) -> (w3588:T10)
        n1569 = Bundle By Name(cluster=w3589, "command"="MEAS.DMM dual read") -> (w3596:T10)
        n1570 = Build Array(w3599, w3598, w3596, w3588) -> (w3594:T10[])
        n1571 = Reverse 1D Array(array=w3594) -> (reversed array=w3595:T10[])
        n1572 = for {
          tunnel: [w3622] -> w3607 mode=indexing
          tunnel: w3604 -> [w3621]
          tunnel: w3595 -> [w3620] mode=indexing
          n1573 = Unbundle By Name(w3620) -> ("command"=w3619:string, "command data"=w3618:variant)
          n1574 = call "App enquece.vi"("Priority Enquece"=TRUE, "command data"=w3618, "command"=w3619, "queue in"=w3621) -> ("error out"=w3622:errorcluster)  [unwired: 6 in, 1 out]
        }
        n1575 = Merge Errors(w3605, w3607) -> (w3606:errorcluster)
      }
      frame "Test DRV 29" {
        w3630 = 28  # DUT index(0-59)
        w3627 = T10 {"command"="", "command data"=variant} ("element")
        w3625 = "MEAS.mux6_1"
        n1576 = disable-structure shown="LOGGING==TRUE" {
          disable-tunnel: w3629 -> [w3651 _]
          frame condition #0 (active) {
            n1577 = Empty String/Path?(string/path=w3651) -> (empty?=w3654:bool)
            n1578 = Select(t="Quece timeout", s=w3654, f=w3651) -> (s? t:f=w3650:string)
            n1579 = call "string log (SubVI).vi"("Enum"=enum16{"Init", "Log", "Read"}."Log", "state Name"=w3650) -> ()  [unwired: 8 in, 2 out]
          }
          frame condition #1 {
          }
        }
        n1580 = To Variant(anything=T3."mux6-1_channel0" ("mux6_1(3wires)_encode")) -> (Variant=w3624:variant)
        n1581 = To Variant(anything=T3."mux6_1_channel5_3" ("mux6_1(3wires)_encode")) -> (Variant=w3640:variant)
        n1582 = To Variant(anything=T3."mux6_1_channel5_2" ("mux6_1(3wires)_encode")) -> (Variant=w3638:variant)
        n1583 = Bundle By Name(cluster=w3627, "command"=w3625, "command data"=w3638) -> (w3637:T10)
        n1584 = Bundle By Name(cluster=w3627, "command"=w3625, "command data"=w3640) -> (w3636:T10)
        n1585 = Bundle By Name(cluster=w3627, "command"=w3625, "command data"=w3624) -> (w3626:T10)
        n1586 = Bundle By Name(cluster=w3627, "command"="MEAS.DMM dual read") -> (w3634:T10)
        n1587 = Build Array(w3637, w3636, w3634, w3626) -> (w3632:T10[])
        n1588 = Reverse 1D Array(array=w3632) -> (reversed array=w3633:T10[])
        n1589 = for {
          tunnel: [w3660] -> w3645 mode=indexing
          tunnel: w3642 -> [w3659]
          tunnel: w3633 -> [w3658] mode=indexing
          n1590 = Unbundle By Name(w3658) -> ("command"=w3657:string, "command data"=w3656:variant)
          n1591 = call "App enquece.vi"("Priority Enquece"=TRUE, "command data"=w3656, "command"=w3657, "queue in"=w3659) -> ("error out"=w3660:errorcluster)  [unwired: 6 in, 1 out]
        }
        n1592 = Merge Errors(w3643, w3645) -> (w3644:errorcluster)
      }
      frame "Test DRV 30" {
        w3668 = 29  # DUT index(0-59)
        w3665 = T10 {"command"="", "command data"=variant} ("element")
        w3663 = "MEAS.mux6_1"
        n1593 = disable-structure shown="LOGGING==TRUE" {
          disable-tunnel: w3667 -> [w3689 _]
          frame condition #0 (active) {
            n1594 = Empty String/Path?(string/path=w3689) -> (empty?=w3692:bool)
            n1595 = Select(t="Quece timeout", s=w3692, f=w3689) -> (s? t:f=w3688:string)
            n1596 = call "string log (SubVI).vi"("Enum"=enum16{"Init", "Log", "Read"}."Log", "state Name"=w3688) -> ()  [unwired: 8 in, 2 out]
          }
          frame condition #1 {
          }
        }
        n1597 = To Variant(anything=T3."mux6-1_channel0" ("mux6_1(3wires)_encode")) -> (Variant=w3662:variant)
        n1598 = To Variant(anything=T3."mux6_1_channel6_3" ("mux6_1(3wires)_encode")) -> (Variant=w3678:variant)
        n1599 = To Variant(anything=T3."mux6_1_channel6_2" ("mux6_1(3wires)_encode")) -> (Variant=w3676:variant)
        n1600 = Bundle By Name(cluster=w3665, "command"=w3663, "command data"=w3676) -> (w3675:T10)
        n1601 = Bundle By Name(cluster=w3665, "command"=w3663, "command data"=w3678) -> (w3674:T10)
        n1602 = Bundle By Name(cluster=w3665, "command"=w3663, "command data"=w3662) -> (w3664:T10)
        n1603 = Bundle By Name(cluster=w3665, "command"="MEAS.DMM dual read") -> (w3672:T10)
        n1604 = Build Array(w3675, w3674, w3672, w3664) -> (w3670:T10[])
        n1605 = Reverse 1D Array(array=w3670) -> (reversed array=w3671:T10[])
        n1606 = for {
          tunnel: [w3698] -> w3683 mode=indexing
          tunnel: w3680 -> [w3697]
          tunnel: w3671 -> [w3696] mode=indexing
          n1607 = Unbundle By Name(w3696) -> ("command"=w3695:string, "command data"=w3694:variant)
          n1608 = call "App enquece.vi"("Priority Enquece"=TRUE, "command data"=w3694, "command"=w3695, "queue in"=w3697) -> ("error out"=w3698:errorcluster)  [unwired: 6 in, 1 out]
        }
        n1609 = Merge Errors(w3681, w3683) -> (w3682:errorcluster)
      }
      frame "Test DRV 31" {
        w3706 = 30  # DUT index(0-59)
        w3703 = T10 {"command"="", "command data"=variant} ("element")
        w3701 = "MEAS.mux6_1"
        n1610 = disable-structure shown="LOGGING==TRUE" {
          disable-tunnel: w3705 -> [w3727 _]
          frame condition #0 (active) {
            n1611 = Empty String/Path?(string/path=w3727) -> (empty?=w3730:bool)
            n1612 = Select(t="Quece timeout", s=w3730, f=w3727) -> (s? t:f=w3726:string)
            n1613 = call "string log (SubVI).vi"("Enum"=enum16{"Init", "Log", "Read"}."Log", "state Name"=w3726) -> ()  [unwired: 8 in, 2 out]
          }
          frame condition #1 {
          }
        }
        n1614 = To Variant(anything=T3."mux6-1_channel0" ("mux6_1(3wires)_encode")) -> (Variant=w3700:variant)
        n1615 = To Variant(anything=T3."mux6_1_channel1_3" ("mux6_1(3wires)_encode")) -> (Variant=w3716:variant)
        n1616 = To Variant(anything=T3."mux6-1_channel1_2" ("mux6_1(3wires)_encode")) -> (Variant=w3714:variant)
        n1617 = Bundle By Name(cluster=w3703, "command"=w3701, "command data"=w3714) -> (w3713:T10)
        n1618 = Bundle By Name(cluster=w3703, "command"=w3701, "command data"=w3716) -> (w3712:T10)
        n1619 = Bundle By Name(cluster=w3703, "command"=w3701, "command data"=w3700) -> (w3702:T10)
        n1620 = Bundle By Name(cluster=w3703, "command"="MEAS.DMM dual read") -> (w3710:T10)
        n1621 = Build Array(w3713, w3712, w3710, w3702) -> (w3708:T10[])
        n1622 = Reverse 1D Array(array=w3708) -> (reversed array=w3709:T10[])
        n1623 = for {
          tunnel: [w3736] -> w3721 mode=indexing
          tunnel: w3718 -> [w3735]
          tunnel: w3709 -> [w3734] mode=indexing
          n1624 = Unbundle By Name(w3734) -> ("command"=w3733:string, "command data"=w3732:variant)
          n1625 = call "App enquece.vi"("Priority Enquece"=TRUE, "command data"=w3732, "command"=w3733, "queue in"=w3735) -> ("error out"=w3736:errorcluster)  [unwired: 6 in, 1 out]
        }
        n1626 = Merge Errors(w3719, w3721) -> (w3720:errorcluster)
      }
      frame "Test DRV 32" {
        w3744 = 31  # DUT index(0-59)
        w3741 = T10 {"command"="", "command data"=variant} ("element")
        w3739 = "MEAS.mux6_1"
        n1627 = disable-structure shown="LOGGING==TRUE" {
          disable-tunnel: w3743 -> [w3765 _]
          frame condition #0 (active) {
            n1628 = Empty String/Path?(string/path=w3765) -> (empty?=w3768:bool)
            n1629 = Select(t="Quece timeout", s=w3768, f=w3765) -> (s? t:f=w3764:string)
            n1630 = call "string log (SubVI).vi"("Enum"=enum16{"Init", "Log", "Read"}."Log", "state Name"=w3764) -> ()  [unwired: 8 in, 2 out]
          }
          frame condition #1 {
          }
        }
        n1631 = To Variant(anything=T3."mux6-1_channel0" ("mux6_1(3wires)_encode")) -> (Variant=w3738:variant)
        n1632 = To Variant(anything=T3."mux6_1_channel2_3" ("mux6_1(3wires)_encode")) -> (Variant=w3754:variant)
        n1633 = To Variant(anything=T3."mux6_1_channel2_2" ("mux6_1(3wires)_encode")) -> (Variant=w3752:variant)
        n1634 = Bundle By Name(cluster=w3741, "command"=w3739, "command data"=w3752) -> (w3751:T10)
        n1635 = Bundle By Name(cluster=w3741, "command"=w3739, "command data"=w3754) -> (w3750:T10)
        n1636 = Bundle By Name(cluster=w3741, "command"=w3739, "command data"=w3738) -> (w3740:T10)
        n1637 = Bundle By Name(cluster=w3741, "command"="MEAS.DMM dual read") -> (w3748:T10)
        n1638 = Build Array(w3751, w3750, w3748, w3740) -> (w3746:T10[])
        n1639 = Reverse 1D Array(array=w3746) -> (reversed array=w3747:T10[])
        n1640 = for {
          tunnel: [w3774] -> w3759 mode=indexing
          tunnel: w3756 -> [w3773]
          tunnel: w3747 -> [w3772] mode=indexing
          n1641 = Unbundle By Name(w3772) -> ("command"=w3771:string, "command data"=w3770:variant)
          n1642 = call "App enquece.vi"("Priority Enquece"=TRUE, "command data"=w3770, "command"=w3771, "queue in"=w3773) -> ("error out"=w3774:errorcluster)  [unwired: 6 in, 1 out]
        }
        n1643 = Merge Errors(w3757, w3759) -> (w3758:errorcluster)
      }
      frame "Test DRV 33" {
        w3782 = 32  # DUT index(0-59)
        w3779 = T10 {"command"="", "command data"=variant} ("element")
        w3777 = "MEAS.mux6_1"
        n1644 = disable-structure shown="LOGGING==TRUE" {
          disable-tunnel: w3781 -> [w3803 _]
          frame condition #0 (active) {
            n1645 = Empty String/Path?(string/path=w3803) -> (empty?=w3806:bool)
            n1646 = Select(t="Quece timeout", s=w3806, f=w3803) -> (s? t:f=w3802:string)
            n1647 = call "string log (SubVI).vi"("Enum"=enum16{"Init", "Log", "Read"}."Log", "state Name"=w3802) -> ()  [unwired: 8 in, 2 out]
          }
          frame condition #1 {
          }
        }
        n1648 = To Variant(anything=T3."mux6-1_channel0" ("mux6_1(3wires)_encode")) -> (Variant=w3776:variant)
        n1649 = To Variant(anything=T3."mux6_1_channel3_3" ("mux6_1(3wires)_encode")) -> (Variant=w3792:variant)
        n1650 = To Variant(anything=T3."mux6_1_channel3_2" ("mux6_1(3wires)_encode")) -> (Variant=w3790:variant)
        n1651 = Bundle By Name(cluster=w3779, "command"=w3777, "command data"=w3790) -> (w3789:T10)
        n1652 = Bundle By Name(cluster=w3779, "command"=w3777, "command data"=w3792) -> (w3788:T10)
        n1653 = Bundle By Name(cluster=w3779, "command"=w3777, "command data"=w3776) -> (w3778:T10)
        n1654 = Bundle By Name(cluster=w3779, "command"="MEAS.DMM dual read") -> (w3786:T10)
        n1655 = Build Array(w3789, w3788, w3786, w3778) -> (w3784:T10[])
        n1656 = Reverse 1D Array(array=w3784) -> (reversed array=w3785:T10[])
        n1657 = for {
          tunnel: [w3812] -> w3797 mode=indexing
          tunnel: w3794 -> [w3811]
          tunnel: w3785 -> [w3810] mode=indexing
          n1658 = Unbundle By Name(w3810) -> ("command"=w3809:string, "command data"=w3808:variant)
          n1659 = call "App enquece.vi"("Priority Enquece"=TRUE, "command data"=w3808, "command"=w3809, "queue in"=w3811) -> ("error out"=w3812:errorcluster)  [unwired: 6 in, 1 out]
        }
        n1660 = Merge Errors(w3795, w3797) -> (w3796:errorcluster)
      }
      frame "Test DRV 34" {
        w3820 = 33  # DUT index(0-59)
        w3817 = T10 {"command"="", "command data"=variant} ("element")
        w3815 = "MEAS.mux6_1"
        n1661 = disable-structure shown="LOGGING==TRUE" {
          disable-tunnel: w3819 -> [w3841 _]
          frame condition #0 (active) {
            n1662 = Empty String/Path?(string/path=w3841) -> (empty?=w3844:bool)
            n1663 = Select(t="Quece timeout", s=w3844, f=w3841) -> (s? t:f=w3840:string)
            n1664 = call "string log (SubVI).vi"("Enum"=enum16{"Init", "Log", "Read"}."Log", "state Name"=w3840) -> ()  [unwired: 8 in, 2 out]
          }
          frame condition #1 {
          }
        }
        n1665 = To Variant(anything=T3."mux6-1_channel0" ("mux6_1(3wires)_encode")) -> (Variant=w3814:variant)
        n1666 = To Variant(anything=T3."mux6_1_channel4_3" ("mux6_1(3wires)_encode")) -> (Variant=w3830:variant)
        n1667 = To Variant(anything=T3."mux6_1_channel4_2" ("mux6_1(3wires)_encode")) -> (Variant=w3828:variant)
        n1668 = Bundle By Name(cluster=w3817, "command"=w3815, "command data"=w3828) -> (w3827:T10)
        n1669 = Bundle By Name(cluster=w3817, "command"=w3815, "command data"=w3830) -> (w3826:T10)
        n1670 = Bundle By Name(cluster=w3817, "command"=w3815, "command data"=w3814) -> (w3816:T10)
        n1671 = Bundle By Name(cluster=w3817, "command"="MEAS.DMM dual read") -> (w3824:T10)
        n1672 = Build Array(w3827, w3826, w3824, w3816) -> (w3822:T10[])
        n1673 = Reverse 1D Array(array=w3822) -> (reversed array=w3823:T10[])
        n1674 = for {
          tunnel: [w3850] -> w3835 mode=indexing
          tunnel: w3832 -> [w3849]
          tunnel: w3823 -> [w3848] mode=indexing
          n1675 = Unbundle By Name(w3848) -> ("command"=w3847:string, "command data"=w3846:variant)
          n1676 = call "App enquece.vi"("Priority Enquece"=TRUE, "command data"=w3846, "command"=w3847, "queue in"=w3849) -> ("error out"=w3850:errorcluster)  [unwired: 6 in, 1 out]
        }
        n1677 = Merge Errors(w3833, w3835) -> (w3834:errorcluster)
      }
      frame "Test DRV 35" {
        w3858 = 34  # DUT index(0-59)
        w3855 = T10 {"command"="", "command data"=variant} ("element")
        w3853 = "MEAS.mux6_1"
        n1678 = disable-structure shown="LOGGING==TRUE" {
          disable-tunnel: w3857 -> [w3879 _]
          frame condition #0 (active) {
            n1679 = Empty String/Path?(string/path=w3879) -> (empty?=w3882:bool)
            n1680 = Select(t="Quece timeout", s=w3882, f=w3879) -> (s? t:f=w3878:string)
            n1681 = call "string log (SubVI).vi"("Enum"=enum16{"Init", "Log", "Read"}."Log", "state Name"=w3878) -> ()  [unwired: 8 in, 2 out]
          }
          frame condition #1 {
          }
        }
        n1682 = To Variant(anything=T3."mux6-1_channel0" ("mux6_1(3wires)_encode")) -> (Variant=w3852:variant)
        n1683 = To Variant(anything=T3."mux6_1_channel5_3" ("mux6_1(3wires)_encode")) -> (Variant=w3868:variant)
        n1684 = To Variant(anything=T3."mux6_1_channel5_2" ("mux6_1(3wires)_encode")) -> (Variant=w3866:variant)
        n1685 = Bundle By Name(cluster=w3855, "command"=w3853, "command data"=w3866) -> (w3865:T10)
        n1686 = Bundle By Name(cluster=w3855, "command"=w3853, "command data"=w3868) -> (w3864:T10)
        n1687 = Bundle By Name(cluster=w3855, "command"=w3853, "command data"=w3852) -> (w3854:T10)
        n1688 = Bundle By Name(cluster=w3855, "command"="MEAS.DMM dual read") -> (w3862:T10)
        n1689 = Build Array(w3865, w3864, w3862, w3854) -> (w3860:T10[])
        n1690 = Reverse 1D Array(array=w3860) -> (reversed array=w3861:T10[])
        n1691 = for {
          tunnel: [w3888] -> w3873 mode=indexing
          tunnel: w3870 -> [w3887]
          tunnel: w3861 -> [w3886] mode=indexing
          n1692 = Unbundle By Name(w3886) -> ("command"=w3885:string, "command data"=w3884:variant)
          n1693 = call "App enquece.vi"("Priority Enquece"=TRUE, "command data"=w3884, "command"=w3885, "queue in"=w3887) -> ("error out"=w3888:errorcluster)  [unwired: 6 in, 1 out]
        }
        n1694 = Merge Errors(w3871, w3873) -> (w3872:errorcluster)
      }
      frame "Test DRV 36" {
        w3896 = 35  # DUT index(0-59)
        w3893 = T10 {"command"="", "command data"=variant} ("element")
        w3891 = "MEAS.mux6_1"
        n1695 = disable-structure shown="LOGGING==TRUE" {
          disable-tunnel: w3895 -> [w3917 _]
          frame condition #0 (active) {
            n1696 = Empty String/Path?(string/path=w3917) -> (empty?=w3920:bool)
            n1697 = Select(t="Quece timeout", s=w3920, f=w3917) -> (s? t:f=w3916:string)
            n1698 = call "string log (SubVI).vi"("Enum"=enum16{"Init", "Log", "Read"}."Log", "state Name"=w3916) -> ()  [unwired: 8 in, 2 out]
          }
          frame condition #1 {
          }
        }
        n1699 = To Variant(anything=T3."mux6-1_channel0" ("mux6_1(3wires)_encode")) -> (Variant=w3890:variant)
        n1700 = To Variant(anything=T3."mux6_1_channel6_3" ("mux6_1(3wires)_encode")) -> (Variant=w3906:variant)
        n1701 = To Variant(anything=T3."mux6_1_channel6_2" ("mux6_1(3wires)_encode")) -> (Variant=w3904:variant)
        n1702 = Bundle By Name(cluster=w3893, "command"=w3891, "command data"=w3904) -> (w3903:T10)
        n1703 = Bundle By Name(cluster=w3893, "command"=w3891, "command data"=w3906) -> (w3902:T10)
        n1704 = Bundle By Name(cluster=w3893, "command"=w3891, "command data"=w3890) -> (w3892:T10)
        n1705 = Bundle By Name(cluster=w3893, "command"="MEAS.DMM dual read") -> (w3900:T10)
        n1706 = Build Array(w3903, w3902, w3900, w3892) -> (w3898:T10[])
        n1707 = Reverse 1D Array(array=w3898) -> (reversed array=w3899:T10[])
        n1708 = for {
          tunnel: [w3926] -> w3911 mode=indexing
          tunnel: w3908 -> [w3925]
          tunnel: w3899 -> [w3924] mode=indexing
          n1709 = Unbundle By Name(w3924) -> ("command"=w3923:string, "command data"=w3922:variant)
          n1710 = call "App enquece.vi"("Priority Enquece"=TRUE, "command data"=w3922, "command"=w3923, "queue in"=w3925) -> ("error out"=w3926:errorcluster)  [unwired: 6 in, 1 out]
        }
        n1711 = Merge Errors(w3909, w3911) -> (w3910:errorcluster)
      }
      frame "Test DRV 37" {
        w3934 = 36  # DUT index(0-59)
        w3931 = T10 {"command"="", "command data"=variant} ("element")
        w3929 = "MEAS.mux6_1"
        n1712 = disable-structure shown="LOGGING==TRUE" {
          disable-tunnel: w3933 -> [w3955 _]
          frame condition #0 (active) {
            n1713 = Empty String/Path?(string/path=w3955) -> (empty?=w3958:bool)
            n1714 = Select(t="Quece timeout", s=w3958, f=w3955) -> (s? t:f=w3954:string)
            n1715 = call "string log (SubVI).vi"("Enum"=enum16{"Init", "Log", "Read"}."Log", "state Name"=w3954) -> ()  [unwired: 8 in, 2 out]
          }
          frame condition #1 {
          }
        }
        n1716 = To Variant(anything=T3."mux6-1_channel0" ("mux6_1(3wires)_encode")) -> (Variant=w3928:variant)
        n1717 = To Variant(anything=T3."mux6_1_channel1_3" ("mux6_1(3wires)_encode")) -> (Variant=w3944:variant)
        n1718 = To Variant(anything=T3."mux6-1_channel1_2" ("mux6_1(3wires)_encode")) -> (Variant=w3942:variant)
        n1719 = Bundle By Name(cluster=w3931, "command"=w3929, "command data"=w3942) -> (w3941:T10)
        n1720 = Bundle By Name(cluster=w3931, "command"=w3929, "command data"=w3944) -> (w3940:T10)
        n1721 = Bundle By Name(cluster=w3931, "command"=w3929, "command data"=w3928) -> (w3930:T10)
        n1722 = Bundle By Name(cluster=w3931, "command"="MEAS.DMM dual read") -> (w3938:T10)
        n1723 = Build Array(w3941, w3940, w3938, w3930) -> (w3936:T10[])
        n1724 = Reverse 1D Array(array=w3936) -> (reversed array=w3937:T10[])
        n1725 = for {
          tunnel: [w3964] -> w3949 mode=indexing
          tunnel: w3946 -> [w3963]
          tunnel: w3937 -> [w3962] mode=indexing
          n1726 = Unbundle By Name(w3962) -> ("command"=w3961:string, "command data"=w3960:variant)
          n1727 = call "App enquece.vi"("Priority Enquece"=TRUE, "command data"=w3960, "command"=w3961, "queue in"=w3963) -> ("error out"=w3964:errorcluster)  [unwired: 6 in, 1 out]
        }
        n1728 = Merge Errors(w3947, w3949) -> (w3948:errorcluster)
      }
      frame "Test DRV 38" {
        w3972 = 37  # DUT index(0-59)
        w3969 = T10 {"command"="", "command data"=variant} ("element")
        w3967 = "MEAS.mux6_1"
        n1729 = disable-structure shown="LOGGING==TRUE" {
          disable-tunnel: w3971 -> [w3993 _]
          frame condition #0 (active) {
            n1730 = Empty String/Path?(string/path=w3993) -> (empty?=w3996:bool)
            n1731 = Select(t="Quece timeout", s=w3996, f=w3993) -> (s? t:f=w3992:string)
            n1732 = call "string log (SubVI).vi"("Enum"=enum16{"Init", "Log", "Read"}."Log", "state Name"=w3992) -> ()  [unwired: 8 in, 2 out]
          }
          frame condition #1 {
          }
        }
        n1733 = To Variant(anything=T3."mux6-1_channel0" ("mux6_1(3wires)_encode")) -> (Variant=w3966:variant)
        n1734 = To Variant(anything=T3."mux6_1_channel2_3" ("mux6_1(3wires)_encode")) -> (Variant=w3982:variant)
        n1735 = To Variant(anything=T3."mux6_1_channel2_2" ("mux6_1(3wires)_encode")) -> (Variant=w3980:variant)
        n1736 = Bundle By Name(cluster=w3969, "command"=w3967, "command data"=w3980) -> (w3979:T10)
        n1737 = Bundle By Name(cluster=w3969, "command"=w3967, "command data"=w3982) -> (w3978:T10)
        n1738 = Bundle By Name(cluster=w3969, "command"=w3967, "command data"=w3966) -> (w3968:T10)
        n1739 = Bundle By Name(cluster=w3969, "command"="MEAS.DMM dual read") -> (w3976:T10)
        n1740 = Build Array(w3979, w3978, w3976, w3968) -> (w3974:T10[])
        n1741 = Reverse 1D Array(array=w3974) -> (reversed array=w3975:T10[])
        n1742 = for {
          tunnel: [w4002] -> w3987 mode=indexing
          tunnel: w3984 -> [w4001]
          tunnel: w3975 -> [w4000] mode=indexing
          n1743 = Unbundle By Name(w4000) -> ("command"=w3999:string, "command data"=w3998:variant)
          n1744 = call "App enquece.vi"("Priority Enquece"=TRUE, "command data"=w3998, "command"=w3999, "queue in"=w4001) -> ("error out"=w4002:errorcluster)  [unwired: 6 in, 1 out]
        }
        n1745 = Merge Errors(w3985, w3987) -> (w3986:errorcluster)
      }
      frame "Test DRV 39" {
        w4010 = 38  # DUT index(0-59)
        w4007 = T10 {"command"="", "command data"=variant} ("element")
        w4005 = "MEAS.mux6_1"
        n1746 = disable-structure shown="LOGGING==TRUE" {
          disable-tunnel: w4009 -> [w4031 _]
          frame condition #0 (active) {
            n1747 = Empty String/Path?(string/path=w4031) -> (empty?=w4034:bool)
            n1748 = Select(t="Quece timeout", s=w4034, f=w4031) -> (s? t:f=w4030:string)
            n1749 = call "string log (SubVI).vi"("Enum"=enum16{"Init", "Log", "Read"}."Log", "state Name"=w4030) -> ()  [unwired: 8 in, 2 out]
          }
          frame condition #1 {
          }
        }
        n1750 = To Variant(anything=T3."mux6-1_channel0" ("mux6_1(3wires)_encode")) -> (Variant=w4004:variant)
        n1751 = To Variant(anything=T3."mux6_1_channel3_3" ("mux6_1(3wires)_encode")) -> (Variant=w4020:variant)
        n1752 = To Variant(anything=T3."mux6_1_channel3_2" ("mux6_1(3wires)_encode")) -> (Variant=w4018:variant)
        n1753 = Bundle By Name(cluster=w4007, "command"=w4005, "command data"=w4018) -> (w4017:T10)
        n1754 = Bundle By Name(cluster=w4007, "command"=w4005, "command data"=w4020) -> (w4016:T10)
        n1755 = Bundle By Name(cluster=w4007, "command"=w4005, "command data"=w4004) -> (w4006:T10)
        n1756 = Bundle By Name(cluster=w4007, "command"="MEAS.DMM dual read") -> (w4014:T10)
        n1757 = Build Array(w4017, w4016, w4014, w4006) -> (w4012:T10[])
        n1758 = Reverse 1D Array(array=w4012) -> (reversed array=w4013:T10[])
        n1759 = for {
          tunnel: [w4040] -> w4025 mode=indexing
          tunnel: w4022 -> [w4039]
          tunnel: w4013 -> [w4038] mode=indexing
          n1760 = Unbundle By Name(w4038) -> ("command"=w4037:string, "command data"=w4036:variant)
          n1761 = call "App enquece.vi"("Priority Enquece"=TRUE, "command data"=w4036, "command"=w4037, "queue in"=w4039) -> ("error out"=w4040:errorcluster)  [unwired: 6 in, 1 out]
        }
        n1762 = Merge Errors(w4023, w4025) -> (w4024:errorcluster)
      }
      frame "Test DRV 40" {
        w4048 = 39  # DUT index(0-59)
        w4045 = T10 {"command"="", "command data"=variant} ("element")
        w4043 = "MEAS.mux6_1"
        n1763 = disable-structure shown="LOGGING==TRUE" {
          disable-tunnel: w4047 -> [w4069 _]
          frame condition #0 (active) {
            n1764 = Empty String/Path?(string/path=w4069) -> (empty?=w4072:bool)
            n1765 = Select(t="Quece timeout", s=w4072, f=w4069) -> (s? t:f=w4068:string)
            n1766 = call "string log (SubVI).vi"("Enum"=enum16{"Init", "Log", "Read"}."Log", "state Name"=w4068) -> ()  [unwired: 8 in, 2 out]
          }
          frame condition #1 {
          }
        }
        n1767 = To Variant(anything=T3."mux6-1_channel0" ("mux6_1(3wires)_encode")) -> (Variant=w4042:variant)
        n1768 = To Variant(anything=T3."mux6_1_channel4_3" ("mux6_1(3wires)_encode")) -> (Variant=w4058:variant)
        n1769 = To Variant(anything=T3."mux6_1_channel4_2" ("mux6_1(3wires)_encode")) -> (Variant=w4056:variant)
        n1770 = Bundle By Name(cluster=w4045, "command"=w4043, "command data"=w4056) -> (w4055:T10)
        n1771 = Bundle By Name(cluster=w4045, "command"=w4043, "command data"=w4058) -> (w4054:T10)
        n1772 = Bundle By Name(cluster=w4045, "command"=w4043, "command data"=w4042) -> (w4044:T10)
        n1773 = Bundle By Name(cluster=w4045, "command"="MEAS.DMM dual read") -> (w4052:T10)
        n1774 = Build Array(w4055, w4054, w4052, w4044) -> (w4050:T10[])
        n1775 = Reverse 1D Array(array=w4050) -> (reversed array=w4051:T10[])
        n1776 = for {
          tunnel: [w4078] -> w4063 mode=indexing
          tunnel: w4060 -> [w4077]
          tunnel: w4051 -> [w4076] mode=indexing
          n1777 = Unbundle By Name(w4076) -> ("command"=w4075:string, "command data"=w4074:variant)
          n1778 = call "App enquece.vi"("Priority Enquece"=TRUE, "command data"=w4074, "command"=w4075, "queue in"=w4077) -> ("error out"=w4078:errorcluster)  [unwired: 6 in, 1 out]
        }
        n1779 = Merge Errors(w4061, w4063) -> (w4062:errorcluster)
      }
      frame "Test DRV 41" {
        w4086 = 40  # DUT index(0-59)
        w4083 = T10 {"command"="", "command data"=variant} ("element")
        w4081 = "MEAS.mux6_1"
        n1780 = disable-structure shown="LOGGING==TRUE" {
          disable-tunnel: w4085 -> [w4107 _]
          frame condition #0 (active) {
            n1781 = Empty String/Path?(string/path=w4107) -> (empty?=w4110:bool)
            n1782 = Select(t="Quece timeout", s=w4110, f=w4107) -> (s? t:f=w4106:string)
            n1783 = call "string log (SubVI).vi"("Enum"=enum16{"Init", "Log", "Read"}."Log", "state Name"=w4106) -> ()  [unwired: 8 in, 2 out]
          }
          frame condition #1 {
          }
        }
        n1784 = To Variant(anything=T3."mux6-1_channel0" ("mux6_1(3wires)_encode")) -> (Variant=w4080:variant)
        n1785 = To Variant(anything=T3."mux6_1_channel5_3" ("mux6_1(3wires)_encode")) -> (Variant=w4096:variant)
        n1786 = To Variant(anything=T3."mux6_1_channel5_2" ("mux6_1(3wires)_encode")) -> (Variant=w4094:variant)
        n1787 = Bundle By Name(cluster=w4083, "command"=w4081, "command data"=w4094) -> (w4093:T10)
        n1788 = Bundle By Name(cluster=w4083, "command"=w4081, "command data"=w4096) -> (w4092:T10)
        n1789 = Bundle By Name(cluster=w4083, "command"=w4081, "command data"=w4080) -> (w4082:T10)
        n1790 = Bundle By Name(cluster=w4083, "command"="MEAS.DMM dual read") -> (w4090:T10)
        n1791 = Build Array(w4093, w4092, w4090, w4082) -> (w4088:T10[])
        n1792 = Reverse 1D Array(array=w4088) -> (reversed array=w4089:T10[])
        n1793 = for {
          tunnel: [w4116] -> w4101 mode=indexing
          tunnel: w4098 -> [w4115]
          tunnel: w4089 -> [w4114] mode=indexing
          n1794 = Unbundle By Name(w4114) -> ("command"=w4113:string, "command data"=w4112:variant)
          n1795 = call "App enquece.vi"("Priority Enquece"=TRUE, "command data"=w4112, "command"=w4113, "queue in"=w4115) -> ("error out"=w4116:errorcluster)  [unwired: 6 in, 1 out]
        }
        n1796 = Merge Errors(w4099, w4101) -> (w4100:errorcluster)
      }
      frame "Test DRV 42" {
        w4124 = 41  # DUT index(0-59)
        w4121 = T10 {"command"="", "command data"=variant} ("element")
        w4119 = "MEAS.mux6_1"
        n1797 = disable-structure shown="LOGGING==TRUE" {
          disable-tunnel: w4123 -> [w4145 _]
          frame condition #0 (active) {
            n1798 = Empty String/Path?(string/path=w4145) -> (empty?=w4148:bool)
            n1799 = Select(t="Quece timeout", s=w4148, f=w4145) -> (s? t:f=w4144:string)
            n1800 = call "string log (SubVI).vi"("Enum"=enum16{"Init", "Log", "Read"}."Log", "state Name"=w4144) -> ()  [unwired: 8 in, 2 out]
          }
          frame condition #1 {
          }
        }
        n1801 = To Variant(anything=T3."mux6-1_channel0" ("mux6_1(3wires)_encode")) -> (Variant=w4118:variant)
        n1802 = To Variant(anything=T3."mux6_1_channel6_3" ("mux6_1(3wires)_encode")) -> (Variant=w4134:variant)
        n1803 = To Variant(anything=T3."mux6_1_channel6_2" ("mux6_1(3wires)_encode")) -> (Variant=w4132:variant)
        n1804 = Bundle By Name(cluster=w4121, "command"=w4119, "command data"=w4132) -> (w4131:T10)
        n1805 = Bundle By Name(cluster=w4121, "command"=w4119, "command data"=w4134) -> (w4130:T10)
        n1806 = Bundle By Name(cluster=w4121, "command"=w4119, "command data"=w4118) -> (w4120:T10)
        n1807 = Bundle By Name(cluster=w4121, "command"="MEAS.DMM dual read") -> (w4128:T10)
        n1808 = Build Array(w4131, w4130, w4128, w4120) -> (w4126:T10[])
        n1809 = Reverse 1D Array(array=w4126) -> (reversed array=w4127:T10[])
        n1810 = for {
          tunnel: [w4154] -> w4139 mode=indexing
          tunnel: w4136 -> [w4153]
          tunnel: w4127 -> [w4152] mode=indexing
          n1811 = Unbundle By Name(w4152) -> ("command"=w4151:string, "command data"=w4150:variant)
          n1812 = call "App enquece.vi"("Priority Enquece"=TRUE, "command data"=w4150, "command"=w4151, "queue in"=w4153) -> ("error out"=w4154:errorcluster)  [unwired: 6 in, 1 out]
        }
        n1813 = Merge Errors(w4137, w4139) -> (w4138:errorcluster)
      }
      frame "Test DRV 43" {
        w4162 = 42  # DUT index(0-59)
        w4159 = T10 {"command"="", "command data"=variant} ("element")
        w4157 = "MEAS.mux6_1"
        n1814 = disable-structure shown="LOGGING==TRUE" {
          disable-tunnel: w4161 -> [w4183 _]
          frame condition #0 (active) {
            n1815 = Empty String/Path?(string/path=w4183) -> (empty?=w4186:bool)
            n1816 = Select(t="Quece timeout", s=w4186, f=w4183) -> (s? t:f=w4182:string)
            n1817 = call "string log (SubVI).vi"("Enum"=enum16{"Init", "Log", "Read"}."Log", "state Name"=w4182) -> ()  [unwired: 8 in, 2 out]
          }
          frame condition #1 {
          }
        }
        n1818 = To Variant(anything=T3."mux6-1_channel0" ("mux6_1(3wires)_encode")) -> (Variant=w4156:variant)
        n1819 = To Variant(anything=T3."mux6_1_channel1_3" ("mux6_1(3wires)_encode")) -> (Variant=w4172:variant)
        n1820 = To Variant(anything=T3."mux6-1_channel1_2" ("mux6_1(3wires)_encode")) -> (Variant=w4170:variant)
        n1821 = Bundle By Name(cluster=w4159, "command"=w4157, "command data"=w4170) -> (w4169:T10)
        n1822 = Bundle By Name(cluster=w4159, "command"=w4157, "command data"=w4172) -> (w4168:T10)
        n1823 = Bundle By Name(cluster=w4159, "command"=w4157, "command data"=w4156) -> (w4158:T10)
        n1824 = Bundle By Name(cluster=w4159, "command"="MEAS.DMM dual read") -> (w4166:T10)
        n1825 = Build Array(w4169, w4168, w4166, w4158) -> (w4164:T10[])
        n1826 = Reverse 1D Array(array=w4164) -> (reversed array=w4165:T10[])
        n1827 = for {
          tunnel: [w4192] -> w4177 mode=indexing
          tunnel: w4174 -> [w4191]
          tunnel: w4165 -> [w4190] mode=indexing
          n1828 = Unbundle By Name(w4190) -> ("command"=w4189:string, "command data"=w4188:variant)
          n1829 = call "App enquece.vi"("Priority Enquece"=TRUE, "command data"=w4188, "command"=w4189, "queue in"=w4191) -> ("error out"=w4192:errorcluster)  [unwired: 6 in, 1 out]
        }
        n1830 = Merge Errors(w4175, w4177) -> (w4176:errorcluster)
      }
      frame "Test DRV 44" {
        w4200 = 43  # DUT index(0-59)
        w4197 = T10 {"command"="", "command data"=variant} ("element")
        w4195 = "MEAS.mux6_1"
        n1831 = disable-structure shown="LOGGING==TRUE" {
          disable-tunnel: w4199 -> [w4221 _]
          frame condition #0 (active) {
            n1832 = Empty String/Path?(string/path=w4221) -> (empty?=w4224:bool)
            n1833 = Select(t="Quece timeout", s=w4224, f=w4221) -> (s? t:f=w4220:string)
            n1834 = call "string log (SubVI).vi"("Enum"=enum16{"Init", "Log", "Read"}."Log", "state Name"=w4220) -> ()  [unwired: 8 in, 2 out]
          }
          frame condition #1 {
          }
        }
        n1835 = To Variant(anything=T3."mux6-1_channel0" ("mux6_1(3wires)_encode")) -> (Variant=w4194:variant)
        n1836 = To Variant(anything=T3."mux6_1_channel2_3" ("mux6_1(3wires)_encode")) -> (Variant=w4210:variant)
        n1837 = To Variant(anything=T3."mux6_1_channel2_2" ("mux6_1(3wires)_encode")) -> (Variant=w4208:variant)
        n1838 = Bundle By Name(cluster=w4197, "command"=w4195, "command data"=w4208) -> (w4207:T10)
        n1839 = Bundle By Name(cluster=w4197, "command"=w4195, "command data"=w4210) -> (w4206:T10)
        n1840 = Bundle By Name(cluster=w4197, "command"=w4195, "command data"=w4194) -> (w4196:T10)
        n1841 = Bundle By Name(cluster=w4197, "command"="MEAS.DMM dual read") -> (w4204:T10)
        n1842 = Build Array(w4207, w4206, w4204, w4196) -> (w4202:T10[])
        n1843 = Reverse 1D Array(array=w4202) -> (reversed array=w4203:T10[])
        n1844 = for {
          tunnel: [w4230] -> w4215 mode=indexing
          tunnel: w4212 -> [w4229]
          tunnel: w4203 -> [w4228] mode=indexing
          n1845 = Unbundle By Name(w4228) -> ("command"=w4227:string, "command data"=w4226:variant)
          n1846 = call "App enquece.vi"("Priority Enquece"=TRUE, "command data"=w4226, "command"=w4227, "queue in"=w4229) -> ("error out"=w4230:errorcluster)  [unwired: 6 in, 1 out]
        }
        n1847 = Merge Errors(w4213, w4215) -> (w4214:errorcluster)
      }
      frame "Test DRV 45" {
        w4238 = 44  # DUT index(0-59)
        w4235 = T10 {"command"="", "command data"=variant} ("element")
        w4233 = "MEAS.mux6_1"
        n1848 = disable-structure shown="LOGGING==TRUE" {
          disable-tunnel: w4237 -> [w4259 _]
          frame condition #0 (active) {
            n1849 = Empty String/Path?(string/path=w4259) -> (empty?=w4262:bool)
            n1850 = Select(t="Quece timeout", s=w4262, f=w4259) -> (s? t:f=w4258:string)
            n1851 = call "string log (SubVI).vi"("Enum"=enum16{"Init", "Log", "Read"}."Log", "state Name"=w4258) -> ()  [unwired: 8 in, 2 out]
          }
          frame condition #1 {
          }
        }
        n1852 = To Variant(anything=T3."mux6-1_channel0" ("mux6_1(3wires)_encode")) -> (Variant=w4232:variant)
        n1853 = To Variant(anything=T3."mux6_1_channel3_3" ("mux6_1(3wires)_encode")) -> (Variant=w4248:variant)
        n1854 = To Variant(anything=T3."mux6_1_channel3_2" ("mux6_1(3wires)_encode")) -> (Variant=w4246:variant)
        n1855 = Bundle By Name(cluster=w4235, "command"=w4233, "command data"=w4246) -> (w4245:T10)
        n1856 = Bundle By Name(cluster=w4235, "command"=w4233, "command data"=w4248) -> (w4244:T10)
        n1857 = Bundle By Name(cluster=w4235, "command"=w4233, "command data"=w4232) -> (w4234:T10)
        n1858 = Bundle By Name(cluster=w4235, "command"="MEAS.DMM dual read") -> (w4242:T10)
        n1859 = Build Array(w4245, w4244, w4242, w4234) -> (w4240:T10[])
        n1860 = Reverse 1D Array(array=w4240) -> (reversed array=w4241:T10[])
        n1861 = for {
          tunnel: [w4268] -> w4253 mode=indexing
          tunnel: w4250 -> [w4267]
          tunnel: w4241 -> [w4266] mode=indexing
          n1862 = Unbundle By Name(w4266) -> ("command"=w4265:string, "command data"=w4264:variant)
          n1863 = call "App enquece.vi"("Priority Enquece"=TRUE, "command data"=w4264, "command"=w4265, "queue in"=w4267) -> ("error out"=w4268:errorcluster)  [unwired: 6 in, 1 out]
        }
        n1864 = Merge Errors(w4251, w4253) -> (w4252:errorcluster)
      }
      frame "Test DRV 46" {
        w4276 = 45  # DUT index(0-59)
        w4273 = T10 {"command"="", "command data"=variant} ("element")
        w4271 = "MEAS.mux6_1"
        n1865 = disable-structure shown="LOGGING==TRUE" {
          disable-tunnel: w4275 -> [w4297 _]
          frame condition #0 (active) {
            n1866 = Empty String/Path?(string/path=w4297) -> (empty?=w4300:bool)
            n1867 = Select(t="Quece timeout", s=w4300, f=w4297) -> (s? t:f=w4296:string)
            n1868 = call "string log (SubVI).vi"("Enum"=enum16{"Init", "Log", "Read"}."Log", "state Name"=w4296) -> ()  [unwired: 8 in, 2 out]
          }
          frame condition #1 {
          }
        }
        n1869 = To Variant(anything=T3."mux6-1_channel0" ("mux6_1(3wires)_encode")) -> (Variant=w4270:variant)
        n1870 = To Variant(anything=T3."mux6_1_channel4_3" ("mux6_1(3wires)_encode")) -> (Variant=w4286:variant)
        n1871 = To Variant(anything=T3."mux6_1_channel4_2" ("mux6_1(3wires)_encode")) -> (Variant=w4284:variant)
        n1872 = Bundle By Name(cluster=w4273, "command"=w4271, "command data"=w4284) -> (w4283:T10)
        n1873 = Bundle By Name(cluster=w4273, "command"=w4271, "command data"=w4286) -> (w4282:T10)
        n1874 = Bundle By Name(cluster=w4273, "command"=w4271, "command data"=w4270) -> (w4272:T10)
        n1875 = Bundle By Name(cluster=w4273, "command"="MEAS.DMM dual read") -> (w4280:T10)
        n1876 = Build Array(w4283, w4282, w4280, w4272) -> (w4278:T10[])
        n1877 = Reverse 1D Array(array=w4278) -> (reversed array=w4279:T10[])
        n1878 = for {
          tunnel: [w4306] -> w4291 mode=indexing
          tunnel: w4288 -> [w4305]
          tunnel: w4279 -> [w4304] mode=indexing
          n1879 = Unbundle By Name(w4304) -> ("command"=w4303:string, "command data"=w4302:variant)
          n1880 = call "App enquece.vi"("Priority Enquece"=TRUE, "command data"=w4302, "command"=w4303, "queue in"=w4305) -> ("error out"=w4306:errorcluster)  [unwired: 6 in, 1 out]
        }
        n1881 = Merge Errors(w4289, w4291) -> (w4290:errorcluster)
      }
      frame "Test DRV 47" {
        w4314 = 46  # DUT index(0-59)
        w4311 = T10 {"command"="", "command data"=variant} ("element")
        w4309 = "MEAS.mux6_1"
        n1882 = disable-structure shown="LOGGING==TRUE" {
          disable-tunnel: w4313 -> [w4335 _]
          frame condition #0 (active) {
            n1883 = Empty String/Path?(string/path=w4335) -> (empty?=w4338:bool)
            n1884 = Select(t="Quece timeout", s=w4338, f=w4335) -> (s? t:f=w4334:string)
            n1885 = call "string log (SubVI).vi"("Enum"=enum16{"Init", "Log", "Read"}."Log", "state Name"=w4334) -> ()  [unwired: 8 in, 2 out]
          }
          frame condition #1 {
          }
        }
        n1886 = To Variant(anything=T3."mux6-1_channel0" ("mux6_1(3wires)_encode")) -> (Variant=w4308:variant)
        n1887 = To Variant(anything=T3."mux6_1_channel5_3" ("mux6_1(3wires)_encode")) -> (Variant=w4324:variant)
        n1888 = To Variant(anything=T3."mux6_1_channel5_2" ("mux6_1(3wires)_encode")) -> (Variant=w4322:variant)
        n1889 = Bundle By Name(cluster=w4311, "command"=w4309, "command data"=w4322) -> (w4321:T10)
        n1890 = Bundle By Name(cluster=w4311, "command"=w4309, "command data"=w4324) -> (w4320:T10)
        n1891 = Bundle By Name(cluster=w4311, "command"=w4309, "command data"=w4308) -> (w4310:T10)
        n1892 = Bundle By Name(cluster=w4311, "command"="MEAS.DMM dual read") -> (w4318:T10)
        n1893 = Build Array(w4321, w4320, w4318, w4310) -> (w4316:T10[])
        n1894 = Reverse 1D Array(array=w4316) -> (reversed array=w4317:T10[])
        n1895 = for {
          tunnel: [w4344] -> w4329 mode=indexing
          tunnel: w4326 -> [w4343]
          tunnel: w4317 -> [w4342] mode=indexing
          n1896 = Unbundle By Name(w4342) -> ("command"=w4341:string, "command data"=w4340:variant)
          n1897 = call "App enquece.vi"("Priority Enquece"=TRUE, "command data"=w4340, "command"=w4341, "queue in"=w4343) -> ("error out"=w4344:errorcluster)  [unwired: 6 in, 1 out]
        }
        n1898 = Merge Errors(w4327, w4329) -> (w4328:errorcluster)
      }
      frame "Test DRV 48" {
        w4352 = 47  # DUT index(0-59)
        w4349 = T10 {"command"="", "command data"=variant} ("element")
        w4347 = "MEAS.mux6_1"
        n1899 = disable-structure shown="LOGGING==TRUE" {
          disable-tunnel: w4351 -> [w4373 _]
          frame condition #0 (active) {
            n1900 = Empty String/Path?(string/path=w4373) -> (empty?=w4376:bool)
            n1901 = Select(t="Quece timeout", s=w4376, f=w4373) -> (s? t:f=w4372:string)
            n1902 = call "string log (SubVI).vi"("Enum"=enum16{"Init", "Log", "Read"}."Log", "state Name"=w4372) -> ()  [unwired: 8 in, 2 out]
          }
          frame condition #1 {
          }
        }
        n1903 = To Variant(anything=T3."mux6-1_channel0" ("mux6_1(3wires)_encode")) -> (Variant=w4346:variant)
        n1904 = To Variant(anything=T3."mux6_1_channel6_3" ("mux6_1(3wires)_encode")) -> (Variant=w4362:variant)
        n1905 = To Variant(anything=T3."mux6_1_channel6_2" ("mux6_1(3wires)_encode")) -> (Variant=w4360:variant)
        n1906 = Bundle By Name(cluster=w4349, "command"=w4347, "command data"=w4360) -> (w4359:T10)
        n1907 = Bundle By Name(cluster=w4349, "command"=w4347, "command data"=w4362) -> (w4358:T10)
        n1908 = Bundle By Name(cluster=w4349, "command"=w4347, "command data"=w4346) -> (w4348:T10)
        n1909 = Bundle By Name(cluster=w4349, "command"="MEAS.DMM dual read") -> (w4356:T10)
        n1910 = Build Array(w4359, w4358, w4356, w4348) -> (w4354:T10[])
        n1911 = Reverse 1D Array(array=w4354) -> (reversed array=w4355:T10[])
        n1912 = for {
          tunnel: [w4382] -> w4367 mode=indexing
          tunnel: w4364 -> [w4381]
          tunnel: w4355 -> [w4380] mode=indexing
          n1913 = Unbundle By Name(w4380) -> ("command"=w4379:string, "command data"=w4378:variant)
          n1914 = call "App enquece.vi"("Priority Enquece"=TRUE, "command data"=w4378, "command"=w4379, "queue in"=w4381) -> ("error out"=w4382:errorcluster)  [unwired: 6 in, 1 out]
        }
        n1915 = Merge Errors(w4365, w4367) -> (w4366:errorcluster)
      }
      frame "Test DRV 49" {
        w4390 = 48  # DUT index(0-59)
        w4387 = T10 {"command"="", "command data"=variant} ("element")
        w4385 = "MEAS.mux6_1"
        n1916 = disable-structure shown="LOGGING==TRUE" {
          disable-tunnel: w4389 -> [w4411 _]
          frame condition #0 (active) {
            n1917 = Empty String/Path?(string/path=w4411) -> (empty?=w4414:bool)
            n1918 = Select(t="Quece timeout", s=w4414, f=w4411) -> (s? t:f=w4410:string)
            n1919 = call "string log (SubVI).vi"("Enum"=enum16{"Init", "Log", "Read"}."Log", "state Name"=w4410) -> ()  [unwired: 8 in, 2 out]
          }
          frame condition #1 {
          }
        }
        n1920 = To Variant(anything=T3."mux6-1_channel0" ("mux6_1(3wires)_encode")) -> (Variant=w4384:variant)
        n1921 = To Variant(anything=T3."mux6_1_channel1_3" ("mux6_1(3wires)_encode")) -> (Variant=w4400:variant)
        n1922 = To Variant(anything=T3."mux6-1_channel1_2" ("mux6_1(3wires)_encode")) -> (Variant=w4398:variant)
        n1923 = Bundle By Name(cluster=w4387, "command"=w4385, "command data"=w4398) -> (w4397:T10)
        n1924 = Bundle By Name(cluster=w4387, "command"=w4385, "command data"=w4400) -> (w4396:T10)
        n1925 = Bundle By Name(cluster=w4387, "command"=w4385, "command data"=w4384) -> (w4386:T10)
        n1926 = Bundle By Name(cluster=w4387, "command"="MEAS.DMM dual read") -> (w4394:T10)
        n1927 = Build Array(w4397, w4396, w4394, w4386) -> (w4392:T10[])
        n1928 = Reverse 1D Array(array=w4392) -> (reversed array=w4393:T10[])
        n1929 = for {
          tunnel: [w4420] -> w4405 mode=indexing
          tunnel: w4402 -> [w4419]
          tunnel: w4393 -> [w4418] mode=indexing
          n1930 = Unbundle By Name(w4418) -> ("command"=w4417:string, "command data"=w4416:variant)
          n1931 = call "App enquece.vi"("Priority Enquece"=TRUE, "command data"=w4416, "command"=w4417, "queue in"=w4419) -> ("error out"=w4420:errorcluster)  [unwired: 6 in, 1 out]
        }
        n1932 = Merge Errors(w4403, w4405) -> (w4404:errorcluster)
      }
      frame "Test DRV 50" {
        w4428 = 49  # DUT index(0-59)
        w4425 = T10 {"command"="", "command data"=variant} ("element")
        w4423 = "MEAS.mux6_1"
        n1933 = disable-structure shown="LOGGING==TRUE" {
          disable-tunnel: w4427 -> [w4449 _]
          frame condition #0 (active) {
            n1934 = Empty String/Path?(string/path=w4449) -> (empty?=w4452:bool)
            n1935 = Select(t="Quece timeout", s=w4452, f=w4449) -> (s? t:f=w4448:string)
            n1936 = call "string log (SubVI).vi"("Enum"=enum16{"Init", "Log", "Read"}."Log", "state Name"=w4448) -> ()  [unwired: 8 in, 2 out]
          }
          frame condition #1 {
          }
        }
        n1937 = To Variant(anything=T3."mux6-1_channel0" ("mux6_1(3wires)_encode")) -> (Variant=w4422:variant)
        n1938 = To Variant(anything=T3."mux6_1_channel2_3" ("mux6_1(3wires)_encode")) -> (Variant=w4438:variant)
        n1939 = To Variant(anything=T3."mux6_1_channel2_2" ("mux6_1(3wires)_encode")) -> (Variant=w4436:variant)
        n1940 = Bundle By Name(cluster=w4425, "command"=w4423, "command data"=w4436) -> (w4435:T10)
        n1941 = Bundle By Name(cluster=w4425, "command"=w4423, "command data"=w4438) -> (w4434:T10)
        n1942 = Bundle By Name(cluster=w4425, "command"=w4423, "command data"=w4422) -> (w4424:T10)
        n1943 = Bundle By Name(cluster=w4425, "command"="MEAS.DMM dual read") -> (w4432:T10)
        n1944 = Build Array(w4435, w4434, w4432, w4424) -> (w4430:T10[])
        n1945 = Reverse 1D Array(array=w4430) -> (reversed array=w4431:T10[])
        n1946 = for {
          tunnel: [w4458] -> w4443 mode=indexing
          tunnel: w4440 -> [w4457]
          tunnel: w4431 -> [w4456] mode=indexing
          n1947 = Unbundle By Name(w4456) -> ("command"=w4455:string, "command data"=w4454:variant)
          n1948 = call "App enquece.vi"("Priority Enquece"=TRUE, "command data"=w4454, "command"=w4455, "queue in"=w4457) -> ("error out"=w4458:errorcluster)  [unwired: 6 in, 1 out]
        }
        n1949 = Merge Errors(w4441, w4443) -> (w4442:errorcluster)
      }
      frame "Test DRV 51" {
        w4466 = 50  # DUT index(0-59)
        w4463 = T10 {"command"="", "command data"=variant} ("element")
        w4461 = "MEAS.mux6_1"
        n1950 = disable-structure shown="LOGGING==TRUE" {
          disable-tunnel: w4465 -> [w4487 _]
          frame condition #0 (active) {
            n1951 = Empty String/Path?(string/path=w4487) -> (empty?=w4490:bool)
            n1952 = Select(t="Quece timeout", s=w4490, f=w4487) -> (s? t:f=w4486:string)
            n1953 = call "string log (SubVI).vi"("Enum"=enum16{"Init", "Log", "Read"}."Log", "state Name"=w4486) -> ()  [unwired: 8 in, 2 out]
          }
          frame condition #1 {
          }
        }
        n1954 = To Variant(anything=T3."mux6-1_channel0" ("mux6_1(3wires)_encode")) -> (Variant=w4460:variant)
        n1955 = To Variant(anything=T3."mux6_1_channel3_3" ("mux6_1(3wires)_encode")) -> (Variant=w4476:variant)
        n1956 = To Variant(anything=T3."mux6_1_channel3_2" ("mux6_1(3wires)_encode")) -> (Variant=w4474:variant)
        n1957 = Bundle By Name(cluster=w4463, "command"=w4461, "command data"=w4474) -> (w4473:T10)
        n1958 = Bundle By Name(cluster=w4463, "command"=w4461, "command data"=w4476) -> (w4472:T10)
        n1959 = Bundle By Name(cluster=w4463, "command"=w4461, "command data"=w4460) -> (w4462:T10)
        n1960 = Bundle By Name(cluster=w4463, "command"="MEAS.DMM dual read") -> (w4470:T10)
        n1961 = Build Array(w4473, w4472, w4470, w4462) -> (w4468:T10[])
        n1962 = Reverse 1D Array(array=w4468) -> (reversed array=w4469:T10[])
        n1963 = for {
          tunnel: [w4496] -> w4481 mode=indexing
          tunnel: w4478 -> [w4495]
          tunnel: w4469 -> [w4494] mode=indexing
          n1964 = Unbundle By Name(w4494) -> ("command"=w4493:string, "command data"=w4492:variant)
          n1965 = call "App enquece.vi"("Priority Enquece"=TRUE, "command data"=w4492, "command"=w4493, "queue in"=w4495) -> ("error out"=w4496:errorcluster)  [unwired: 6 in, 1 out]
        }
        n1966 = Merge Errors(w4479, w4481) -> (w4480:errorcluster)
      }
      frame "Test DRV 52" {
        w4504 = 51  # DUT index(0-59)
        w4501 = T10 {"command"="", "command data"=variant} ("element")
        w4499 = "MEAS.mux6_1"
        n1967 = disable-structure shown="LOGGING==TRUE" {
          disable-tunnel: w4503 -> [w4525 _]
          frame condition #0 (active) {
            n1968 = Empty String/Path?(string/path=w4525) -> (empty?=w4528:bool)
            n1969 = Select(t="Quece timeout", s=w4528, f=w4525) -> (s? t:f=w4524:string)
            n1970 = call "string log (SubVI).vi"("Enum"=enum16{"Init", "Log", "Read"}."Log", "state Name"=w4524) -> ()  [unwired: 8 in, 2 out]
          }
          frame condition #1 {
          }
        }
        n1971 = To Variant(anything=T3."mux6-1_channel0" ("mux6_1(3wires)_encode")) -> (Variant=w4498:variant)
        n1972 = To Variant(anything=T3."mux6_1_channel4_3" ("mux6_1(3wires)_encode")) -> (Variant=w4514:variant)
        n1973 = To Variant(anything=T3."mux6_1_channel4_2" ("mux6_1(3wires)_encode")) -> (Variant=w4512:variant)
        n1974 = Bundle By Name(cluster=w4501, "command"=w4499, "command data"=w4512) -> (w4511:T10)
        n1975 = Bundle By Name(cluster=w4501, "command"=w4499, "command data"=w4514) -> (w4510:T10)
        n1976 = Bundle By Name(cluster=w4501, "command"=w4499, "command data"=w4498) -> (w4500:T10)
        n1977 = Bundle By Name(cluster=w4501, "command"="MEAS.DMM dual read") -> (w4508:T10)
        n1978 = Build Array(w4511, w4510, w4508, w4500) -> (w4506:T10[])
        n1979 = Reverse 1D Array(array=w4506) -> (reversed array=w4507:T10[])
        n1980 = for {
          tunnel: [w4534] -> w4519 mode=indexing
          tunnel: w4516 -> [w4533]
          tunnel: w4507 -> [w4532] mode=indexing
          n1981 = Unbundle By Name(w4532) -> ("command"=w4531:string, "command data"=w4530:variant)
          n1982 = call "App enquece.vi"("Priority Enquece"=TRUE, "command data"=w4530, "command"=w4531, "queue in"=w4533) -> ("error out"=w4534:errorcluster)  [unwired: 6 in, 1 out]
        }
        n1983 = Merge Errors(w4517, w4519) -> (w4518:errorcluster)
      }
      frame "Test DRV 53" {
        w4542 = 52  # DUT index(0-59)
        w4539 = T10 {"command"="", "command data"=variant} ("element")
        w4537 = "MEAS.mux6_1"
        n1984 = disable-structure shown="LOGGING==TRUE" {
          disable-tunnel: w4541 -> [w4563 _]
          frame condition #0 (active) {
            n1985 = Empty String/Path?(string/path=w4563) -> (empty?=w4566:bool)
            n1986 = Select(t="Quece timeout", s=w4566, f=w4563) -> (s? t:f=w4562:string)
            n1987 = call "string log (SubVI).vi"("Enum"=enum16{"Init", "Log", "Read"}."Log", "state Name"=w4562) -> ()  [unwired: 8 in, 2 out]
          }
          frame condition #1 {
          }
        }
        n1988 = To Variant(anything=T3."mux6-1_channel0" ("mux6_1(3wires)_encode")) -> (Variant=w4536:variant)
        n1989 = To Variant(anything=T3."mux6_1_channel5_3" ("mux6_1(3wires)_encode")) -> (Variant=w4552:variant)
        n1990 = To Variant(anything=T3."mux6_1_channel5_2" ("mux6_1(3wires)_encode")) -> (Variant=w4550:variant)
        n1991 = Bundle By Name(cluster=w4539, "command"=w4537, "command data"=w4550) -> (w4549:T10)
        n1992 = Bundle By Name(cluster=w4539, "command"=w4537, "command data"=w4552) -> (w4548:T10)
        n1993 = Bundle By Name(cluster=w4539, "command"=w4537, "command data"=w4536) -> (w4538:T10)
        n1994 = Bundle By Name(cluster=w4539, "command"="MEAS.DMM dual read") -> (w4546:T10)
        n1995 = Build Array(w4549, w4548, w4546, w4538) -> (w4544:T10[])
        n1996 = Reverse 1D Array(array=w4544) -> (reversed array=w4545:T10[])
        n1997 = for {
          tunnel: [w4572] -> w4557 mode=indexing
          tunnel: w4554 -> [w4571]
          tunnel: w4545 -> [w4570] mode=indexing
          n1998 = Unbundle By Name(w4570) -> ("command"=w4569:string, "command data"=w4568:variant)
          n1999 = call "App enquece.vi"("Priority Enquece"=TRUE, "command data"=w4568, "command"=w4569, "queue in"=w4571) -> ("error out"=w4572:errorcluster)  [unwired: 6 in, 1 out]
        }
        n2000 = Merge Errors(w4555, w4557) -> (w4556:errorcluster)
      }
      frame "Test DRV 54" {
        w4580 = 53  # DUT index(0-59)
        w4577 = T10 {"command"="", "command data"=variant} ("element")
        w4575 = "MEAS.mux6_1"
        n2001 = disable-structure shown="LOGGING==TRUE" {
          disable-tunnel: w4579 -> [w4601 _]
          frame condition #0 (active) {
            n2002 = Empty String/Path?(string/path=w4601) -> (empty?=w4604:bool)
            n2003 = Select(t="Quece timeout", s=w4604, f=w4601) -> (s? t:f=w4600:string)
            n2004 = call "string log (SubVI).vi"("Enum"=enum16{"Init", "Log", "Read"}."Log", "state Name"=w4600) -> ()  [unwired: 8 in, 2 out]
          }
          frame condition #1 {
          }
        }
        n2005 = To Variant(anything=T3."mux6-1_channel0" ("mux6_1(3wires)_encode")) -> (Variant=w4574:variant)
        n2006 = To Variant(anything=T3."mux6_1_channel6_3" ("mux6_1(3wires)_encode")) -> (Variant=w4590:variant)
        n2007 = To Variant(anything=T3."mux6_1_channel6_2" ("mux6_1(3wires)_encode")) -> (Variant=w4588:variant)
        n2008 = Bundle By Name(cluster=w4577, "command"=w4575, "command data"=w4588) -> (w4587:T10)
        n2009 = Bundle By Name(cluster=w4577, "command"=w4575, "command data"=w4590) -> (w4586:T10)
        n2010 = Bundle By Name(cluster=w4577, "command"=w4575, "command data"=w4574) -> (w4576:T10)
        n2011 = Bundle By Name(cluster=w4577, "command"="MEAS.DMM dual read") -> (w4584:T10)
        n2012 = Build Array(w4587, w4586, w4584, w4576) -> (w4582:T10[])
        n2013 = Reverse 1D Array(array=w4582) -> (reversed array=w4583:T10[])
        n2014 = for {
          tunnel: [w4610] -> w4595 mode=indexing
          tunnel: w4592 -> [w4609]
          tunnel: w4583 -> [w4608] mode=indexing
          n2015 = Unbundle By Name(w4608) -> ("command"=w4607:string, "command data"=w4606:variant)
          n2016 = call "App enquece.vi"("Priority Enquece"=TRUE, "command data"=w4606, "command"=w4607, "queue in"=w4609) -> ("error out"=w4610:errorcluster)  [unwired: 6 in, 1 out]
        }
        n2017 = Merge Errors(w4593, w4595) -> (w4594:errorcluster)
      }
      frame "Test DRV 55" {
        w4618 = 54  # DUT index(0-59)
        w4615 = T10 {"command"="", "command data"=variant} ("element")
        w4613 = "MEAS.mux6_1"
        n2018 = disable-structure shown="LOGGING==TRUE" {
          disable-tunnel: w4617 -> [w4639 _]
          frame condition #0 (active) {
            n2019 = Empty String/Path?(string/path=w4639) -> (empty?=w4642:bool)
            n2020 = Select(t="Quece timeout", s=w4642, f=w4639) -> (s? t:f=w4638:string)
            n2021 = call "string log (SubVI).vi"("Enum"=enum16{"Init", "Log", "Read"}."Log", "state Name"=w4638) -> ()  [unwired: 8 in, 2 out]
          }
          frame condition #1 {
          }
        }
        n2022 = To Variant(anything=T3."mux6-1_channel0" ("mux6_1(3wires)_encode")) -> (Variant=w4612:variant)
        n2023 = To Variant(anything=T3."mux6_1_channel1_3" ("mux6_1(3wires)_encode")) -> (Variant=w4628:variant)
        n2024 = To Variant(anything=T3."mux6-1_channel1_2" ("mux6_1(3wires)_encode")) -> (Variant=w4626:variant)
        n2025 = Bundle By Name(cluster=w4615, "command"=w4613, "command data"=w4626) -> (w4625:T10)
        n2026 = Bundle By Name(cluster=w4615, "command"=w4613, "command data"=w4628) -> (w4624:T10)
        n2027 = Bundle By Name(cluster=w4615, "command"=w4613, "command data"=w4612) -> (w4614:T10)
        n2028 = Bundle By Name(cluster=w4615, "command"="MEAS.DMM dual read") -> (w4622:T10)
        n2029 = Build Array(w4625, w4624, w4622, w4614) -> (w4620:T10[])
        n2030 = Reverse 1D Array(array=w4620) -> (reversed array=w4621:T10[])
        n2031 = for {
          tunnel: [w4648] -> w4633 mode=indexing
          tunnel: w4630 -> [w4647]
          tunnel: w4621 -> [w4646] mode=indexing
          n2032 = Unbundle By Name(w4646) -> ("command"=w4645:string, "command data"=w4644:variant)
          n2033 = call "App enquece.vi"("Priority Enquece"=TRUE, "command data"=w4644, "command"=w4645, "queue in"=w4647) -> ("error out"=w4648:errorcluster)  [unwired: 6 in, 1 out]
        }
        n2034 = Merge Errors(w4631, w4633) -> (w4632:errorcluster)
      }
      frame "Test DRV 56" {
        w4656 = 55  # DUT index(0-59)
        w4653 = T10 {"command"="", "command data"=variant} ("element")
        w4651 = "MEAS.mux6_1"
        n2035 = disable-structure shown="LOGGING==TRUE" {
          disable-tunnel: w4655 -> [w4677 _]
          frame condition #0 (active) {
            n2036 = Empty String/Path?(string/path=w4677) -> (empty?=w4680:bool)
            n2037 = Select(t="Quece timeout", s=w4680, f=w4677) -> (s? t:f=w4676:string)
            n2038 = call "string log (SubVI).vi"("Enum"=enum16{"Init", "Log", "Read"}."Log", "state Name"=w4676) -> ()  [unwired: 8 in, 2 out]
          }
          frame condition #1 {
          }
        }
        n2039 = To Variant(anything=T3."mux6-1_channel0" ("mux6_1(3wires)_encode")) -> (Variant=w4650:variant)
        n2040 = To Variant(anything=T3."mux6_1_channel2_3" ("mux6_1(3wires)_encode")) -> (Variant=w4666:variant)
        n2041 = To Variant(anything=T3."mux6_1_channel2_2" ("mux6_1(3wires)_encode")) -> (Variant=w4664:variant)
        n2042 = Bundle By Name(cluster=w4653, "command"=w4651, "command data"=w4664) -> (w4663:T10)
        n2043 = Bundle By Name(cluster=w4653, "command"=w4651, "command data"=w4666) -> (w4662:T10)
        n2044 = Bundle By Name(cluster=w4653, "command"=w4651, "command data"=w4650) -> (w4652:T10)
        n2045 = Bundle By Name(cluster=w4653, "command"="MEAS.DMM dual read") -> (w4660:T10)
        n2046 = Build Array(w4663, w4662, w4660, w4652) -> (w4658:T10[])
        n2047 = Reverse 1D Array(array=w4658) -> (reversed array=w4659:T10[])
        n2048 = for {
          tunnel: [w4686] -> w4671 mode=indexing
          tunnel: w4668 -> [w4685]
          tunnel: w4659 -> [w4684] mode=indexing
          n2049 = Unbundle By Name(w4684) -> ("command"=w4683:string, "command data"=w4682:variant)
          n2050 = call "App enquece.vi"("Priority Enquece"=TRUE, "command data"=w4682, "command"=w4683, "queue in"=w4685) -> ("error out"=w4686:errorcluster)  [unwired: 6 in, 1 out]
        }
        n2051 = Merge Errors(w4669, w4671) -> (w4670:errorcluster)
      }
      frame "Test DRV 57" {
        w4694 = 56  # DUT index(0-59)
        w4691 = T10 {"command"="", "command data"=variant} ("element")
        w4689 = "MEAS.mux6_1"
        n2052 = disable-structure shown="LOGGING==TRUE" {
          disable-tunnel: w4693 -> [w4715 _]
          frame condition #0 (active) {
            n2053 = Empty String/Path?(string/path=w4715) -> (empty?=w4718:bool)
            n2054 = Select(t="Quece timeout", s=w4718, f=w4715) -> (s? t:f=w4714:string)
            n2055 = call "string log (SubVI).vi"("Enum"=enum16{"Init", "Log", "Read"}."Log", "state Name"=w4714) -> ()  [unwired: 8 in, 2 out]
          }
          frame condition #1 {
          }
        }
        n2056 = To Variant(anything=T3."mux6-1_channel0" ("mux6_1(3wires)_encode")) -> (Variant=w4688:variant)
        n2057 = To Variant(anything=T3."mux6_1_channel3_3" ("mux6_1(3wires)_encode")) -> (Variant=w4704:variant)
        n2058 = To Variant(anything=T3."mux6_1_channel3_2" ("mux6_1(3wires)_encode")) -> (Variant=w4702:variant)
        n2059 = Bundle By Name(cluster=w4691, "command"=w4689, "command data"=w4702) -> (w4701:T10)
        n2060 = Bundle By Name(cluster=w4691, "command"=w4689, "command data"=w4704) -> (w4700:T10)
        n2061 = Bundle By Name(cluster=w4691, "command"=w4689, "command data"=w4688) -> (w4690:T10)
        n2062 = Bundle By Name(cluster=w4691, "command"="MEAS.DMM dual read") -> (w4698:T10)
        n2063 = Build Array(w4701, w4700, w4698, w4690) -> (w4696:T10[])
        n2064 = Reverse 1D Array(array=w4696) -> (reversed array=w4697:T10[])
        n2065 = for {
          tunnel: [w4724] -> w4709 mode=indexing
          tunnel: w4706 -> [w4723]
          tunnel: w4697 -> [w4722] mode=indexing
          n2066 = Unbundle By Name(w4722) -> ("command"=w4721:string, "command data"=w4720:variant)
          n2067 = call "App enquece.vi"("Priority Enquece"=TRUE, "command data"=w4720, "command"=w4721, "queue in"=w4723) -> ("error out"=w4724:errorcluster)  [unwired: 6 in, 1 out]
        }
        n2068 = Merge Errors(w4707, w4709) -> (w4708:errorcluster)
      }
      frame "Test DRV 58" {
        w4732 = 57  # DUT index(0-59)
        w4729 = T10 {"command"="", "command data"=variant} ("element")
        w4727 = "MEAS.mux6_1"
        n2069 = disable-structure shown="LOGGING==TRUE" {
          disable-tunnel: w4731 -> [w4753 _]
          frame condition #0 (active) {
            n2070 = Empty String/Path?(string/path=w4753) -> (empty?=w4756:bool)
            n2071 = Select(t="Quece timeout", s=w4756, f=w4753) -> (s? t:f=w4752:string)
            n2072 = call "string log (SubVI).vi"("Enum"=enum16{"Init", "Log", "Read"}."Log", "state Name"=w4752) -> ()  [unwired: 8 in, 2 out]
          }
          frame condition #1 {
          }
        }
        n2073 = To Variant(anything=T3."mux6-1_channel0" ("mux6_1(3wires)_encode")) -> (Variant=w4726:variant)
        n2074 = To Variant(anything=T3."mux6_1_channel4_3" ("mux6_1(3wires)_encode")) -> (Variant=w4742:variant)
        n2075 = To Variant(anything=T3."mux6_1_channel4_2" ("mux6_1(3wires)_encode")) -> (Variant=w4740:variant)
        n2076 = Bundle By Name(cluster=w4729, "command"=w4727, "command data"=w4740) -> (w4739:T10)
        n2077 = Bundle By Name(cluster=w4729, "command"=w4727, "command data"=w4742) -> (w4738:T10)
        n2078 = Bundle By Name(cluster=w4729, "command"=w4727, "command data"=w4726) -> (w4728:T10)
        n2079 = Bundle By Name(cluster=w4729, "command"="MEAS.DMM dual read") -> (w4736:T10)
        n2080 = Build Array(w4739, w4738, w4736, w4728) -> (w4734:T10[])
        n2081 = Reverse 1D Array(array=w4734) -> (reversed array=w4735:T10[])
        n2082 = for {
          tunnel: [w4762] -> w4747 mode=indexing
          tunnel: w4744 -> [w4761]
          tunnel: w4735 -> [w4760] mode=indexing
          n2083 = Unbundle By Name(w4760) -> ("command"=w4759:string, "command data"=w4758:variant)
          n2084 = call "App enquece.vi"("Priority Enquece"=TRUE, "command data"=w4758, "command"=w4759, "queue in"=w4761) -> ("error out"=w4762:errorcluster)  [unwired: 6 in, 1 out]
        }
        n2085 = Merge Errors(w4745, w4747) -> (w4746:errorcluster)
      }
      frame "Test DRV 59" {
        w4770 = 58  # DUT index(0-59)
        w4767 = T10 {"command"="", "command data"=variant} ("element")
        w4765 = "MEAS.mux6_1"
        n2086 = disable-structure shown="LOGGING==TRUE" {
          disable-tunnel: w4769 -> [w4791 _]
          frame condition #0 (active) {
            n2087 = Empty String/Path?(string/path=w4791) -> (empty?=w4794:bool)
            n2088 = Select(t="Quece timeout", s=w4794, f=w4791) -> (s? t:f=w4790:string)
            n2089 = call "string log (SubVI).vi"("Enum"=enum16{"Init", "Log", "Read"}."Log", "state Name"=w4790) -> ()  [unwired: 8 in, 2 out]
          }
          frame condition #1 {
          }
        }
        n2090 = To Variant(anything=T3."mux6-1_channel0" ("mux6_1(3wires)_encode")) -> (Variant=w4764:variant)
        n2091 = To Variant(anything=T3."mux6_1_channel5_3" ("mux6_1(3wires)_encode")) -> (Variant=w4780:variant)
        n2092 = To Variant(anything=T3."mux6_1_channel5_2" ("mux6_1(3wires)_encode")) -> (Variant=w4778:variant)
        n2093 = Bundle By Name(cluster=w4767, "command"=w4765, "command data"=w4778) -> (w4777:T10)
        n2094 = Bundle By Name(cluster=w4767, "command"=w4765, "command data"=w4780) -> (w4776:T10)
        n2095 = Bundle By Name(cluster=w4767, "command"=w4765, "command data"=w4764) -> (w4766:T10)
        n2096 = Bundle By Name(cluster=w4767, "command"="MEAS.DMM dual read") -> (w4774:T10)
        n2097 = Build Array(w4777, w4776, w4774, w4766) -> (w4772:T10[])
        n2098 = Reverse 1D Array(array=w4772) -> (reversed array=w4773:T10[])
        n2099 = for {
          tunnel: [w4800] -> w4785 mode=indexing
          tunnel: w4782 -> [w4799]
          tunnel: w4773 -> [w4798] mode=indexing
          n2100 = Unbundle By Name(w4798) -> ("command"=w4797:string, "command data"=w4796:variant)
          n2101 = call "App enquece.vi"("Priority Enquece"=TRUE, "command data"=w4796, "command"=w4797, "queue in"=w4799) -> ("error out"=w4800:errorcluster)  [unwired: 6 in, 1 out]
        }
        n2102 = Merge Errors(w4783, w4785) -> (w4784:errorcluster)
      }
      frame "Test DRV 60" {
        w4808 = 59  # DUT index(0-59)
        w4805 = T10 {"command"="", "command data"=variant} ("element")
        w4803 = "MEAS.mux6_1"
        n2103 = disable-structure shown="LOGGING==TRUE" {
          disable-tunnel: w4807 -> [w4829 _]
          frame condition #0 (active) {
            n2104 = Empty String/Path?(string/path=w4829) -> (empty?=w4832:bool)
            n2105 = Select(t="Quece timeout", s=w4832, f=w4829) -> (s? t:f=w4828:string)
            n2106 = call "string log (SubVI).vi"("Enum"=enum16{"Init", "Log", "Read"}."Log", "state Name"=w4828) -> ()  [unwired: 8 in, 2 out]
          }
          frame condition #1 {
          }
        }
        n2107 = To Variant(anything=T3."mux6-1_channel0" ("mux6_1(3wires)_encode")) -> (Variant=w4802:variant)
        n2108 = To Variant(anything=T3."mux6_1_channel6_3" ("mux6_1(3wires)_encode")) -> (Variant=w4818:variant)
        n2109 = To Variant(anything=T3."mux6_1_channel6_2" ("mux6_1(3wires)_encode")) -> (Variant=w4816:variant)
        n2110 = Bundle By Name(cluster=w4805, "command"=w4803, "command data"=w4816) -> (w4815:T10)
        n2111 = Bundle By Name(cluster=w4805, "command"=w4803, "command data"=w4818) -> (w4814:T10)
        n2112 = Bundle By Name(cluster=w4805, "command"=w4803, "command data"=w4802) -> (w4804:T10)
        n2113 = Bundle By Name(cluster=w4805, "command"="MEAS.DMM dual read") -> (w4812:T10)
        n2114 = Build Array(w4815, w4814, w4812, w4804) -> (w4810:T10[])
        n2115 = Reverse 1D Array(array=w4810) -> (reversed array=w4811:T10[])
        n2116 = for {
          tunnel: [w4838] -> w4823 mode=indexing
          tunnel: w4820 -> [w4837]
          tunnel: w4811 -> [w4836] mode=indexing
          n2117 = Unbundle By Name(w4836) -> ("command"=w4835:string, "command data"=w4834:variant)
          n2118 = call "App enquece.vi"("Priority Enquece"=TRUE, "command data"=w4834, "command"=w4835, "queue in"=w4837) -> ("error out"=w4838:errorcluster)  [unwired: 6 in, 1 out]
        }
        n2119 = Merge Errors(w4821, w4823) -> (w4822:errorcluster)
      }
      frame "separated" {
      }
    }
    "DC Measure Completed" <- w136
    "Progress" <- w133
    n2120 = feedback-in #1(w133) -> ()
    n2121 = disable-structure shown="LOGGING==TRUE" {
      disable-tunnel: [w160 _] -> w134
      disable-tunnel: w135 -> [w157 _]
      frame condition #0 (active) {
        n2122 = property on="State log" class="Str"("Text.Scroll Position"=inf) -> ()  [unwired: 2 in, 2 out]
        n2123 = call "string log (SubVI).vi"("error in (no error)"=w157, "Enum"=enum16{"Init", "Log", "Read"}."Read") -> ("error out"=w160:errorcluster, "State log"=→"State log":string)  [unwired: 8 in]
      }
      frame condition #1 {
      }
    }
  }
  n2124 = property on="State log" class="Str"("Text.Scroll Position"=inf) -> ()  [unwired: 2 in, 2 out]
  n2125 = Unregister For Events(event registration refnum=w90) -> (error out=w6:errorcluster)  [unwired: 1 in]
  n2126 = Release Queue(queue=w86, error in (no error)=w85) -> (error out=w4:errorcluster)  [unwired: 1 in, 2 out]
  n2127 = Destroy User Event(user event=w3, error in=w4) -> (error out=w2:errorcluster)
  n2128 = Merge Errors(w6, w2) -> (w5:errorcluster)
  n2129 = disable-structure shown="RUN_TIME_ENGINE==True" {
    disable-tunnel: w5 -> [w4847 _]
    frame condition #0 (active) {
      "error out" <- w4847
    }
    frame condition #1 {
      n2130 = Quit LabVIEW(quit? (T)=TRUE) -> ()
    }
  }
